vi "数据编码.vi"(0 "table输入":string(combo), 5 "错误常量 2":errorcluster caption="错误输入", 9 "QN":string, 13 "MN":string, 14 "PW":string) -> (4 "错误常量":errorcluster caption="错误输出", 8 "数据区":string, 15 "通讯包字符串":string)   [LabVIEW 2016]
uses:
  <vilib>/ptbypt/NI_PtbyPt.lvlib
panel:
  in  "时间戳 2":string
  in  "时间戳":string
  out "总包数":i32
  out "包数":i32=1024
  out "核查数据发送次数":i32
  out "当前包数":i32
  out "总包数":string
  out "小时数据发送次数":i32
  out "长度":i32
  in  "数据块":T1
  out "通讯包":T2={"包头（2）"="##", "数据段长度（4）"="", "数据段"="", "CRC校验"="", "包尾"=""}
  # "范例代码：\n\n##0101QN=20160801085857223;ST=32;CN=1062;PW=100000;MN=010000A8900016F000169DC0;Flag=5\n;CP=&&RtdInterval=30&&1C80\\r\\n"
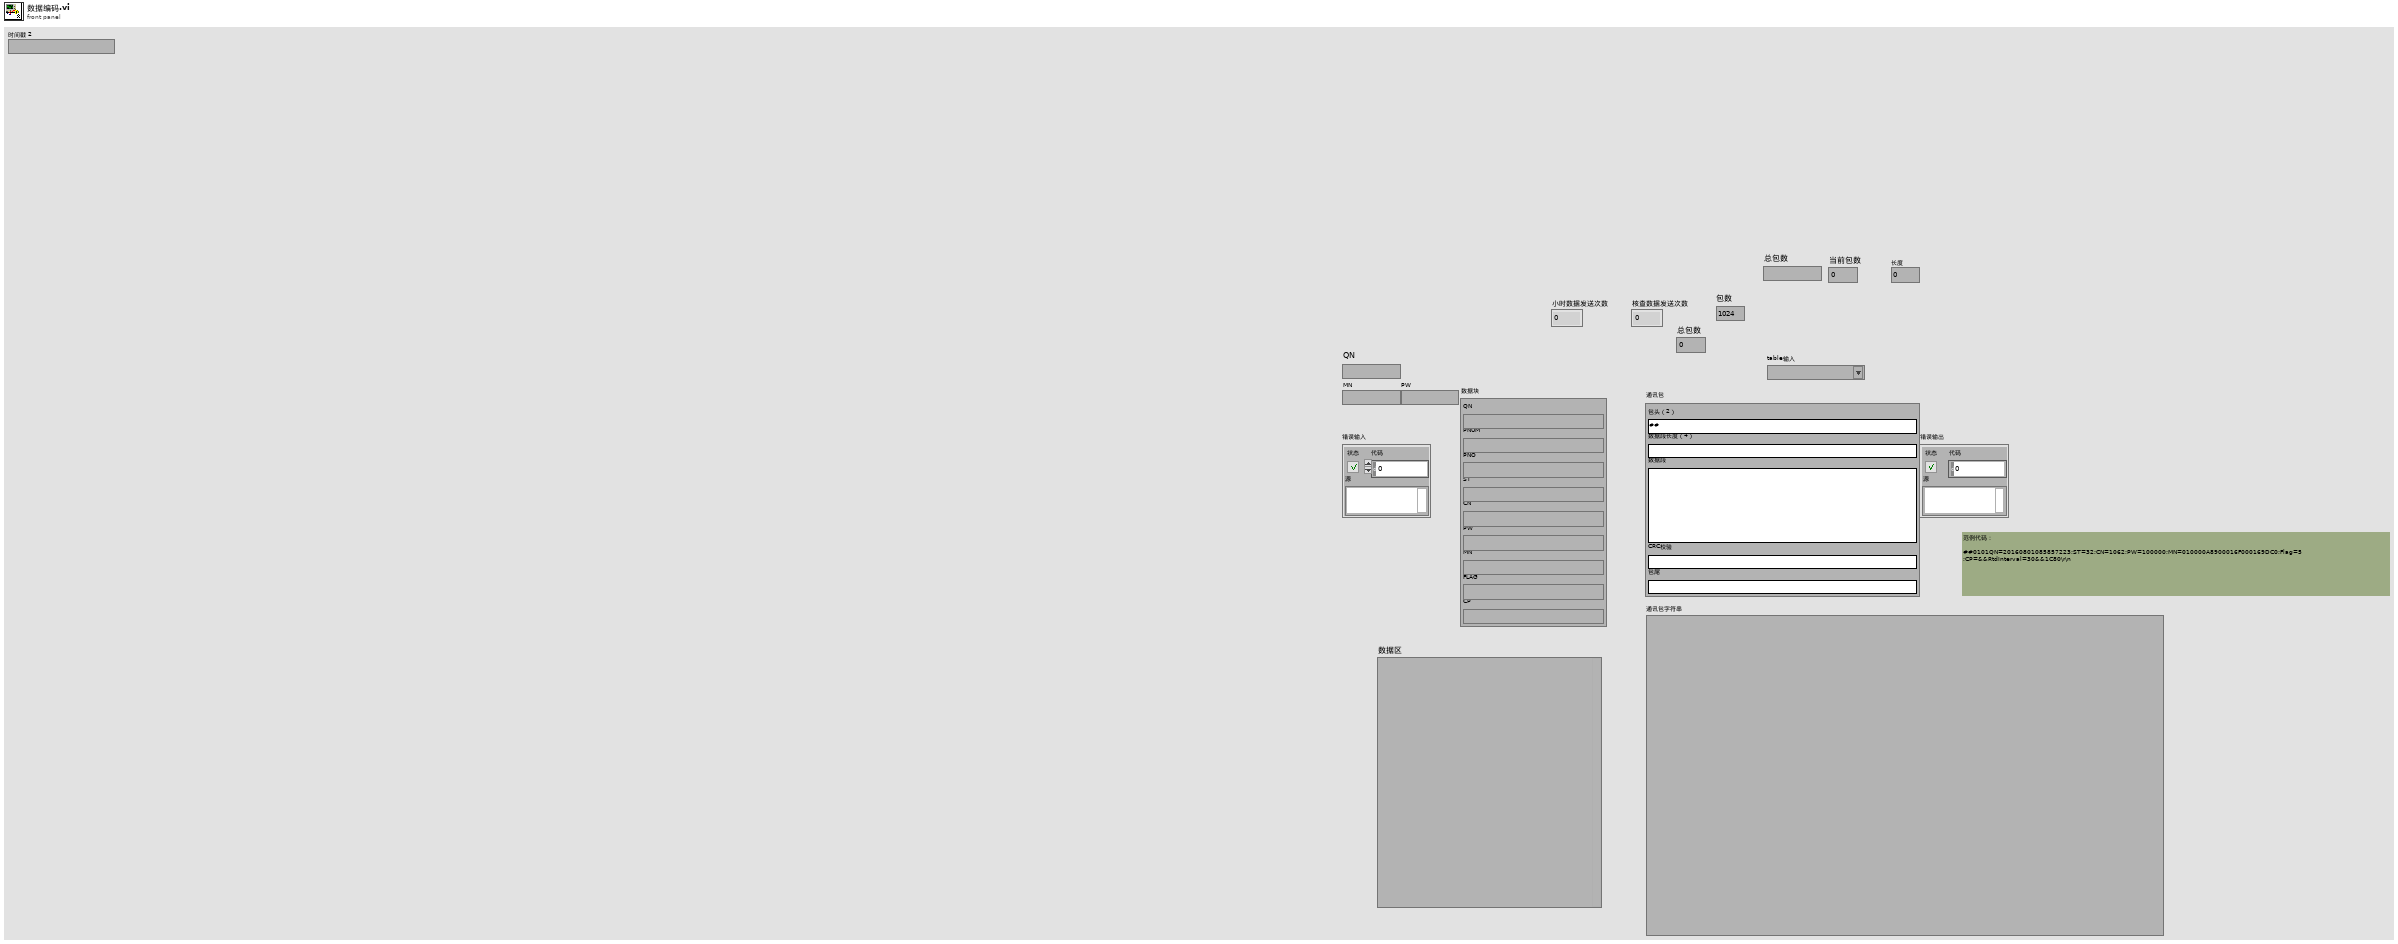
[diagram p1: front panel]
types:
  T1 = cluster{"QN":string, "ST":string, "CN":string, "PW":string, "MN":string, "FLAG":string, "PNUM":string, "PNO":string, "CP":string}
  T2 = cluster{"包头（2）":string, "数据段长度（4）":string, "数据段":string, "CRC校验":string, "包尾":string}
  T3 = cluster{"PH":string[][], "CODCr":string[][], "氨氮":string[][], "CODMn":string[][], "总氮":string[][], "总磷":string[][], "电导率":string[][], "水温":string[][], "DO":string[][], "浊度":string[][], "叶绿素":string[][], "藻密度":string[][]}
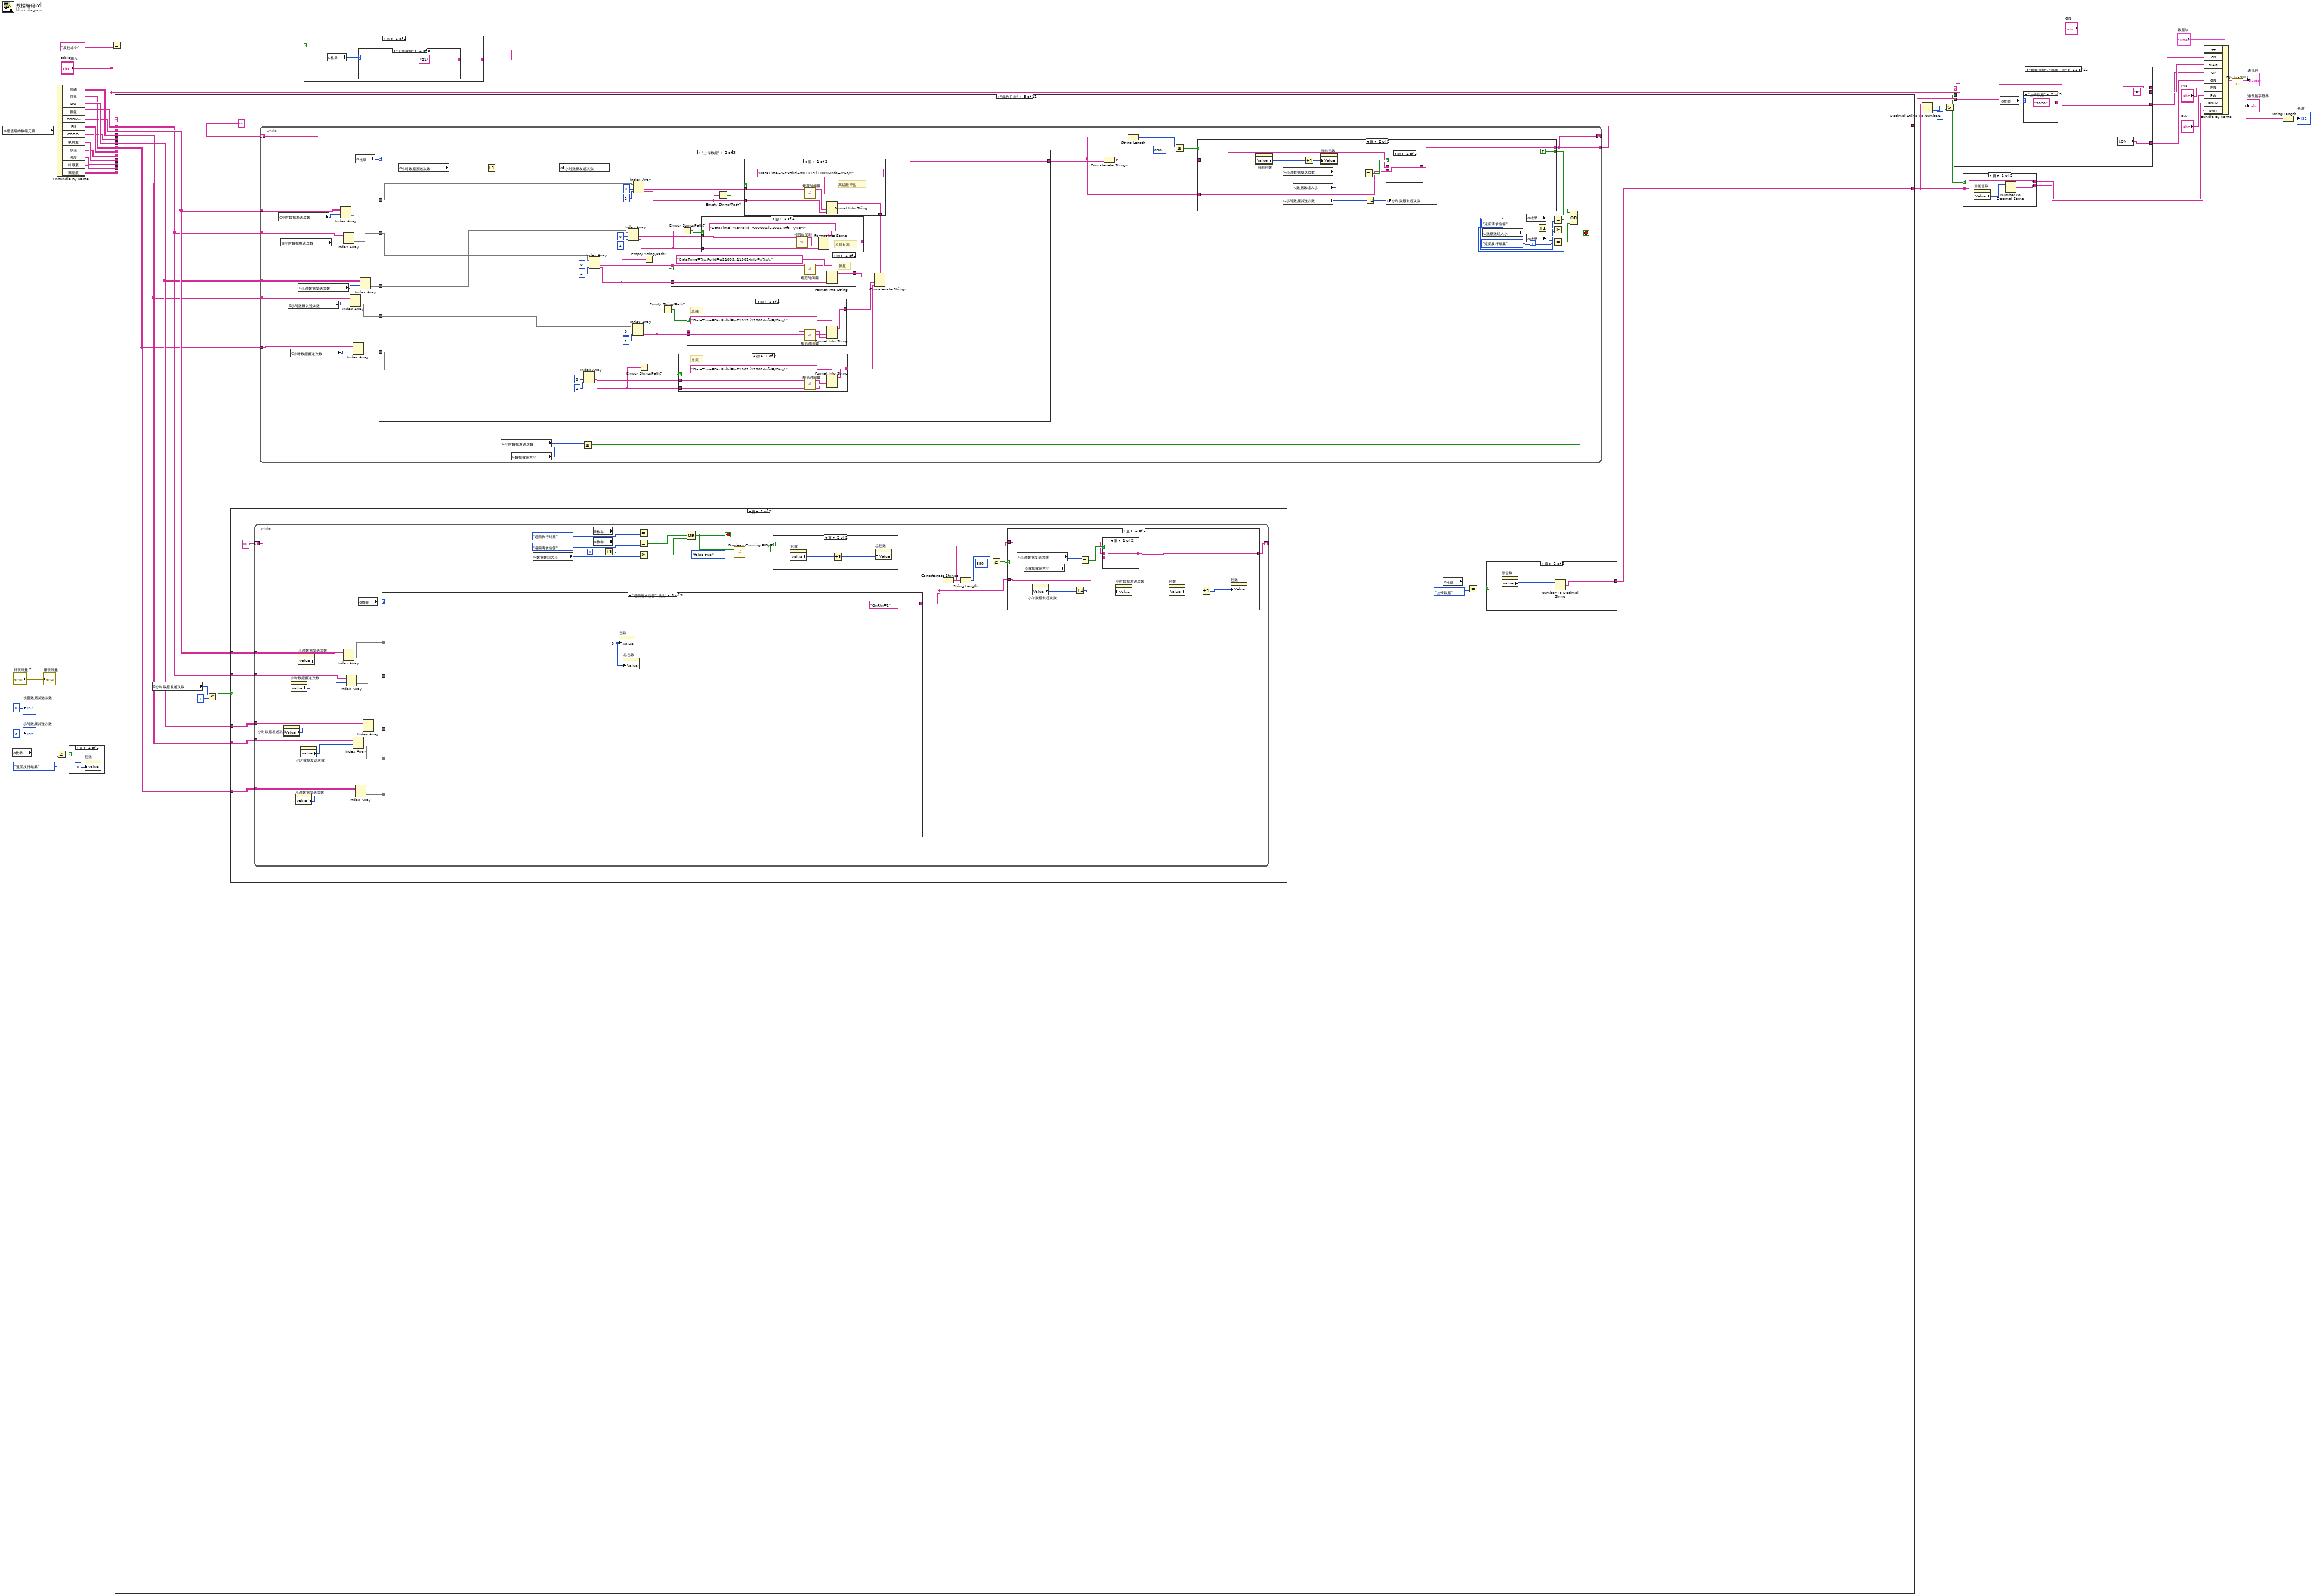
[diagram p0: block diagram]
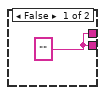
[diagram p3: hidden frame]
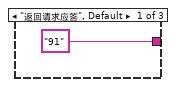
[diagram p4: hidden frame]
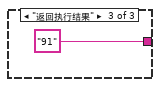
[diagram p5: hidden frame]
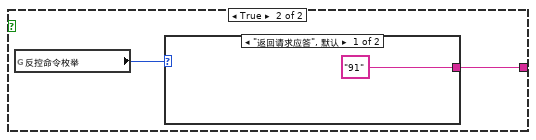
[diagram p6: hidden frame]
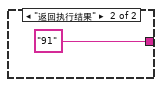
[diagram p7: hidden frame]
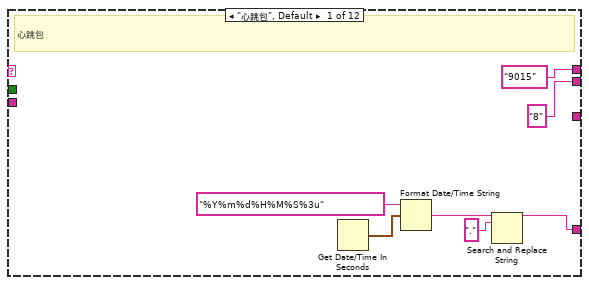
[diagram p8: hidden frame]
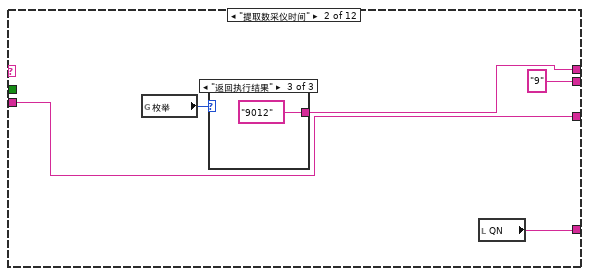
[diagram p9: hidden frame]
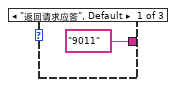
[diagram p10: hidden frame]
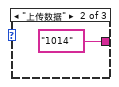
[diagram p11: hidden frame]
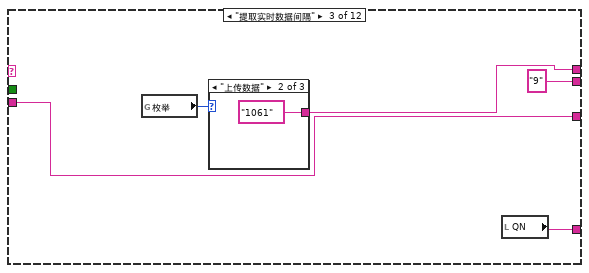
[diagram p12: hidden frame]
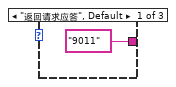
[diagram p13: hidden frame]
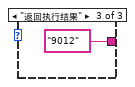
[diagram p14: hidden frame]
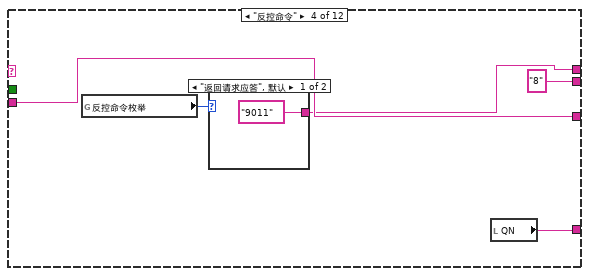
[diagram p15: hidden frame]
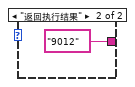
[diagram p16: hidden frame]
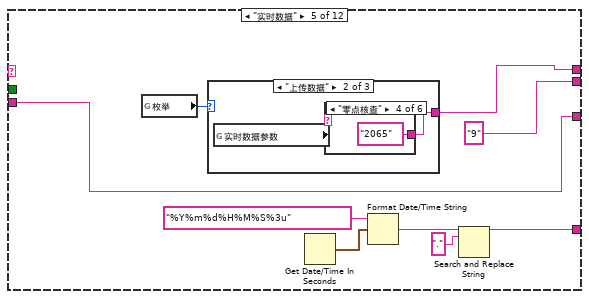
[diagram p17: hidden frame]
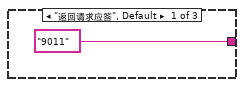
[diagram p18: hidden frame]
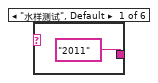
[diagram p19: hidden frame]
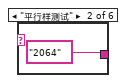
[diagram p20: hidden frame]
diagram:
  n1 = global read "插值后的新数组.vi" "插值后的数组元素"() -> (w9:T3)
  n2 = global read "全局1.vi" "枚举"() -> (w17:enum16{"返回请求应答", "上传数据", "返回执行结果"})
  n3 = Not Equal?(x=w17, y=enum16{"返回请求应答", "上传数据", "返回执行结果"}."返回执行结果") -> (x != y?=w15:bool)
  n4 = Unbundle By Name(w9) -> ("总磷"=w25:string[][], "总氮"=w24:string[][], "DO"=w26:string[][], "氨氮"=w27:string[][], "CODMn"=w8:string[][], "PH"=w12:string[][], "CODCr"=w11:string[][], "电导率"=w7:string[][], "水温"=w6:string[][], "浊度"=w5:string[][], "叶绿素"=w4:string[][], "藻密度"=w3:string[][])
  n5 = case shown="真" w15 {
    frame False {
    }
    frame True {
      n6 = property on="包数" class="DigNum (严格)"("Value"=0 ("总包数")) -> ()  [unwired: 2 in, 2 out]
    }
  }
  n7 = Equal?(x="table输入", y="反控命令") -> (x = y?=w29:bool)
  n8 = case shown="\"操作日志\"" "table输入" {
    tunnel: [w44 _ w48 w58 w67 w591 w985 w1448 w1880 w2166 w2437] -> w10
    tunnel: w8 -> [_ _ _ _ _ w589 w983 w1457 w1879 w2165 _]
    tunnel: w27 -> [_ _ _ _ _ w588 w982 w1456 w1878 w2164 _]
    tunnel: w26 -> [_ _ _ _ _ w587 w981 w1455 w1877 w2163 _]
    tunnel: w25 -> [_ _ _ _ _ w586 w980 w1454 w1876 w2162 _]
    tunnel: w24 -> [_ _ _ _ _ w585 w979 w1453 w1875 w2161 _]
    tunnel: [_ _ "" "" _ w558 w952 w1447 w1871 w2156 _] -> w14
    tunnel: w12 -> [_ _ _ _ _ w579 w973 w1445 _ _ _]
    tunnel: w11 -> [_ _ _ _ _ w578 w972 w1444 _ _ _]
    tunnel: w7 -> [_ _ _ _ _ w577 w971 _ _ _ _]
    tunnel: w6 -> [_ _ _ _ _ w576 w970 _ _ _ _]
    tunnel: w5 -> [_ _ _ _ _ w575 w969 _ _ _ _]
    tunnel: w4 -> [_ _ _ _ _ w574 w968 _ _ _ _]
    tunnel: w3 -> [_ _ _ _ _ w573 w967 _ _ _ _]
    frame "反控命令" {
      n9 = global read "全局 反控命令枚举.vi" "反控命令枚举"() -> (w43:enum16{"返回请求应答", "返回执行结果"})
      n10 = case shown="\"返回执行结果\"" w43 {
        tunnel: ["QnRtn=1" "ExeRtn=1"] -> w44
        frame "返回请求应答", Default {
        }
        frame "返回执行结果" {
        }
      }
    }
    frame "心跳包", Default {
    }
    frame "提取数采仪时间" {
      n11 = global read "全局1.vi" "枚举"() -> (w49:enum16{"返回请求应答", "上传数据", "返回执行结果"})
      n12 = case shown="\"上传数据\"" w49 {
        tunnel: ["QnRtn=1" w51 "ExeRtn=1"] -> w48
        frame "返回请求应答", Default {
        }
        frame "上传数据" {
          n13 = Get Date/Time In Seconds() -> (seconds since 1Jan1904=w55:timestamp)
          n14 = Format Date/Time String(time format string (%c)="%Y%m%d%H%M%S" ("时间格式字符串(%c)"), seconds (now)=w55) -> (date/time string=w52:string)  [unwired: 1 in]
          n15 = Concatenate Strings("SystemTime=", w52) -> (w51:string)
        }
        frame "返回执行结果" {
        }
      }
    }
    frame "提取实时数据间隔" {
      n16 = global read "全局1.vi" "枚举"() -> (w59:enum16{"返回请求应答", "上传数据", "返回执行结果"})
      n17 = case shown="\"上传数据\"" w59 {
        tunnel: ["QnRtn=1" w63 "ExeRtn=1"] -> w58
        frame "返回请求应答", Default {
        }
        frame "上传数据" {
          n18 = global read "实时数据发送间隔全局.vi" "实时数据发送间隔"() -> (w62:u32)
          n19 = Number To Decimal String(number=w62) -> (decimal integer string=w61:string)  [unwired: 1 in]
          n20 = Concatenate Strings("RtdInterval=", w61) -> (w63:string)
        }
        frame "返回执行结果" {
        }
      }
    }
    frame "实时数据" {
      n21 = global read "全局 实时数据参数.vi" "实时数据参数"() -> (w66:string)
      n22 = case shown="\"水样测试\", 默认" w66 {
        tunnel: [w68 w194 w321 w447] -> w67
        frame "水样测试", Default {
          n23 = global read "全局1.vi" "枚举"() -> (w69:enum16{"返回请求应答", "上传数据", "返回执行结果"})
          n24 = case shown="\"上传数据\"" w69 {
            tunnel: ["QnRtn=1" w75 "ExeRtn=1"] -> w68
            frame "返回请求应答", Default {
            }
            frame "上传数据" {
              n25 = control-ref of="时间戳"() -> (w73:refnum<vi>)
              n26 = Empty String/Path?(string/path="时间戳") -> (empty?=w72:bool)
              n27 = call "实时数据时间戳 (子VI).vi"("String输入"=w73) -> ()  [unwired: 11 in]
              n28 = Not(x=w72) -> (.not. x?=w71:bool)
              n29 = case shown="真" w71 {
                tunnel: ["" w190] -> w75
                tunnel: "时间戳" -> [_ w189]
                frame False {
                }
                frame True {
                  # "CODCr"
                  # "总氮"
                  # "总磷"
                  # "叶绿素"
                  # "叶绿素"
                  # "浊度"
                  # "电导率"
                  # "DO"
                  # "PH"
                  # "水温"
                  # "NH3"
                  # "CODMn"
                  n30 = global read "全局 所有参数.vi" "CODMn"() -> (w173:string[][])
                  n31 = global read "全局 所有参数.vi" "氨氮"() -> (w178:string[][])
                  n32 = global read "全局 所有参数.vi" "水温"() -> (w166:string[][])
                  n33 = global read "全局 所有参数.vi" "电导率"() -> (w138:string[][])
                  n34 = global read "全局 所有参数.vi" "DO"() -> (w148:string[][])
                  n35 = global read "全局 所有参数.vi" "PH"() -> (w156:string[][])
                  n36 = global read "全局 所有参数.vi" "藻密度"() -> (w111:string[][])
                  n37 = global read "全局 所有参数.vi" "浊度"() -> (w130:string[][])
                  n38 = global read "全局 所有参数.vi" "叶绿素"() -> (w121:string[][])
                  n39 = global read "全局 所有参数.vi" "CODCr"() -> (w83:string[][])
                  n40 = global read "全局 所有参数.vi" "总磷"() -> (w103:string[][])
                  n41 = global read "全局 所有参数.vi" "总氮"() -> (w91:string[][])
                  n42 = Index Array(array=w178, index (row)=0 ("索引 (行)")) -> (element=w176:string[])  [unwired: 1 in]
                  n43 = call "规范小时时间戳.vi"("字符串"=w189) -> ("result string"=w192:string)  [unwired: 10 in]
                  n44 = Index Array(array=w166, index (row)=0 ("索引 (行)")) -> (element=w168:string[])  [unwired: 1 in]
                  n45 = Index Array(array=w148, index (row)=0 ("索引 (行)")) -> (element=w150:string[])  [unwired: 1 in]
                  n46 = Index Array(array=w156, index (row)=0 ("索引 (行)")) -> (element=w154:string[])  [unwired: 1 in]
                  n47 = Index Array(array=w138, index (row)=0 ("索引 (行)")) -> (element=w136:string[])  [unwired: 1 in]
                  n48 = Index Array(array=w173, index (row)=0 ("索引 (行)")) -> (element=w171:string[])  [unwired: 1 in]
                  n49 = Index Array(array=w130, index (row)=0 ("索引 (行)")) -> (element=w132:string[])  [unwired: 1 in]
                  n50 = Index Array(array=w111, index (row)=0 ("索引 (行)")) -> (element=w109:string[])  [unwired: 1 in]
                  n51 = Index Array(array=w121, index (row)=0 ("索引 (行)")) -> (element=w123:string[])  [unwired: 1 in]
                  n52 = Index Array(array=w103, index (row)=0 ("索引 (行)")) -> (element=w105:string[])  [unwired: 1 in]
                  n53 = Index Array(array=w176, index=3 ("索引")) -> (element=w175:string)
                  n54 = Index Array(array=w91, index (row)=0 ("索引 (行)")) -> (element=w89:string[])  [unwired: 1 in]
                  n55 = Index Array(array=w83, index (row)=0 ("索引 (行)")) -> (element=w85:string[])  [unwired: 1 in]
                  n56 = Index Array(array=w168, index=3 ("索引")) -> (element=w169:string)
                  n57 = Index Array(array=w150, index=3 ("索引")) -> (element=w151:string)
                  n58 = Index Array(array=w154, index=3 ("索引")) -> (element=w153:string)
                  n59 = Index Array(array=w136, index=3 ("索引")) -> (element=w135:string)
                  n60 = Index Array(array=w132, index=3 ("索引")) -> (element=w133:string)
                  n61 = Index Array(array=w171, index=3 ("索引")) -> (element=w170:string)
                  n62 = Index Array(array=w109, index=3 ("索引")) -> (element=w108:string)
                  n63 = Index Array(array=w123, index=3 ("索引")) -> (element=w124:string)
                  n64 = Index Array(array=w105, index=3 ("索引")) -> (element=w106:string)
                  n65 = Index Array(array=w89, index=3 ("索引")) -> (element=w88:string)
                  n66 = Index Array(array=w85, index=3 ("索引")) -> (element=w86:string)
                  n67 = call "数据编码整合输出.vi"("数据标识"="N" ("字符串"), "数据类型"="-Rtd=", "污染物编码"="w21003", "数据精度"=3 ("精度"), "数据值"=w175) -> ("编码输出"=w180:string)  [unwired: 6 in]
                  n68 = call "数据编码整合输出.vi"("数据标识"="N" ("字符串"), "数据类型"="-Rtd=", "污染物编码"="w01010", "数据值"=w169) -> ("编码输出"=w161:string)  [unwired: 7 in]
                  n69 = call "数据编码整合输出.vi"("数据标识"="N" ("字符串"), "数据类型"="-Rtd=", "污染物编码"="w01009", "数据值"=w151) -> ("编码输出"=w143:string)  [unwired: 7 in]
                  n70 = call "数据编码整合输出.vi"("数据标识"="N" ("字符串"), "数据类型"="-Rtd=", "污染物编码"="w01001", "数据值"=w153) -> ("编码输出"=w152:string)  [unwired: 7 in]
                  n71 = call "数据编码整合输出.vi"("数据标识"="N" ("字符串"), "数据类型"="-Rtd=", "污染物编码"="w01014", "数据值"=w135) -> ("编码输出"=w134:string)  [unwired: 7 in]
                  n72 = call "数据编码整合输出.vi"("数据标识"="N" ("字符串"), "数据类型"="-Rtd=", "污染物编码"="w01014", "数据值"=w133) -> ("编码输出"=w125:string)  [unwired: 7 in]
                  n73 = call "数据编码整合输出.vi"("数据标识"="N" ("字符串"), "数据类型"="-Rtd=", "污染物编码"="w01019", "数据值"=w170) -> ("编码输出"=w185:string)  [unwired: 7 in]
                  n74 = call "数据编码整合输出.vi"("数据标识"="N" ("字符串"), "数据类型"="-Rtd=", "污染物编码"="w19011", "数据值"=w108) -> ("编码输出"=w107:string)  [unwired: 7 in]
                  n75 = call "数据编码整合输出.vi"("数据标识"="N" ("字符串"), "数据类型"="-Rtd=", "污染物编码"="w01016", "数据值"=w124) -> ("编码输出"=w116:string)  [unwired: 7 in]
                  n76 = call "数据编码整合输出.vi"("数据标识"="N" ("字符串"), "数据类型"="-Rtd=", "污染物编码"="w21011", "数据精度"=3 ("精度"), "数据值"=w106) -> ("编码输出"=w97:string)  [unwired: 6 in]
                  n77 = call "数据编码整合输出.vi"("数据标识"="N" ("字符串"), "数据类型"="-Rtd=", "污染物编码"="w21001", "数据精度"=3 ("精度"), "数据值"=w88) -> ("编码输出"=w87:string)  [unwired: 6 in]
                  n78 = call "数据编码整合输出.vi"("数据标识"="N" ("字符串"), "数据类型"="-Rtd=", "污染物编码"="w01018", "数据精度"=3 ("精度"), "数据值"=w86) -> ("编码输出"=w77:string)  [unwired: 6 in]
                  n79 = Format Into String(format string="DataTime=%s;%s%s%s%s%s%s%s%s%s%s%s%s" ("格式字符串"), w192, w185, w180, w161, w152, w143, w134, w125, w116, w107, w97, w87, w77) -> (resulting string=w190:string)  [unwired: 2 in, 1 out]
                }
              }
            }
            frame "返回执行结果" {
            }
          }
        }
        frame "平行样测试" {
          n80 = global read "全局1.vi" "枚举"() -> (w195:enum16{"返回请求应答", "上传数据", "返回执行结果"})
          n81 = case shown="\"上传数据\"" w195 {
            tunnel: ["QnRtn=1" w200 "ExeRtn=1"] -> w194
            frame "返回请求应答", Default {
            }
            frame "上传数据" {
              n82 = control-ref of="时间戳"() -> (w198:refnum<vi>)
              n83 = local read "时间戳"() -> (w199:string)
              n84 = call "实时数据时间戳 (子VI).vi"("String输入"=w198) -> ()  [unwired: 11 in]
              n85 = Empty String/Path?(string/path=w199) -> (empty?=w201:bool)
              n86 = Not(x=w201) -> (.not. x?=w197:bool)
              n87 = case shown="假" w197 {
                tunnel: ["" w316] -> w200
                tunnel: w199 -> [_ w203]
                frame False {
                }
                frame True {
                  # "CODCr"
                  # "总氮"
                  # "总磷"
                  # "叶绿素"
                  # "叶绿素"
                  # "浊度"
                  # "电导率"
                  # "DO"
                  # "PH"
                  # "水温"
                  # "NH3"
                  # "CODMn"
                  n88 = global read "全局 所有参数.vi" "CODMn"() -> (w300:string[][])
                  n89 = global read "全局 所有参数.vi" "氨氮"() -> (w305:string[][])
                  n90 = global read "全局 所有参数.vi" "水温"() -> (w293:string[][])
                  n91 = global read "全局 所有参数.vi" "电导率"() -> (w265:string[][])
                  n92 = global read "全局 所有参数.vi" "DO"() -> (w275:string[][])
                  n93 = global read "全局 所有参数.vi" "PH"() -> (w283:string[][])
                  n94 = global read "全局 所有参数.vi" "藻密度"() -> (w238:string[][])
                  n95 = global read "全局 所有参数.vi" "浊度"() -> (w257:string[][])
                  n96 = global read "全局 所有参数.vi" "叶绿素"() -> (w248:string[][])
                  n97 = global read "全局 所有参数.vi" "CODCr"() -> (w210:string[][])
                  n98 = global read "全局 所有参数.vi" "总磷"() -> (w230:string[][])
                  n99 = global read "全局 所有参数.vi" "总氮"() -> (w218:string[][])
                  n100 = Index Array(array=w305, index (row)=0 ("索引 (行)")) -> (element=w303:string[])  [unwired: 1 in]
                  n101 = Index Array(array=w293, index (row)=0 ("索引 (行)")) -> (element=w295:string[])  [unwired: 1 in]
                  n102 = Index Array(array=w275, index (row)=0 ("索引 (行)")) -> (element=w277:string[])  [unwired: 1 in]
                  n103 = Index Array(array=w283, index (row)=0 ("索引 (行)")) -> (element=w281:string[])  [unwired: 1 in]
                  n104 = Index Array(array=w265, index (row)=0 ("索引 (行)")) -> (element=w263:string[])  [unwired: 1 in]
                  n105 = Index Array(array=w300, index (row)=0 ("索引 (行)")) -> (element=w298:string[])  [unwired: 1 in]
                  n106 = call "规范小时时间戳.vi"("字符串"=w203) -> ("result string"=w318:string)  [unwired: 10 in]
                  n107 = Index Array(array=w257, index (row)=0 ("索引 (行)")) -> (element=w259:string[])  [unwired: 1 in]
                  n108 = Index Array(array=w238, index (row)=0 ("索引 (行)")) -> (element=w236:string[])  [unwired: 1 in]
                  n109 = Index Array(array=w248, index (row)=0 ("索引 (行)")) -> (element=w250:string[])  [unwired: 1 in]
                  n110 = Index Array(array=w230, index (row)=0 ("索引 (行)")) -> (element=w232:string[])  [unwired: 1 in]
                  n111 = Index Array(array=w303, index=3 ("索引")) -> (element=w302:string)
                  n112 = Index Array(array=w218, index (row)=0 ("索引 (行)")) -> (element=w216:string[])  [unwired: 1 in]
                  n113 = Index Array(array=w210, index (row)=0 ("索引 (行)")) -> (element=w212:string[])  [unwired: 1 in]
                  n114 = Index Array(array=w295, index=3 ("索引")) -> (element=w296:string)
                  n115 = Index Array(array=w277, index=3 ("索引")) -> (element=w278:string)
                  n116 = Index Array(array=w281, index=3 ("索引")) -> (element=w280:string)
                  n117 = Index Array(array=w263, index=3 ("索引")) -> (element=w262:string)
                  n118 = Index Array(array=w259, index=3 ("索引")) -> (element=w260:string)
                  n119 = Index Array(array=w298, index=3 ("索引")) -> (element=w297:string)
                  n120 = Index Array(array=w236, index=3 ("索引")) -> (element=w235:string)
                  n121 = Index Array(array=w250, index=3 ("索引")) -> (element=w251:string)
                  n122 = Index Array(array=w232, index=3 ("索引")) -> (element=w233:string)
                  n123 = Index Array(array=w216, index=3 ("索引")) -> (element=w215:string)
                  n124 = Index Array(array=w212, index=3 ("索引")) -> (element=w213:string)
                  n125 = call "数据编码整合输出.vi"("数据标识"="N" ("字符串"), "数据类型"="-Rtd=", "污染物编码"="w21003", "数据精度"=3 ("精度"), "数据值"=w302) -> ("编码输出"=w307:string)  [unwired: 6 in]
                  n126 = call "数据编码整合输出.vi"("数据标识"="N" ("字符串"), "数据类型"="-Rtd=", "污染物编码"="w01010", "数据值"=w296) -> ("编码输出"=w288:string)  [unwired: 7 in]
                  n127 = call "数据编码整合输出.vi"("数据标识"="N" ("字符串"), "数据类型"="-Rtd=", "污染物编码"="w01009", "数据值"=w278) -> ("编码输出"=w270:string)  [unwired: 7 in]
                  n128 = call "数据编码整合输出.vi"("数据标识"="N" ("字符串"), "数据类型"="-Rtd=", "污染物编码"="w01001", "数据值"=w280) -> ("编码输出"=w279:string)  [unwired: 7 in]
                  n129 = call "数据编码整合输出.vi"("数据标识"="N" ("字符串"), "数据类型"="-Rtd=", "污染物编码"="w01014", "数据值"=w262) -> ("编码输出"=w261:string)  [unwired: 7 in]
                  n130 = call "数据编码整合输出.vi"("数据标识"="N" ("字符串"), "数据类型"="-Rtd=", "污染物编码"="w01014", "数据值"=w260) -> ("编码输出"=w252:string)  [unwired: 7 in]
                  n131 = call "数据编码整合输出.vi"("数据标识"="N" ("字符串"), "数据类型"="-Rtd=", "污染物编码"="w01019", "数据值"=w297) -> ("编码输出"=w312:string)  [unwired: 7 in]
                  n132 = call "数据编码整合输出.vi"("数据标识"="N" ("字符串"), "数据类型"="-Rtd=", "污染物编码"="w19011", "数据值"=w235) -> ("编码输出"=w234:string)  [unwired: 7 in]
                  n133 = call "数据编码整合输出.vi"("数据标识"="N" ("字符串"), "数据类型"="-Rtd=", "污染物编码"="w01016", "数据值"=w251) -> ("编码输出"=w243:string)  [unwired: 7 in]
                  n134 = call "数据编码整合输出.vi"("数据标识"="N" ("字符串"), "数据类型"="-Rtd=", "污染物编码"="w21011", "数据精度"=3 ("精度"), "数据值"=w233) -> ("编码输出"=w224:string)  [unwired: 6 in]
                  n135 = call "数据编码整合输出.vi"("数据标识"="N" ("字符串"), "数据类型"="-Rtd=", "污染物编码"="w21001", "数据精度"=3 ("精度"), "数据值"=w215) -> ("编码输出"=w214:string)  [unwired: 6 in]
                  n136 = call "数据编码整合输出.vi"("数据标识"="N" ("字符串"), "数据类型"="-Rtd=", "污染物编码"="w01018", "数据精度"=3 ("精度"), "数据值"=w213) -> ("编码输出"=w204:string)  [unwired: 6 in]
                  n137 = Format Into String(format string="DataTime=%s;%s%s%s%s%s%s%s%s%s%s%s%s" ("格式字符串"), w318, w312, w307, w288, w279, w270, w261, w252, w243, w234, w224, w214, w204) -> (resulting string=w316:string)  [unwired: 2 in, 1 out]
                }
              }
            }
            frame "返回执行结果" {
            }
          }
        }
        frame "加标回收测试" {
          n138 = global read "全局1.vi" "枚举"() -> (w320:enum16{"返回请求应答", "上传数据", "返回执行结果"})
          n139 = case shown="\"上传数据\"" w320 {
            tunnel: ["QnRtn=1" w326 "ExeRtn=1"] -> w321
            frame "返回请求应答", Default {
            }
            frame "上传数据" {
              n140 = control-ref of="时间戳"() -> (w325:refnum<vi>)
              n141 = local read "时间戳"() -> (w324:string)
              n142 = Empty String/Path?(string/path=w324) -> (empty?=w327:bool)
              n143 = call "实时数据时间戳 (子VI).vi"("String输入"=w325) -> ()  [unwired: 11 in]
              n144 = Not(x=w327) -> (.not. x?=w323:bool)
              n145 = case shown="真" w323 {
                tunnel: ["" w442] -> w326
                tunnel: w324 -> [_ w329]
                frame False {
                }
                frame True {
                  # "CODCr"
                  # "总氮"
                  # "总磷"
                  # "叶绿素"
                  # "叶绿素"
                  # "浊度"
                  # "电导率"
                  # "DO"
                  # "PH"
                  # "水温"
                  # "NH3"
                  # "CODMn"
                  n146 = global read "全局 所有参数.vi" "CODMn"() -> (w426:string[][])
                  n147 = global read "全局 所有参数.vi" "氨氮"() -> (w431:string[][])
                  n148 = global read "全局 所有参数.vi" "水温"() -> (w419:string[][])
                  n149 = global read "全局 所有参数.vi" "电导率"() -> (w391:string[][])
                  n150 = global read "全局 所有参数.vi" "DO"() -> (w401:string[][])
                  n151 = global read "全局 所有参数.vi" "PH"() -> (w409:string[][])
                  n152 = global read "全局 所有参数.vi" "藻密度"() -> (w364:string[][])
                  n153 = global read "全局 所有参数.vi" "浊度"() -> (w383:string[][])
                  n154 = global read "全局 所有参数.vi" "叶绿素"() -> (w374:string[][])
                  n155 = global read "全局 所有参数.vi" "CODCr"() -> (w336:string[][])
                  n156 = global read "全局 所有参数.vi" "总磷"() -> (w356:string[][])
                  n157 = global read "全局 所有参数.vi" "总氮"() -> (w344:string[][])
                  n158 = Index Array(array=w431, index (row)=0 ("索引 (行)")) -> (element=w429:string[])  [unwired: 1 in]
                  n159 = Index Array(array=w419, index (row)=0 ("索引 (行)")) -> (element=w421:string[])  [unwired: 1 in]
                  n160 = Index Array(array=w401, index (row)=0 ("索引 (行)")) -> (element=w403:string[])  [unwired: 1 in]
                  n161 = Index Array(array=w409, index (row)=0 ("索引 (行)")) -> (element=w407:string[])  [unwired: 1 in]
                  n162 = Index Array(array=w391, index (row)=0 ("索引 (行)")) -> (element=w389:string[])  [unwired: 1 in]
                  n163 = Index Array(array=w426, index (row)=0 ("索引 (行)")) -> (element=w424:string[])  [unwired: 1 in]
                  n164 = Index Array(array=w383, index (row)=0 ("索引 (行)")) -> (element=w385:string[])  [unwired: 1 in]
                  n165 = Index Array(array=w364, index (row)=0 ("索引 (行)")) -> (element=w362:string[])  [unwired: 1 in]
                  n166 = Index Array(array=w374, index (row)=0 ("索引 (行)")) -> (element=w376:string[])  [unwired: 1 in]
                  n167 = Index Array(array=w356, index (row)=0 ("索引 (行)")) -> (element=w358:string[])  [unwired: 1 in]
                  n168 = Index Array(array=w429, index=3 ("索引")) -> (element=w428:string)
                  n169 = call "规范小时时间戳.vi"("字符串"=w329) -> ("result string"=w444:string)  [unwired: 10 in]
                  n170 = Index Array(array=w344, index (row)=0 ("索引 (行)")) -> (element=w342:string[])  [unwired: 1 in]
                  n171 = Index Array(array=w336, index (row)=0 ("索引 (行)")) -> (element=w338:string[])  [unwired: 1 in]
                  n172 = Index Array(array=w421, index=3 ("索引")) -> (element=w422:string)
                  n173 = Index Array(array=w403, index=3 ("索引")) -> (element=w404:string)
                  n174 = Index Array(array=w407, index=3 ("索引")) -> (element=w406:string)
                  n175 = Index Array(array=w389, index=3 ("索引")) -> (element=w388:string)
                  n176 = Index Array(array=w385, index=3 ("索引")) -> (element=w386:string)
                  n177 = Index Array(array=w424, index=3 ("索引")) -> (element=w423:string)
                  n178 = Index Array(array=w362, index=3 ("索引")) -> (element=w361:string)
                  n179 = Index Array(array=w376, index=3 ("索引")) -> (element=w377:string)
                  n180 = Index Array(array=w358, index=3 ("索引")) -> (element=w359:string)
                  n181 = Index Array(array=w342, index=3 ("索引")) -> (element=w341:string)
                  n182 = Index Array(array=w338, index=3 ("索引")) -> (element=w339:string)
                  n183 = call "数据编码整合输出.vi"("数据标识"="N" ("字符串"), "数据类型"="-Rtd=", "污染物编码"="w21003", "数据精度"=3 ("精度"), "数据值"=w428) -> ("编码输出"=w433:string)  [unwired: 6 in]
                  n184 = call "数据编码整合输出.vi"("数据标识"="N" ("字符串"), "数据类型"="-Rtd=", "污染物编码"="w01010", "数据值"=w422) -> ("编码输出"=w414:string)  [unwired: 7 in]
                  n185 = call "数据编码整合输出.vi"("数据标识"="N" ("字符串"), "数据类型"="-Rtd=", "污染物编码"="w01009", "数据值"=w404) -> ("编码输出"=w396:string)  [unwired: 7 in]
                  n186 = call "数据编码整合输出.vi"("数据标识"="N" ("字符串"), "数据类型"="-Rtd=", "污染物编码"="w01001", "数据值"=w406) -> ("编码输出"=w405:string)  [unwired: 7 in]
                  n187 = call "数据编码整合输出.vi"("数据标识"="N" ("字符串"), "数据类型"="-Rtd=", "污染物编码"="w01014", "数据值"=w388) -> ("编码输出"=w387:string)  [unwired: 7 in]
                  n188 = call "数据编码整合输出.vi"("数据标识"="N" ("字符串"), "数据类型"="-Rtd=", "污染物编码"="w01014", "数据值"=w386) -> ("编码输出"=w378:string)  [unwired: 7 in]
                  n189 = call "数据编码整合输出.vi"("数据标识"="N" ("字符串"), "数据类型"="-Rtd=", "污染物编码"="w01019", "数据值"=w423) -> ("编码输出"=w438:string)  [unwired: 7 in]
                  n190 = call "数据编码整合输出.vi"("数据标识"="N" ("字符串"), "数据类型"="-Rtd=", "污染物编码"="w19011", "数据值"=w361) -> ("编码输出"=w360:string)  [unwired: 7 in]
                  n191 = call "数据编码整合输出.vi"("数据标识"="N" ("字符串"), "数据类型"="-Rtd=", "污染物编码"="w01016", "数据值"=w377) -> ("编码输出"=w369:string)  [unwired: 7 in]
                  n192 = call "数据编码整合输出.vi"("数据标识"="N" ("字符串"), "数据类型"="-Rtd=", "污染物编码"="w21011", "数据精度"=3 ("精度"), "数据值"=w359) -> ("编码输出"=w350:string)  [unwired: 6 in]
                  n193 = call "数据编码整合输出.vi"("数据标识"="N" ("字符串"), "数据类型"="-Rtd=", "污染物编码"="w21001", "数据精度"=3 ("精度"), "数据值"=w341) -> ("编码输出"=w340:string)  [unwired: 6 in]
                  n194 = call "数据编码整合输出.vi"("数据标识"="N" ("字符串"), "数据类型"="-Rtd=", "污染物编码"="w01018", "数据精度"=3 ("精度"), "数据值"=w339) -> ("编码输出"=w330:string)  [unwired: 6 in]
                  n195 = Format Into String(format string="DataTime=%s;%s%s%s%s%s%s%s%s%s%s%s%s" ("格式字符串"), w444, w438, w433, w414, w405, w396, w387, w378, w369, w360, w350, w340, w330) -> (resulting string=w442:string)  [unwired: 2 in, 1 out]
                }
              }
            }
            frame "返回执行结果" {
            }
          }
        }
        frame "跨度核查", "零点核查" {
          n196 = global read "全局1.vi" "枚举"() -> (w446:enum16{"返回请求应答", "上传数据", "返回执行结果"})
          n197 = case shown="\"上传数据\"" w446 {
            tunnel: ["QnRtn=1" w452 "ExeRtn=1"] -> w447
            frame "返回请求应答", Default {
            }
            frame "上传数据" {
              n198 = control-ref of="时间戳"() -> (w450:refnum<vi>)
              n199 = local read "时间戳"() -> (w451:string)
              n200 = call "实时数据时间戳 (子VI).vi"("String输入"=w450) -> ()  [unwired: 11 in]
              n201 = Empty String/Path?(string/path=w451) -> (empty?=w453:bool)
              n202 = Not(x=w453) -> (.not. x?=w449:bool)
              n203 = case shown="假" w449 {
                tunnel: ["" w554] -> w452
                tunnel: w451 -> [_ w533]
                frame False {
                }
                frame True {
                  # "CODCr"
                  # "总氮"
                  # "总磷"
                  # "NH3"
                  # "CODMn"
                  n204 = global read "全局 所有参数.vi" "CODMn"() -> (w548:string[][])
                  n205 = global read "全局 所有参数.vi" "氨氮"() -> (w552:string[][])
                  n206 = global read "全局 所有参数.vi" "总磷"() -> (w543:string[][])
                  n207 = global read "全局 所有参数.vi" "总氮"() -> (w540:string[][])
                  n208 = global read "全局 所有参数.vi" "CODCr"() -> (w535:string[][])
                  n209 = Index Array(array=w552, index (row)=0 ("索引 (行)")) -> (element=w550:string[])  [unwired: 1 in]
                  n210 = Index Array(array=w548, index (row)=0 ("索引 (行)")) -> (element=w546:string[])  [unwired: 1 in]
                  n211 = Index Array(array=w543, index (row)=0 ("索引 (行)")) -> (element=w545:string[])  [unwired: 1 in]
                  n212 = Index Array(array=w540, index (row)=0 ("索引 (行)")) -> (element=w538:string[])  [unwired: 1 in]
                  n213 = Index Array(array=w535, index (row)=0 ("索引 (行)")) -> (element=w537:string[])  [unwired: 1 in]
                  n214 = Index Array(array=w550, index #1=3 ("索引"), index #2=7 ("索引")) -> (element #1=w508:string, element #2=w506:string)
                  n215 = call "规范小时时间戳.vi"("字符串"=w533) -> ("result string"=w556:string)  [unwired: 10 in]
                  n216 = Index Array(array=w546, index #1=3 ("索引"), index #2=7 ("索引")) -> (element #1=w530:string, element #2=w520:string)
                  n217 = Index Array(array=w545, index #1=3 ("索引"), index #2=7 ("索引")) -> (element #1=w490:string, element #2=w488:string)
                  n218 = Index Array(array=w538, index #1=3 ("索引"), index #2=7 ("索引")) -> (element #1=w475:string, element #2=w473:string)
                  n219 = Index Array(array=w537, index #1=3 ("索引"), index #2=7 ("索引")) -> (element #1=w460:string, element #2=w458:string)
                  n220 = call "核查数据编码整合输出.vi"("字段结束"=FALSE, "数据标识"="N" ("字符串"), "数据类型"="-Check=", "污染物编码"="w01019", "数据值"=w530) -> ("编码输出"=w526:string)  [unwired: 6 in]
                  n221 = call "核查数据编码整合输出.vi"("字段结束"=FALSE, "数据标识"="N" ("字符串"), "数据类型"="-Check=", "污染物编码"="w21003", "数据精度"=3 ("精度"), "数据值"=w508) -> ("编码输出"=w504:string)  [unwired: 5 in]
                  n222 = call "核查数据编码整合输出.vi"("字段结束"=TRUE, "数据标识"="N" ("字符串"), "数据类型"="-StandardValue=", "污染物编码"="w01019", "数据值"=w520) -> ("编码输出"=w519:string)  [unwired: 6 in]
                  n223 = call "核查数据编码整合输出.vi"("字段结束"=TRUE, "数据标识"="N" ("字符串"), "数据类型"="-StandardValue=", "污染物编码"="w21001", "数据精度"=3 ("精度"), "数据值"=w473) -> ("编码输出"=w477:string)  [unwired: 5 in]
                  n224 = call "核查数据编码整合输出.vi"("字段结束"=TRUE, "数据标识"="N" ("字符串"), "数据类型"="-StandardValue=", "污染物编码"="w21011", "数据精度"=3 ("精度"), "数据值"=w488) -> ("编码输出"=w501:string)  [unwired: 5 in]
                  n225 = call "核查数据编码整合输出.vi"("字段结束"=TRUE, "数据标识"="N" ("字符串"), "数据类型"="-StandardValue=", "污染物编码"="w21003", "数据精度"=3 ("精度"), "数据值"=w506) -> ("编码输出"=w505:string)  [unwired: 5 in]
                  n226 = call "核查数据编码整合输出.vi"("字段结束"=FALSE, "数据标识"="N" ("字符串"), "数据类型"="-Check=", "污染物编码"="w21001", "数据精度"=3 ("精度"), "数据值"=w475) -> ("编码输出"=w476:string)  [unwired: 5 in]
                  n227 = call "核查数据编码整合输出.vi"("字段结束"=FALSE, "数据标识"="N" ("字符串"), "数据类型"="-Check=", "污染物编码"="w21011", "数据精度"=3 ("精度"), "数据值"=w490) -> ("编码输出"=w502:string)  [unwired: 5 in]
                  n228 = call "核查数据编码整合输出.vi"("字段结束"=TRUE, "数据标识"="N" ("字符串"), "数据类型"="-StandardValue=", "污染物编码"="w01018", "数据精度"=3 ("精度"), "数据值"=w458) -> ("编码输出"=w471:string)  [unwired: 5 in]
                  n229 = call "核查数据编码整合输出.vi"("字段结束"=FALSE, "数据标识"="N" ("字符串"), "数据类型"="-Check=", "污染物编码"="w01018", "数据精度"=3 ("精度"), "数据值"=w460) -> ("编码输出"=w472:string)  [unwired: 5 in]
                  n230 = Concatenate Strings(w504, w505) -> (w503:string)
                  n231 = Concatenate Strings(w526, w519) -> (w525:string)
                  n232 = Concatenate Strings(w476, w477) -> (w456:string)
                  n233 = Concatenate Strings(w502, w501) -> (w457:string)
                  n234 = Concatenate Strings(w472, w471) -> (w455:string)
                  n235 = Format Into String(format string="DataTime=%s;%s%s%s%s%s" ("格式字符串"), w556, w525, w503, w457, w456, w455) -> (resulting string=w554:string)  [unwired: 2 in, 1 out]
                }
              }
            }
            frame "返回执行结果" {
            }
          }
        }
      }
    }
    frame "小时数据" {
      # "发送小时数据"
      n236 = global read "插值后的新数组.vi" "插值后的数组元素"() -> (w572:T3)
      n237 = while {
        tunnel: w589 -> [w818]
        tunnel: w588 -> [w814]
        tunnel: w587 -> [w812]
        tunnel: w586 -> [w809]
        tunnel: w585 -> [w806]
        tunnel: [w791] -> w591
        shift-right: [w791] -> _
        shift-left: "" -> [w792]
        tunnel: w579 -> [w787]
        tunnel: w578 -> [w783]
        tunnel: w577 -> [w781]
        tunnel: w576 -> [w778]
        tunnel: w575 -> [w774]
        tunnel: w574 -> [w771]
        tunnel: w573 -> [w770]
        i -> [w821]
        stop <- w799 stop-if-true
        # "藻密度"
        # "叶绿素"
        # "浊度"
        # "水温"
        n238 = global read "全局 小时数据发送次数.vi" "小时数据发送次数"() -> (w782:i32)
        n239 = global read "全局 小时数据发送次数.vi" "小时数据发送次数"() -> (w784:i32)
        n240 = global read "全局 小时数据发送次数.vi" "小时数据发送次数"() -> (w788:i32)
        n241 = global read "全局 小时数据发送次数.vi" "小时数据发送次数"() -> (w813:i32)
        n242 = global read "全局 小时数据发送次数.vi" "小时数据发送次数"() -> (w776:i32)
        n243 = global read "全局 小时数据发送次数.vi" "小时数据发送次数"() -> (w810:i32)
        n244 = global read "全局 小时数据发送次数.vi" "小时数据发送次数"() -> (w819:i32)
        n245 = global read "全局 小时数据发送次数.vi" "小时数据发送次数"() -> (w772:i32)
        n246 = global read "全局 小时数据发送次数.vi" "小时数据发送次数"() -> (w816:i32)
        n247 = global read "全局 小时数据发送次数.vi" "小时数据发送次数"() -> (w779:i32)
        n248 = global read "全局 小时数据发送次数.vi" "小时数据发送次数"() -> (w807:i32)
        n249 = global read "全局 小时数据发送次数.vi" "小时数据发送次数"() -> (w773:i32)
        n250 = Index Array(array=w783, index (row)=w784) -> (element=w785:string[])  [unwired: 1 in]
        n251 = Index Array(array=w787, index (row)=w788) -> (element=w786:string[])  [unwired: 1 in]
        n252 = Index Array(array=w814, index (row)=w816) -> (element=w815:string[])  [unwired: 1 in]
        n253 = Index Array(array=w812, index (row)=w813) -> (element=w811:string[])  [unwired: 1 in]
        n254 = Index Array(array=w809, index (row)=w810) -> (element=w808:string[])  [unwired: 1 in]
        n255 = Index Array(array=w818, index (row)=w819) -> (element=w817:string[])  [unwired: 1 in]
        n256 = Index Array(array=w781, index (row)=w782) -> (element=w780:string[])  [unwired: 1 in]
        n257 = Index Array(array=w774, index (row)=w776) -> (element=w775:string[])  [unwired: 1 in]
        n258 = Index Array(array=w778, index (row)=w779) -> (element=w777:string[])  [unwired: 1 in]
        n259 = Index Array(array=w806, index (row)=w807) -> (element=w805:string[])  [unwired: 1 in]
        n260 = Index Array(array=w770, index (row)=w772) -> (element=w768:string[])  [unwired: 1 in]
        n261 = Index Array(array=w771, index (row)=w773) -> (element=w769:string[])  [unwired: 1 in]
        n262 = global read "全局1.vi" "枚举"() -> (w822:enum16{"返回请求应答", "上传数据", "返回执行结果"})
        n263 = case shown="\"返回执行结果\"" w822 {
          tunnel: ["QnRtn=1" w853 "ExeRtn=1"] -> w798
          tunnel: w817 -> [_ w925 _]
          tunnel: w811 -> [_ w942 _]
          tunnel: w808 -> [_ w941 _]
          tunnel: w805 -> [_ w940 _]
          tunnel: w815 -> [_ w938 _]
          tunnel: w786 -> [_ w924 _]
          tunnel: w785 -> [_ w930 _]
          tunnel: w780 -> [_ w927 _]
          tunnel: w777 -> [_ w926 _]
          tunnel: w775 -> [_ w923 _]
          tunnel: w769 -> [_ w922 _]
          tunnel: w768 -> [_ w921 _]
          frame "返回请求应答", Default {
            w844 = 0 ("当前包数")
            n264 = property on="当前包数" class="DigNum (严格)"("Value"=w844) -> ()  [unwired: 2 in, 2 out]
            n265 = property on="总包数" class="DigNum (严格)"("Value"=w844) -> ()  [unwired: 2 in, 2 out]
            n266 = global read "全局 数据数组大小.vi" "数据数组大小"() -> (w845:i32)
            n267 = global write "全局1.vi" "枚举"(enum16{"返回请求应答", "上传数据", "返回执行结果"}."上传数据" ("枚举")) -> ()
            n268 = Equal To 0?(x=w845) -> (x = 0?=w846:bool)
            n269 = case shown="真" w846 {
              frame False {
              }
              frame True {
                n270 = global read "全局 小时数据发送次数.vi" "小时数据发送次数"() -> (w850:i32)
                n271 = Increment(x=w850) -> (x+1=w849:i32)
                n272 = global write "全局 小时数据发送次数.vi" "小时数据发送次数"(w849) -> ()
              }
            }
          }
          frame "上传数据" {
            # "PH"
            # "总氮"
            # "总磷"
            # "藻密度"
            # "叶绿素"
            # "浊度"
            # "电导率"
            # "DO"
            # "CODCr"
            # "水温"
            # "NH3"
            # "CODMn"
            n273 = Index Array(array=w922) -> (element #2=w879:string)  [unwired: 2 in, 1 out]
            n274 = Index Array(array=w927) -> (element #2=w888:string)  [unwired: 2 in, 1 out]
            n275 = Index Array(array=w923) -> (element #2=w884:string)  [unwired: 2 in, 1 out]
            n276 = Index Array(array=w921) -> (element #2=w874:string)  [unwired: 2 in, 1 out]
            n277 = Index Array(array=w926) -> (element #2=w906:string)  [unwired: 2 in, 1 out]
            n278 = Index Array(array=w942, index #1=0 ("索引")) -> (element #2=w895:string)  [unwired: 1 in, 1 out]
            n279 = Index Array(array=w925, index #1=0 ("索引"), index #2=1 ("索引")) -> (element #1=w893:string, element #2=w920:string)
            n280 = Index Array(array=w924) -> (element #2=w856:string)  [unwired: 2 in, 1 out]
            n281 = Index Array(array=w938, index #1=0 ("索引"), index #2=1 ("索引")) -> (element #2=w912:string)  [unwired: 1 out]
            n282 = Index Array(array=w930, index #1=0 ("索引"), index #2=1 ("索引")) -> (element #2=w900:string)  [unwired: 1 out]
            n283 = Index Array(array=w941, index #1=0 ("索引"), index #2=1 ("索引")) -> (element #2=w869:string)  [unwired: 1 out]
            n284 = Index Array(array=w940, index #1=0 ("索引"), index #2=1 ("索引")) -> (element #2=w864:string)  [unwired: 1 out]
            n285 = global read "全局 小时数据发送次数.vi" "小时数据发送次数"() -> (w937:i32)
            n286 = call "规范小时时间戳.vi"("字符串"=w893) -> ("result string"=w852:string)  [unwired: 10 in]
            n287 = Increment(x=w937) -> (x+1=w936:i32)
            n288 = global write "全局 小时数据发送次数.vi" "小时数据发送次数"(w936) -> ()
            n289 = call "数据编码整合输出.vi"("数据标识"="N" ("字符串"), "数据类型"="-Avg=", "污染物编码"="w01019", "数据值"=w920) -> ("编码输出"=w919:string)  [unwired: 7 in]
            n290 = call "数据编码整合输出.vi"("数据标识"="N" ("字符串"), "数据类型"="-Avg=", "污染物编码"="w01010", "数据值"=w906) -> ("编码输出"=w905:string)  [unwired: 7 in]
            n291 = call "数据编码整合输出.vi"("数据标识"="N" ("字符串"), "数据类型"="-Avg=", "污染物编码"="w01018", "数据精度"=3, "数据值"=w900) -> ("编码输出"=w899:string)  [unwired: 6 in]
            n292 = call "数据编码整合输出.vi"("数据标识"="N" ("字符串"), "数据类型"="-Avg=", "污染物编码"="w21003", "数据精度"=3, "数据值"=w912) -> ("编码输出"=w911:string)  [unwired: 6 in]
            n293 = call "数据编码整合输出.vi"("数据标识"="N" ("字符串"), "数据类型"="-Avg=", "污染物编码"="w21001", "数据精度"=3, "数据值"=w864) -> ("编码输出"=w863:string)  [unwired: 6 in]
            n294 = call "数据编码整合输出.vi"("数据标识"="N" ("字符串"), "数据类型"="-Avg=", "污染物编码"="w01001", "数据精度"=2, "数据值"=w856) -> ("编码输出"=w855:string)  [unwired: 6 in]
            n295 = call "数据编码整合输出.vi"("数据标识"="N" ("字符串"), "数据类型"="-Avg=", "污染物编码"="w01014", "数据值"=w888) -> ("编码输出"=w889:string)  [unwired: 7 in]
            n296 = call "数据编码整合输出.vi"("数据标识"="N" ("字符串"), "数据类型"="-Avg=", "污染物编码"="w01009", "数据值"=w895) -> ("编码输出"=w894:string)  [unwired: 7 in]
            n297 = call "数据编码整合输出.vi"("数据标识"="N" ("字符串"), "数据类型"="-Avg=", "污染物编码"="w19011", "数据值"=w874) -> ("编码输出"=w873:string)  [unwired: 7 in]
            n298 = call "数据编码整合输出.vi"("数据标识"="N" ("字符串"), "数据类型"="-Avg=", "污染物编码"="w01003", "数据值"=w884) -> ("编码输出"=w883:string)  [unwired: 7 in]
            n299 = call "数据编码整合输出.vi"("数据标识"="N" ("字符串"), "数据类型"="-Avg=", "污染物编码"="w01016", "数据值"=w879) -> ("编码输出"=w878:string)  [unwired: 7 in]
            n300 = call "数据编码整合输出.vi"("数据标识"="N" ("字符串"), "数据类型"="-Avg=", "污染物编码"="w21011", "数据精度"=3, "数据值"=w869) -> ("编码输出"=w868:string)  [unwired: 6 in]
            n301 = Format Into String(format string="DataTime=%s;%s%s%s%s%s%s%s%s%s%s%s%s" ("格式字符串"), w852, w919, w911, w905, w899, w894, w889, w883, w878, w873, w868, w863, w855) -> (resulting string=w854:string)  [unwired: 2 in, 1 out]
            n302 = Empty String/Path?(string/path=w852) -> (empty?=w851:bool)
            n303 = case shown="真" w851 {
              tunnel: w854 -> [w947 _]
              tunnel: [w947 ""] -> w853
              frame False {
              }
              frame True {
              }
            }
          }
          frame "返回执行结果" {
            w949 = 0 ("当前包数")
            n304 = property on="当前包数" class="DigNum (严格)"("Value"=w949) -> ()  [unwired: 2 in, 2 out]
            n305 = property on="总包数" class="DigNum (严格)"("Value"=w949) -> ()  [unwired: 2 in, 2 out]
            n306 = global write "全局1.vi" "枚举"(enum16{"返回请求应答", "上传数据", "返回执行结果"}."返回请求应答" ("枚举")) -> ()
          }
        }
        n307 = Concatenate Strings(w792, w798) -> (w790:string)
        n308 = String Length(string=w790) -> (length=w795:i32)
        n309 = Greater Or Equal?(x=w795, y=1024) -> (x >= y?=w789:bool)
        n310 = case shown="假" w789 {
          tunnel: [w823 TRUE ("值")] -> w793
          tunnel: [w824 w834] -> w791
          tunnel: w792 -> [_ w835]
          tunnel: w790 -> [w824 w833]
          frame False {
            n311 = global read "全局 小时数据发送次数.vi" "小时数据发送次数"() -> (w825:i32)
            n312 = global read "全局 数据数组大小.vi" "数据数组大小"() -> (w826:i32)
            n313 = Equal?(x=w825, y=w826) -> (x = y?=w827:bool)
            n314 = case shown="真" w827 {
              tunnel: [_ TRUE ("值")] -> w823
              frame False {
              }
              frame True {
                n315 = property on="当前包数" class="DigNum (严格)"() -> ("Value"=w830:i32)  [unwired: 2 in, 2 out]
                n316 = Increment(x=w830) -> (x+1=w829:i32)
                n317 = property on="当前包数" class="DigNum (严格)"("Value"=w829) -> ()  [unwired: 2 in, 2 out]
              }
            }
          }
          frame True {
            n318 = property on="当前包数" class="DigNum (严格)"() -> ("Value"=w841:i32)  [unwired: 2 in, 2 out]
            n319 = global read "全局 小时数据发送次数.vi" "小时数据发送次数"() -> (w837:i32)
            n320 = global read "全局 小时数据发送次数.vi" "小时数据发送次数"() -> (w832:i32)
            n321 = Increment(x=w841) -> (x+1=→"当前包数":i32)
            n322 = global read "全局 数据数组大小.vi" "数据数组大小"() -> (w838:i32)
            n323 = Equal?(x=w837, y=w838) -> (x = y?=w836:bool)
            n324 = Decrement(x=w832) -> (x-1=w831:i32)
            n325 = case shown="假" w836 {
              tunnel: w835 -> [w842 _]
              tunnel: [w842 w843] -> w834
              tunnel: w833 -> [_ w843]
              frame False {
              }
              frame True {
              }
            }
            n326 = global write "全局 小时数据发送次数.vi" "小时数据发送次数"(w831) -> ()
          }
        }
        n327 = global read "全局 小时数据发送次数.vi" "小时数据发送次数"() -> (w797:i32)
        n328 = global read "全局 数据数组大小.vi" "数据数组大小"() -> (w820:i32)
        n329 = global read "全局 数据数组大小.vi" "数据数组大小"() -> (w796:i32)
        n330 = Greater Or Equal?(x=w797, y=w796) -> (x >= y?=w767:bool)
        n331 = global read "全局1.vi" "枚举"() -> (w803:enum16{"返回请求应答", "上传数据", "返回执行结果"})
        n332 = Increment(x=w821) -> (x+1=w804:i32)
        n333 = Not Equal?(x=w803, y=enum16{"返回请求应答", "上传数据", "返回执行结果"}."上传数据") -> (x != y?=w801:bool)
        n334 = Greater Or Equal?(x=w804, y=w820) -> (x >= y?=w800:bool)
        n335 = Compound Arithmetic op=OR ("复合运算")(w767, w793, w801, w800) -> (w799:bool)
      }
      n336 = Unbundle By Name(w572) -> ("总磷"=w571:string[][], "总氮"=w570:string[][], "DO"=w569:string[][], "氨氮"=w568:string[][], "CODMn"=w567:string[][], "PH"=w565:string[][], "CODCr"=w566:string[][], "电导率"=w564:string[][], "水温"=w563:string[][], "浊度"=w562:string[][], "叶绿素"=w561:string[][], "藻密度"=w560:string[][])
      n337 = while {
        tunnel: w567 -> [w660]
        tunnel: w568 -> [w659]
        tunnel: w569 -> [w658]
        tunnel: w571 -> [w657]
        tunnel: w570 -> [w656]
        tunnel: [w633] -> w584 mode=indexing
        shift-right: [w639] -> _
        shift-left: "" -> [w638]
        tunnel: w566 -> [w616]
        tunnel: w565 -> [w618]
        tunnel: w564 -> [w624]
        tunnel: w563 -> [w621]
        tunnel: w562 -> [w611]
        tunnel: w561 -> [w609]
        tunnel: w560 -> [w608]
        i -> [w662]
        stop <- w634 stop-if-true
        n338 = property on="小时数据发送次数" class="DigNum (严格)"() -> ("Value"=w647:i32)  [unwired: 2 in, 2 out]
        n339 = property on="小时数据发送次数" class="DigNum (严格)"() -> ("Value"=w646:i32)  [unwired: 2 in, 2 out]
        n340 = property on="小时数据发送次数" class="DigNum (严格)"() -> ("Value"=w623:i32)  [unwired: 2 in, 2 out]
        n341 = property on="小时数据发送次数" class="DigNum (严格)"() -> ("Value"=w617:i32)  [unwired: 2 in, 2 out]
        n342 = property on="小时数据发送次数" class="DigNum (严格)"() -> ("Value"=w645:i32)  [unwired: 2 in, 2 out]
        n343 = property on="小时数据发送次数" class="DigNum (严格)"() -> ("Value"=w626:i32)  [unwired: 2 in, 2 out]
        n344 = property on="小时数据发送次数" class="DigNum (严格)"() -> ("Value"=w644:i32)  [unwired: 2 in, 2 out]
        n345 = property on="小时数据发送次数" class="DigNum (严格)"() -> ("Value"=w614:i32)  [unwired: 2 in, 2 out]
        n346 = property on="小时数据发送次数" class="DigNum (严格)"() -> ("Value"=w613:i32)  [unwired: 2 in, 2 out]
        n347 = property on="小时数据发送次数" class="DigNum (严格)"() -> ("Value"=w612:i32)  [unwired: 2 in, 2 out]
        n348 = property on="小时数据发送次数" class="DigNum (严格)"() -> ("Value"=w648:i32)  [unwired: 2 in, 2 out]
        n349 = property on="小时数据发送次数" class="DigNum (严格)"() -> ("Value"=w620:i32)  [unwired: 2 in, 2 out]
        n350 = global read "全局 数据数组大小.vi" "数据数组大小"() -> (w661:i32)
        n351 = global read "全局1.vi" "枚举"() -> (w650:enum16{"返回请求应答", "上传数据", "返回执行结果"})
        n352 = global read "全局1.vi" "枚举"() -> (w654:enum16{"返回请求应答", "上传数据", "返回执行结果"})
        n353 = Index Array(array=w660, index (row)=w647) -> (element=w627:string[])  [unwired: 1 in]
        n354 = Index Array(array=w659, index (row)=w646) -> (element=w628:string[])  [unwired: 1 in]
        n355 = Index Array(array=w621, index (row)=w623) -> (element=w622:string[])  [unwired: 1 in]
        n356 = Index Array(array=w616, index (row)=w617) -> (element=w615:string[])  [unwired: 1 in]
        n357 = Index Array(array=w658, index (row)=w645) -> (element=w629:string[])  [unwired: 1 in]
        n358 = Index Array(array=w624, index (row)=w626) -> (element=w625:string[])  [unwired: 1 in]
        n359 = Index Array(array=w657, index (row)=w644) -> (element=w631:string[])  [unwired: 1 in]
        n360 = Index Array(array=w611, index (row)=w614) -> (element=w610:string[])  [unwired: 1 in]
        n361 = Index Array(array=w609, index (row)=w613) -> (element=w606:string[])  [unwired: 1 in]
        n362 = Index Array(array=w608, index (row)=w612) -> (element=w607:string[])  [unwired: 1 in]
        n363 = Index Array(array=w656, index (row)=w648) -> (element=w630:string[])  [unwired: 1 in]
        n364 = Increment(x=w662) -> (x+1=w655:i32)
        n365 = Index Array(array=w618, index (row)=w620) -> (element=w619:string[])  [unwired: 1 in]
        n366 = global read "全局1.vi" "枚举"() -> (w632:enum16{"返回请求应答", "上传数据", "返回执行结果"})
        n367 = Equal?(x=w650, y=enum16{"返回请求应答", "上传数据", "返回执行结果"}."返回执行结果") -> (x = y?=w649:bool)
        n368 = Equal?(x=w654, y=enum16{"返回请求应答", "上传数据", "返回执行结果"}."返回请求应答") -> (x = y?=w652:bool)
        n369 = Greater Or Equal?(x=w655, y=w661) -> (x >= y?=w637:bool)
        n370 = Compound Arithmetic op=OR ("复合运算")(w649, w652, w637) -> (w634:bool)
        n371 = case shown="\"上传数据\"" w632 {
          tunnel: ["QnRtn=1" w746 "ExeRtn=1"] -> w633
          tunnel: w629 -> [_ w752 _]
          tunnel: w631 -> [_ w751 _]
          tunnel: w630 -> [_ w750 _]
          tunnel: w628 -> [_ w748 _]
          tunnel: w619 -> [_ w737 _]
          tunnel: w625 -> [_ w739 _]
          tunnel: w622 -> [_ w738 _]
          tunnel: w610 -> [_ w736 _]
          tunnel: w606 -> [_ w735 _]
          tunnel: w607 -> [_ w734 _]
          tunnel: w627 -> [_ w731 _]
          tunnel: w615 -> [_ w730 _]
          frame "返回请求应答", Default {
          }
          frame "上传数据" {
            # "PH"
            # "总氮"
            # "总磷"
            # "藻密度"
            # "叶绿素"
            # "浊度"
            # "电导率"
            # "DO"
            # "CODCr"
            # "水温"
            # "NH3"
            # "CODMn"
            n372 = Index Array(array=w737) -> (element #2=w664:string)  [unwired: 2 in, 1 out]
            n373 = Index Array(array=w750, index #1=0 ("索引"), index #2=1 ("索引")) -> (element #2=w667:string)  [unwired: 1 out]
            n374 = Index Array(array=w738) -> (element #2=w714:string)  [unwired: 2 in, 1 out]
            n375 = Index Array(array=w739) -> (element #2=w695:string)  [unwired: 2 in, 1 out]
            n376 = Index Array(array=w736) -> (element #2=w693:string)  [unwired: 2 in, 1 out]
            n377 = Index Array(array=w731, index #1=0 ("索引"), index #2=1 ("索引")) -> (element #1=w729:string, element #2=w725:string)
            n378 = Index Array(array=w748, index #1=0 ("索引"), index #2=1 ("索引")) -> (element #2=w719:string)  [unwired: 1 out]
            n379 = Index Array(array=w730, index #1=0 ("索引"), index #2=1 ("索引")) -> (element #2=w708:string)  [unwired: 1 out]
            n380 = Index Array(array=w752, index #1=0 ("索引")) -> (element #2=w697:string)  [unwired: 1 in, 1 out]
            n381 = Index Array(array=w751, index #1=0 ("索引"), index #2=1 ("索引")) -> (element #2=w669:string)  [unwired: 1 out]
            n382 = Index Array(array=w735) -> (element #2=w673:string)  [unwired: 2 in, 1 out]
            n383 = Index Array(array=w734) -> (element #2=w671:string)  [unwired: 2 in, 1 out]
            n384 = property on="小时数据发送次数" class="DigNum (严格)"() -> ("Value"=w733:i32)  [unwired: 2 in, 2 out]
            n385 = Increment(x=w733) -> (x+1=w732:i32)
            n386 = call "规范小时时间戳.vi"("字符串"=w729) -> ("result string"=w757:string)  [unwired: 10 in]
            n387 = property on="小时数据发送次数" class="DigNum (严格)"("Value"=w732) -> ()  [unwired: 2 in, 2 out]
            n388 = call "数据编码整合输出.vi"("数据标识"="N" ("字符串"), "数据类型"="-Avg=", "污染物编码"="w21001", "数据精度"=3, "数据值"=w667) -> ("编码输出"=w666:string)  [unwired: 6 in]
            n389 = call "数据编码整合输出.vi"("数据标识"="N" ("字符串"), "数据类型"="-Avg=", "污染物编码"="w01001", "数据精度"=2, "数据值"=w664) -> ("编码输出"=w665:string)  [unwired: 6 in]
            n390 = call "数据编码整合输出.vi"("数据标识"="N" ("字符串"), "数据类型"="-Avg=", "污染物编码"="w21011", "数据精度"=3, "数据值"=w669) -> ("编码输出"=w668:string)  [unwired: 6 in]
            n391 = call "数据编码整合输出.vi"("数据标识"="N" ("字符串"), "数据类型"="-Avg=", "污染物编码"="w19011", "数据值"=w671) -> ("编码输出"=w670:string)  [unwired: 7 in]
            n392 = call "数据编码整合输出.vi"("数据标识"="N" ("字符串"), "数据类型"="-Avg=", "污染物编码"="w01016", "数据值"=w673) -> ("编码输出"=w672:string)  [unwired: 7 in]
            n393 = call "数据编码整合输出.vi"("数据标识"="N" ("字符串"), "数据类型"="-Avg=", "污染物编码"="w01003", "数据值"=w693) -> ("编码输出"=w692:string)  [unwired: 7 in]
            n394 = call "数据编码整合输出.vi"("数据标识"="N" ("字符串"), "数据类型"="-Avg=", "污染物编码"="w01014", "数据值"=w695) -> ("编码输出"=w694:string)  [unwired: 7 in]
            n395 = call "数据编码整合输出.vi"("数据标识"="N" ("字符串"), "数据类型"="-Avg=", "污染物编码"="w01009", "数据值"=w697) -> ("编码输出"=w696:string)  [unwired: 7 in]
            n396 = call "数据编码整合输出.vi"("数据标识"="N" ("字符串"), "数据类型"="-Avg=", "污染物编码"="w01018", "数据精度"=3, "数据值"=w708) -> ("编码输出"=w707:string)  [unwired: 6 in]
            n397 = call "数据编码整合输出.vi"("数据标识"="N" ("字符串"), "数据类型"="-Avg=", "污染物编码"="w01010", "数据值"=w714) -> ("编码输出"=w713:string)  [unwired: 7 in]
            n398 = call "数据编码整合输出.vi"("数据标识"="N" ("字符串"), "数据类型"="-Avg=", "污染物编码"="w21003", "数据精度"=3, "数据值"=w719) -> ("编码输出"=w718:string)  [unwired: 6 in]
            n399 = call "数据编码整合输出.vi"("数据标识"="N" ("字符串"), "数据类型"="-Avg=", "污染物编码"="w01019", "数据值"=w725) -> ("编码输出"=w724:string)  [unwired: 7 in]
            n400 = Format Into String(format string="DataTime=%s;%s%s%s%s%s%s%s%s%s%s%s%s" ("格式字符串"), w757, w724, w718, w713, w707, w696, w694, w692, w672, w670, w668, w666, w665) -> (resulting string=w746:string)  [unwired: 2 in, 1 out]
          }
          frame "返回执行结果" {
          }
        }
        n401 = call <vilib>:"Boolean Crossing PtByPt.vi"("direction"=enum16{"either", "false-true", "true-false"}."false-true", "input"=w634) -> ("crossing"=w636:bool)  [unwired: 1 in]
        n402 = case shown="真" w636 {
          frame False {
          }
          frame True {
            n403 = property on="包数" class="DigNum (严格)"() -> ("Value"=w760:i32)  [unwired: 2 in, 2 out]
            n404 = Increment(x=w760) -> (x+1=→"总包数":i32)
          }
        }
        n405 = Concatenate Strings(w638, w633) -> (w640:string)
        n406 = String Length(string=w640) -> (length=w643:i32)
        n407 = Greater Or Equal?(x=w643, y=1024) -> (x >= y?=w641:bool)
        n408 = case shown="真" w641 {
          tunnel: w640 -> [w761 _]
          tunnel: [w761 w762] -> w639
          tunnel: w633 -> [_ w762]
          frame False {
          }
          frame True {
            n409 = property on="包数" class="DigNum (严格)"() -> ("Value"=w766:i32)  [unwired: 2 in, 2 out]
            n410 = property on="小时数据发送次数" class="DigNum (严格)"() -> ("Value"=w764:i32)  [unwired: 2 in, 2 out]
            n411 = Increment(x=w766) -> (x+1=→"包数":i32)
            n412 = Decrement(x=w764) -> (x-1=w763:i32)
            n413 = property on="小时数据发送次数" class="DigNum (严格)"("Value"=w763) -> ()  [unwired: 2 in, 2 out]
          }
        }
      }
      n414 = global read "全局1.vi" "枚举"() -> (w583:enum16{"返回请求应答", "上传数据", "返回执行结果"})
      n415 = Equal?(x=w583, y=enum16{"返回请求应答", "上传数据", "返回执行结果"}."上传数据") -> (x = y?=w581:bool)
      n416 = case shown="真" w581 {
        tunnel: w584 -> [_ w601]
        tunnel: [w592 w597] -> w559
        tunnel: [w592 w593] -> w558
        frame False {
          w592 = ""
        }
        frame True {
          n417 = for {
            tunnel: w601 -> [w605] mode=indexing
            shift-right: [w603] -> w602
            shift-left: "" -> [w604]
            n418 = Concatenate Strings(w604, w605) -> (w603:string)
          }
          "数据区" <- w602
          n419 = String Length(string=w602) -> (length=w598:i32)
          n420 = property on="总包数" class="DigNum (严格)"() -> ("Value"=w594:i32)  [unwired: 2 in, 2 out]
          n421 = Quotient & Remainder(x=w598, y=834) -> (floor(x/y)=w596:i32)  [unwired: 1 out]
          n422 = Increment(x=w596) -> (x+1=w595:i32)
          n423 = Number To Decimal String(number=w595) -> (decimal integer string=w597:string)  [unwired: 1 in]
          n424 = Number To Decimal String(number=w594) -> (decimal integer string=w593:string)  [unwired: 1 in]
        }
      }
      "总包数" <- w559
    }
    frame "提取实时数据" {
      # "提取实时数据"
      n425 = global read "插值后的新数组.vi" "插值后的数组元素"() -> (w966:T3)
      n426 = Unbundle By Name(w966) -> ("总磷"=w965:string[][], "总氮"=w964:string[][], "DO"=w963:string[][], "氨氮"=w962:string[][], "CODMn"=w961:string[][], "PH"=w959:string[][], "CODCr"=w960:string[][], "电导率"=w958:string[][], "水温"=w957:string[][], "浊度"=w956:string[][], "叶绿素"=w955:string[][], "藻密度"=w954:string[][])
      n427 = while {
        tunnel: w983 -> [w1292]
        tunnel: w982 -> [w1288]
        tunnel: w981 -> [w1286]
        tunnel: w980 -> [w1283]
        tunnel: w979 -> [w1280]
        tunnel: [w1239] -> w985
        shift-right: [w1239] -> _
        shift-left: "" -> [w1242]
        tunnel: w973 -> [w1275]
        tunnel: w972 -> [w1271]
        tunnel: w971 -> [w1269]
        tunnel: w970 -> [w1266]
        tunnel: w969 -> [w1262]
        tunnel: w968 -> [w1259]
        tunnel: w967 -> [w1258]
        i -> [w1244]
        stop <- w1240 stop-if-true
        # "叶绿素"
        # "浊度"
        # "电导率"
        n428 = global read "全局 小时数据发送次数.vi" "小时数据发送次数"() -> (w1276:i32)
        n429 = global read "全局 小时数据发送次数.vi" "小时数据发送次数"() -> (w1270:i32)
        n430 = global read "全局 小时数据发送次数.vi" "小时数据发送次数"() -> (w1261:i32)
        n431 = global read "全局 小时数据发送次数.vi" "小时数据发送次数"() -> (w1290:i32)
        n432 = global read "全局 小时数据发送次数.vi" "小时数据发送次数"() -> (w1293:i32)
        n433 = global read "全局 小时数据发送次数.vi" "小时数据发送次数"() -> (w1284:i32)
        n434 = global read "全局 小时数据发送次数.vi" "小时数据发送次数"() -> (w1264:i32)
        n435 = global read "全局 小时数据发送次数.vi" "小时数据发送次数"() -> (w1287:i32)
        n436 = global read "全局 小时数据发送次数.vi" "小时数据发送次数"() -> (w1260:i32)
        n437 = global read "全局 小时数据发送次数.vi" "小时数据发送次数"() -> (w1267:i32)
        n438 = global read "全局 小时数据发送次数.vi" "小时数据发送次数"() -> (w1281:i32)
        n439 = global read "全局 小时数据发送次数.vi" "小时数据发送次数"() -> (w1272:i32)
        n440 = global read "全局 小时数据发送次数.vi" "小时数据发送次数"() -> (w1278:i32)
        n441 = global read "全局 数据数组大小.vi" "数据数组大小"() -> (w1277:i32)
        n442 = Index Array(array=w1275, index (row)=w1276) -> (element=w1274:string[])  [unwired: 1 in]
        n443 = Greater Or Equal?(x=w1278, y=w1277) -> (x >= y?=w1241:bool)
        n444 = Index Array(array=w1292, index (row)=w1293) -> (element=w1291:string[])  [unwired: 1 in]
        n445 = Index Array(array=w1288, index (row)=w1290) -> (element=w1289:string[])  [unwired: 1 in]
        n446 = Index Array(array=w1266, index (row)=w1267) -> (element=w1265:string[])  [unwired: 1 in]
        n447 = Index Array(array=w1271, index (row)=w1272) -> (element=w1273:string[])  [unwired: 1 in]
        n448 = Index Array(array=w1286, index (row)=w1287) -> (element=w1285:string[])  [unwired: 1 in]
        n449 = Index Array(array=w1269, index (row)=w1270) -> (element=w1268:string[])  [unwired: 1 in]
        n450 = Index Array(array=w1283, index (row)=w1284) -> (element=w1282:string[])  [unwired: 1 in]
        n451 = Index Array(array=w1262, index (row)=w1264) -> (element=w1263:string[])  [unwired: 1 in]
        n452 = Index Array(array=w1259, index (row)=w1261) -> (element=w1257:string[])  [unwired: 1 in]
        n453 = Index Array(array=w1280, index (row)=w1281) -> (element=w1279:string[])  [unwired: 1 in]
        n454 = Index Array(array=w1258, index (row)=w1260) -> (element=w1256:string[])  [unwired: 1 in]
        n455 = global read "全局1.vi" "枚举"() -> (w1294:enum16{"返回请求应答", "上传数据", "返回执行结果"})
        n456 = case shown="\"上传数据\"" w1294 {
          tunnel: ["QnRtn=1" w1327 "ExeRtn=1"] -> w1243
          tunnel: w1291 -> [_ w1416 _]
          tunnel: w1285 -> [_ w1433 _]
          tunnel: w1282 -> [_ w1432 _]
          tunnel: w1279 -> [_ w1431 _]
          tunnel: w1289 -> [_ w1429 _]
          tunnel: w1274 -> [_ w1415 _]
          tunnel: w1273 -> [_ w1421 _]
          tunnel: w1268 -> [_ w1418 _]
          tunnel: w1265 -> [_ w1417 _]
          tunnel: w1263 -> [_ w1414 _]
          tunnel: w1257 -> [_ w1413 _]
          tunnel: w1256 -> [_ w1412 _]
          frame "返回请求应答", Default {
            n457 = local write "总包数"("" ("总包数")) -> ()
            n458 = property on="当前包数" class="DigNum (严格)"("Value"=0 ("当前包数")) -> ()  [unwired: 2 in, 2 out]
            n459 = global read "全局 数据数组大小.vi" "数据数组大小"() -> (w1316:i32)
            n460 = global write "全局1.vi" "枚举"(enum16{"返回请求应答", "上传数据", "返回执行结果"}."上传数据" ("枚举")) -> ()
            n461 = Equal To 0?(x=w1316) -> (x = 0?=w1317:bool)
            n462 = case shown="真" w1317 {
              frame False {
              }
              frame True {
                n463 = global read "全局 小时数据发送次数.vi" "小时数据发送次数"() -> (w1323:i32)
                n464 = Increment(x=w1323) -> (x+1=w1322:i32)
                n465 = global write "全局 小时数据发送次数.vi" "小时数据发送次数"(w1322) -> ()
              }
            }
          }
          frame "上传数据" {
            (unwired) "-Rtd=" ("数据类型")
            # "PH"
            # "总氮"
            # "总磷"
            # "藻密度"
            # "叶绿素"
            # "浊度"
            # "电导率"
            # "DO"
            # "CODCr"
            # "水温"
            # "NH3"
            # "CODMn"
            n466 = Index Array(array=w1415, index #2=3 ("索引"), index #3=5 ("索引")) -> (element #2=w1328:string, element #3=w1329:string)  [unwired: 1 in, 1 out]
            n467 = Index Array(array=w1431, index #1=0 ("索引"), index #2=3 ("索引"), index #3=5 ("索引")) -> (element #2=w1331:string, element #3=w1332:string)  [unwired: 1 out]
            n468 = Index Array(array=w1413, index #2=3 ("索引"), index #3=5 ("索引")) -> (element #2=w1340:string, element #3=w1341:string)  [unwired: 1 in, 1 out]
            n469 = Index Array(array=w1412, index #2=3 ("索引"), index #3=5 ("索引")) -> (element #2=w1337:string, element #3=w1338:string)  [unwired: 1 in, 1 out]
            n470 = Index Array(array=w1417, index #2=3 ("索引"), index #3=5 ("索引")) -> (element #2=w1377:string, element #3=w1378:string)  [unwired: 1 in, 1 out]
            n471 = Index Array(array=w1418, index #2=3 ("索引"), index #3=5 ("索引")) -> (element #2=w1361:string, element #3=w1362:string)  [unwired: 1 in, 1 out]
            n472 = Index Array(array=w1414, index #2=3 ("索引"), index #3=5 ("索引")) -> (element #2=w1344:string, element #3=w1345:string)  [unwired: 1 in, 1 out]
            n473 = Index Array(array=w1432, index #1=0 ("索引"), index #2=3 ("索引"), index #3=5 ("索引")) -> (element #2=w1334:string, element #3=w1335:string)  [unwired: 1 out]
            n474 = Index Array(array=w1416, index #1=0 ("索引"), index #2=3 ("索引"), index #3=5 ("索引")) -> (element #1=w1392:string, element #2=w1389:string, element #3=w1388:string)
            n475 = Index Array(array=w1429, index #1=0 ("索引"), index #2=3 ("索引"), index #3=5 ("索引")) -> (element #2=w1380:string, element #3=w1381:string)  [unwired: 1 out]
            n476 = Index Array(array=w1421, index #1=0 ("索引"), index #2=3 ("索引"), index #3=5 ("索引")) -> (element #2=w1367:string, element #3=w1368:string)  [unwired: 1 out]
            n477 = Index Array(array=w1433, index #1=0 ("索引"), index #2=3 ("索引"), index #3=5 ("索引")) -> (element #2=w1364:string, element #3=w1365:string)  [unwired: 1 out]
            n478 = global read "全局 小时数据发送次数.vi" "小时数据发送次数"() -> (w1428:i32)
            n479 = call "规范小时时间戳.vi"("字符串"=w1392) -> ("result string"=w1325:string)  [unwired: 10 in]
            n480 = Increment(x=w1428) -> (x+1=w1427:i32)
            n481 = global write "全局 小时数据发送次数.vi" "小时数据发送次数"(w1427) -> ()
            n482 = call "数据编码整合输出.vi"("数据标识"=w1329, "数据类型"="-Rtd=", "污染物编码"="w01001", "数据精度"=2, "数据值"=w1328) -> ("编码输出"=w1330:string)  [unwired: 6 in]
            n483 = call "数据编码整合输出.vi"("数据标识"=w1388, "数据类型"="-Rtd=", "污染物编码"="w01019", "数据值"=w1389) -> ("编码输出"=w1387:string)  [unwired: 7 in]
            n484 = call "数据编码整合输出.vi"("数据标识"=w1381, "数据类型"="-Rtd=", "污染物编码"="w21003", "数据精度"=3 ("精度"), "数据值"=w1380) -> ("编码输出"=w1379:string)  [unwired: 6 in]
            n485 = call "数据编码整合输出.vi"("数据标识"=w1332, "数据类型"="-Rtd=", "污染物编码"="w21001", "数据精度"=3, "数据值"=w1331) -> ("编码输出"=w1333:string)  [unwired: 6 in]
            n486 = call "数据编码整合输出.vi"("数据标识"=w1341, "数据类型"="-Rtd=", "污染物编码"="w01016", "数据值"=w1340) -> ("编码输出"=w1342:string)  [unwired: 7 in]
            n487 = call "数据编码整合输出.vi"("数据标识"=w1338, "数据类型"="-Rtd=", "污染物编码"="w19011", "数据值"=w1337) -> ("编码输出"=w1339:string)  [unwired: 7 in]
            n488 = call "数据编码整合输出.vi"("数据标识"=w1335, "污染物编码"="w21011", "数据精度"=3, "数据值"=w1334) -> ("编码输出"=w1336:string)  [unwired: 7 in]
            n489 = call "数据编码整合输出.vi"("数据标识"=w1368, "数据类型"="-Rtd=", "污染物编码"="w01018", "数据精度"=3, "数据值"=w1367) -> ("编码输出"=w1366:string)  [unwired: 6 in]
            n490 = call "数据编码整合输出.vi"("数据标识"=w1378, "数据类型"="-Rtd=", "污染物编码"="w01010", "数据值"=w1377) -> ("编码输出"=w1376:string)  [unwired: 7 in]
            n491 = call "数据编码整合输出.vi"("数据标识"=w1345, "数据类型"="-Rtd=", "污染物编码"="w01003", "数据值"=w1344) -> ("编码输出"=w1343:string)  [unwired: 7 in]
            n492 = call "数据编码整合输出.vi"("数据标识"=w1362, "数据类型"="-Rtd=", "污染物编码"="w01014", "数据值"=w1361) -> ("编码输出"=w1360:string)  [unwired: 7 in]
            n493 = call "数据编码整合输出.vi"("数据标识"=w1365, "数据类型"="-Rtd=", "污染物编码"="w01009", "数据值"=w1364) -> ("编码输出"=w1363:string)  [unwired: 7 in]
            n494 = Format Into String(format string="DataTime=%s;%s%s%s%s%s%s%s%s%s%s%s%s" ("格式字符串"), w1325, w1387, w1379, w1376, w1366, w1363, w1360, w1343, w1342, w1339, w1336, w1333, w1330) -> (resulting string=w1326:string)  [unwired: 2 in, 1 out]
            n495 = Empty String/Path?(string/path=w1325) -> (empty?=w1324:bool)
            n496 = case shown="真" w1324 {
              tunnel: [w1438 ""] -> w1327
              tunnel: w1326 -> [w1438 _]
              frame False {
              }
              frame True {
              }
            }
          }
          frame "返回执行结果" {
            n497 = local write "总包数"("" ("总包数")) -> ()
            n498 = property on="当前包数" class="DigNum (严格)"("Value"=0 ("当前包数")) -> ()  [unwired: 2 in, 2 out]
            n499 = global write "全局1.vi" "枚举"(enum16{"返回请求应答", "上传数据", "返回执行结果"}."返回请求应答" ("枚举")) -> ()
          }
        }
        n500 = Concatenate Strings(w1242, w1243) -> (w1246:string)
        n501 = String Length(string=w1246) -> (length=w1249:i32)
        n502 = Greater Or Equal?(x=w1249, y=1024) -> (x >= y?=w1245:bool)
        n503 = case shown="真" w1245 {
          tunnel: [w1295 TRUE ("值")] -> w1247
          tunnel: [w1296 w1308] -> w1239
          tunnel: w1242 -> [_ w1309]
          tunnel: w1246 -> [w1296 w1307]
          frame False {
            n504 = global read "全局 小时数据发送次数.vi" "小时数据发送次数"() -> (w1297:i32)
            n505 = global read "全局 数据数组大小.vi" "数据数组大小"() -> (w1298:i32)
            n506 = Equal?(x=w1297, y=w1298) -> (x = y?=w1299:bool)
            n507 = case shown="真" w1299 {
              tunnel: [_ TRUE ("值")] -> w1295
              frame False {
              }
              frame True {
                n508 = property on="当前包数" class="DigNum (严格)"() -> ("Value"=w1301:i32)  [unwired: 2 in, 2 out]
                n509 = Increment(x=w1301) -> (x+1=w1300:i32)
                n510 = property on="当前包数" class="DigNum (严格)"("Value"=w1300) -> ()  [unwired: 2 in, 2 out]
              }
            }
          }
          frame True {
            n511 = property on="当前包数" class="DigNum (严格)"() -> ("Value"=w1304:i32)  [unwired: 2 in, 2 out]
            n512 = global read "全局 小时数据发送次数.vi" "小时数据发送次数"() -> (w1311:i32)
            n513 = global read "全局 小时数据发送次数.vi" "小时数据发送次数"() -> (w1306:i32)
            n514 = global read "全局 数据数组大小.vi" "数据数组大小"() -> (w1312:i32)
            n515 = Increment(x=w1304) -> (x+1=w1303:i32)
            n516 = property on="当前包数" class="DigNum (严格)"("Value"=w1303) -> ()  [unwired: 2 in, 2 out]
            n517 = Equal?(x=w1311, y=w1312) -> (x = y?=w1310:bool)
            n518 = Decrement(x=w1306) -> (x-1=w1305:i32)
            n519 = case shown="假" w1310 {
              tunnel: w1309 -> [w1314 _]
              tunnel: [w1314 w1315] -> w1308
              tunnel: w1307 -> [_ w1315]
              frame False {
              }
              frame True {
              }
            }
            n520 = global write "全局 小时数据发送次数.vi" "小时数据发送次数"(w1305) -> ()
          }
        }
        n521 = global read "全局 数据数组大小.vi" "数据数组大小"() -> (w1255:i32)
        n522 = global read "全局1.vi" "枚举"() -> (w1253:enum16{"返回请求应答", "上传数据", "返回执行结果"})
        n523 = Increment(x=w1244) -> (x+1=w1254:i32)
        n524 = Not Equal?(x=w1253, y=enum16{"返回请求应答", "上传数据", "返回执行结果"}."上传数据") -> (x != y?=w1251:bool)
        n525 = Greater Or Equal?(x=w1254, y=w1255) -> (x >= y?=w1250:bool)
        n526 = Compound Arithmetic op=OR ("复合运算")(w1241, w1247, w1251, w1250) -> (w1240:bool)
      }
      n527 = while {
        tunnel: w961 -> [w1054]
        tunnel: w962 -> [w1053]
        tunnel: w963 -> [w1052]
        tunnel: w965 -> [w1051]
        tunnel: w964 -> [w1050]
        tunnel: [w1027] -> w978 mode=indexing
        shift-right: [w1033] -> _
        shift-left: "" -> [w1032]
        tunnel: w960 -> [w1010]
        tunnel: w959 -> [w1012]
        tunnel: w958 -> [w1018]
        tunnel: w957 -> [w1015]
        tunnel: w956 -> [w1005]
        tunnel: w955 -> [w1003]
        tunnel: w954 -> [w1002]
        i -> [w1056]
        stop <- w1028 stop-if-true
        n528 = property on="小时数据发送次数" class="DigNum (严格)"() -> ("Value"=w1041:i32)  [unwired: 2 in, 2 out]
        n529 = property on="小时数据发送次数" class="DigNum (严格)"() -> ("Value"=w1040:i32)  [unwired: 2 in, 2 out]
        n530 = property on="小时数据发送次数" class="DigNum (严格)"() -> ("Value"=w1017:i32)  [unwired: 2 in, 2 out]
        n531 = property on="小时数据发送次数" class="DigNum (严格)"() -> ("Value"=w1011:i32)  [unwired: 2 in, 2 out]
        n532 = property on="小时数据发送次数" class="DigNum (严格)"() -> ("Value"=w1039:i32)  [unwired: 2 in, 2 out]
        n533 = property on="小时数据发送次数" class="DigNum (严格)"() -> ("Value"=w1020:i32)  [unwired: 2 in, 2 out]
        n534 = property on="小时数据发送次数" class="DigNum (严格)"() -> ("Value"=w1038:i32)  [unwired: 2 in, 2 out]
        n535 = property on="小时数据发送次数" class="DigNum (严格)"() -> ("Value"=w1008:i32)  [unwired: 2 in, 2 out]
        n536 = property on="小时数据发送次数" class="DigNum (严格)"() -> ("Value"=w1007:i32)  [unwired: 2 in, 2 out]
        n537 = property on="小时数据发送次数" class="DigNum (严格)"() -> ("Value"=w1006:i32)  [unwired: 2 in, 2 out]
        n538 = property on="小时数据发送次数" class="DigNum (严格)"() -> ("Value"=w1042:i32)  [unwired: 2 in, 2 out]
        n539 = property on="小时数据发送次数" class="DigNum (严格)"() -> ("Value"=w1014:i32)  [unwired: 2 in, 2 out]
        n540 = global read "全局 数据数组大小.vi" "数据数组大小"() -> (w1055:i32)
        n541 = global read "全局1.vi" "枚举"() -> (w1044:enum16{"返回请求应答", "上传数据", "返回执行结果"})
        n542 = global read "全局1.vi" "枚举"() -> (w1048:enum16{"返回请求应答", "上传数据", "返回执行结果"})
        n543 = Index Array(array=w1054, index (row)=w1041) -> (element=w1021:string[])  [unwired: 1 in]
        n544 = Index Array(array=w1053, index (row)=w1040) -> (element=w1022:string[])  [unwired: 1 in]
        n545 = Index Array(array=w1015, index (row)=w1017) -> (element=w1016:string[])  [unwired: 1 in]
        n546 = Index Array(array=w1010, index (row)=w1011) -> (element=w1009:string[])  [unwired: 1 in]
        n547 = Index Array(array=w1052, index (row)=w1039) -> (element=w1023:string[])  [unwired: 1 in]
        n548 = Index Array(array=w1018, index (row)=w1020) -> (element=w1019:string[])  [unwired: 1 in]
        n549 = Index Array(array=w1051, index (row)=w1038) -> (element=w1025:string[])  [unwired: 1 in]
        n550 = Index Array(array=w1005, index (row)=w1008) -> (element=w1004:string[])  [unwired: 1 in]
        n551 = Index Array(array=w1003, index (row)=w1007) -> (element=w1000:string[])  [unwired: 1 in]
        n552 = Index Array(array=w1002, index (row)=w1006) -> (element=w1001:string[])  [unwired: 1 in]
        n553 = Index Array(array=w1050, index (row)=w1042) -> (element=w1024:string[])  [unwired: 1 in]
        n554 = Index Array(array=w1012, index (row)=w1014) -> (element=w1013:string[])  [unwired: 1 in]
        n555 = Increment(x=w1056) -> (x+1=w1049:i32)
        n556 = global read "全局1.vi" "枚举"() -> (w1026:enum16{"返回请求应答", "上传数据", "返回执行结果"})
        n557 = Equal?(x=w1044, y=enum16{"返回请求应答", "上传数据", "返回执行结果"}."返回执行结果") -> (x = y?=w1043:bool)
        n558 = Equal?(x=w1048, y=enum16{"返回请求应答", "上传数据", "返回执行结果"}."返回请求应答") -> (x = y?=w1046:bool)
        n559 = Greater Or Equal?(x=w1049, y=w1055) -> (x >= y?=w1031:bool)
        n560 = case shown="\"上传数据\"" w1026 {
          tunnel: ["QnRtn=1" w1113 "ExeRtn=1"] -> w1027
          tunnel: w1023 -> [_ w1132 _]
          tunnel: w1025 -> [_ w1131 _]
          tunnel: w1024 -> [_ w1130 _]
          tunnel: w1022 -> [_ w1128 _]
          tunnel: w1013 -> [_ w1089 _]
          tunnel: w1019 -> [_ w1098 _]
          tunnel: w1016 -> [_ w1096 _]
          tunnel: w1004 -> [_ w1084 _]
          tunnel: w1000 -> [_ w1077 _]
          tunnel: w1001 -> [_ w1076 _]
          tunnel: w1021 -> [_ w1069 _]
          tunnel: w1009 -> [_ w1066 _]
          frame "返回请求应答", Default {
          }
          frame "上传数据" {
            # "将非空数组的时间戳写入"
            n561 = Index Array(array=w1096, index #2=3 ("索引")) -> (element #2=w1091:string)  [unwired: 1 in, 1 out]
            n562 = Index Array(array=w1098, index #2=3 ("索引")) -> (element #2=w1068:string)  [unwired: 1 in, 1 out]
            n563 = Index Array(array=w1084, index #2=3 ("索引")) -> (element #2=w1073:string)  [unwired: 1 in, 1 out]
            n564 = Index Array(array=w1077, index #2=3 ("索引")) -> (element #2=w1075:string)  [unwired: 1 in, 1 out]
            n565 = Index Array(array=w1076, index #2=3 ("索引")) -> (element #2=w1074:string)  [unwired: 1 in, 1 out]
            n566 = Index Array(array=w1089, index #2=3 ("索引")) -> (element #2=w1067:string)  [unwired: 1 in, 1 out]
            n567 = Index Array(array=w1069, index #1=0 ("索引"), index #2=3 ("索引")) -> (element #2=w1126:string)  [unwired: 1 out]
            n568 = Index Array(array=w1128, index #1=0 ("索引"), index #2=3 ("索引")) -> (element #2=w1123:string)  [unwired: 1 out]
            n569 = Index Array(array=w1066, index #1=0 ("索引"), index #2=3 ("索引")) -> (element #2=w1104:string)  [unwired: 1 out]
            n570 = Index Array(array=w1132, index #1=0 ("索引"), index #2=3 ("索引")) -> (element #2=w1102:string)  [unwired: 1 out]
            n571 = Index Array(array=w1131, index #1=0 ("索引"), index #2=3 ("索引")) -> (element #1=w1058:string, element #2=w1103:string)
            n572 = Index Array(array=w1130, index #1=0 ("索引"), index #2=3 ("索引")) -> (element #2=w1116:string)  [unwired: 1 out]
            n573 = Empty String/Path?(string/path=w1091) -> (empty?=w1094:bool)
            n574 = Empty String/Path?(string/path=w1068) -> (empty?=w1120:bool)
            n575 = Empty String/Path?(string/path=w1073) -> (empty?=w1086:bool)
            n576 = Empty String/Path?(string/path=w1075) -> (empty?=w1081:bool)
            n577 = Empty String/Path?(string/path=w1074) -> (empty?=w1080:bool)
            n578 = Empty String/Path?(string/path=w1067) -> (empty?=w1093:bool)
            n579 = property on="小时数据发送次数" class="DigNum (严格)"() -> ("Value"=w1071:i32)  [unwired: 2 in, 2 out]
            n580 = Empty String/Path?(string/path=w1116) -> (empty?=w1117:bool)
            n581 = Empty String/Path?(string/path=w1126) -> (empty?=w1127:bool)
            n582 = Empty String/Path?(string/path=w1123) -> (empty?=w1124:bool)
            n583 = Empty String/Path?(string/path=w1102) -> (empty?=w1121:bool)
            n584 = Empty String/Path?(string/path=w1103) -> (empty?=w1119:bool)
            n585 = Not(x=w1094) -> (.not. x?=w1092:bool)
            n586 = Not(x=w1120) -> (.not. x?=w1097:bool)
            n587 = Not(x=w1086) -> (.not. x?=w1085:bool)
            n588 = Not(x=w1081) -> (.not. x?=w1078:bool)
            n589 = Not(x=w1080) -> (.not. x?=w1079:bool)
            n590 = Not(x=w1093) -> (.not. x?=w1090:bool)
            n591 = case shown="真" w1092 {
              tunnel: ["" ("编码输出") w1173] -> w1095
              tunnel: w1091 -> [_ w1174]
              frame False {
              }
              frame True {
                n592 = call "字符串精度转换.vi"("输入字符串"=w1174) -> ("输出字符串"=w1172:string)  [unwired: 10 in]
                n593 = call "污染物CP编码.vi"("字符串"="N", "数据类型"="-Rtd=", "污染物浓度"=w1172, "污染物编码"="w01010") -> ("编码输出"=w1173:string)  [unwired: 6 in]
              }
            }
            n594 = case shown="真" w1085 {
              tunnel: ["" ("编码输出") w1160] -> w1087
              tunnel: w1073 -> [_ w1159]
              frame False {
              }
              frame True {
                n595 = call "字符串精度转换.vi"("输入字符串"=w1159) -> ("输出字符串"=w1158:string)  [unwired: 10 in]
                n596 = call "污染物CP编码.vi"("字符串"="N", "数据类型"="-Rtd=", "污染物浓度"=w1158, "污染物编码"="w01003") -> ("编码输出"=w1160:string)  [unwired: 6 in]
              }
            }
            n597 = case shown="真" w1078 {
              tunnel: ["" ("编码输出") w1153] -> w1083
              tunnel: w1075 -> [_ w1152]
              frame False {
              }
              frame True {
                n598 = call "字符串精度转换.vi"("输入字符串"=w1152) -> ("输出字符串"=w1151:string)  [unwired: 10 in]
                n599 = call "污染物CP编码.vi"("字符串"="N", "数据类型"="-Rtd=", "污染物浓度"=w1151, "污染物编码"="w01016") -> ("编码输出"=w1153:string)  [unwired: 6 in]
              }
            }
            n600 = case shown="真" w1079 {
              tunnel: ["" ("编码输出") w1146] -> w1082
              tunnel: w1074 -> [_ w1145]
              frame False {
              }
              frame True {
                n601 = call "字符串精度转换.vi"("输入字符串"=w1145) -> ("输出字符串"=w1144:string)  [unwired: 10 in]
                n602 = call "污染物CP编码.vi"("字符串"="N", "数据类型"="-Rtd=", "污染物浓度"=w1144, "污染物编码"="w19011") -> ("编码输出"=w1146:string)  [unwired: 6 in]
              }
            }
            n603 = case shown="真" w1090 {
              tunnel: ["" ("编码输出") w1167] -> w1088
              tunnel: w1067 -> [_ w1166]
              frame False {
              }
              frame True {
                n604 = call "字符串精度转换.vi"("输入字符串"=w1166) -> ("输出字符串"=w1165:string)  [unwired: 10 in]
                n605 = call "污染物CP编码.vi"("字符串"="N", "数据类型"="-Rtd=", "污染物浓度"=w1165, "污染物编码"="w01001") -> ("编码输出"=w1167:string)  [unwired: 6 in]
              }
            }
            n606 = Increment(x=w1071) -> (x+1=w1070:i32)
            n607 = Not(x=w1127) -> (.not. x?=w1125:bool)
            n608 = Not(x=w1124) -> (.not. x?=w1122:bool)
            n609 = Not(x=w1121) -> (.not. x?=w1099:bool)
            n610 = Not(x=w1119) -> (.not. x?=w1118:bool)
            n611 = case shown="真" w1097 {
              tunnel: ["" ("编码输出") w1180] -> w1100
              tunnel: w1068 -> [_ w1181]
              frame False {
              }
              frame True {
                n612 = call "字符串精度转换.vi"("输入字符串"=w1181) -> ("输出字符串"=w1179:string)  [unwired: 10 in]
                n613 = call "污染物CP编码.vi"("字符串"="N", "数据类型"="-Rtd=", "污染物浓度"=w1179, "污染物编码"="w01014") -> ("编码输出"=w1180:string)  [unwired: 6 in]
              }
            }
            n614 = property on="小时数据发送次数" class="DigNum (严格)"("Value"=w1070) -> ()  [unwired: 2 in, 2 out]
            n615 = call "规范小时时间戳.vi"("字符串"=w1058) -> ("result string"=w1140:string)  [unwired: 10 in]
            n616 = case shown="真" w1125 {
              tunnel: ["" ("编码输出") w1228] -> w1141
              tunnel: w1126 -> [_ w1226]
              frame False {
              }
              frame True {
                n617 = call "字符串精度转换.vi"("输入字符串"=w1226) -> ("输出字符串"=w1225:string)  [unwired: 10 in]
                n618 = call "污染物CP编码.vi"("字符串"="N", "数据类型"="-Rtd=", "污染物浓度"=w1225, "污染物编码"="w01019") -> ("编码输出"=w1228:string)  [unwired: 6 in]
              }
            }
            n619 = case shown="真" w1122 {
              tunnel: ["" ("编码输出") w1220] -> w1138
              tunnel: w1123 -> [_ w1219]
              frame False {
              }
              frame True {
                n620 = call "字符串精度转换.vi"("精度"=3, "输入字符串"=w1219) -> ("输出字符串"=w1217:string)  [unwired: 9 in]
                n621 = call "污染物CP编码.vi"("字符串"="N", "数据类型"="-Rtd=", "污染物浓度"=w1217, "污染物编码"="w21003") -> ("编码输出"=w1220:string)  [unwired: 6 in]
              }
            }
            n622 = case shown="真" w1099 {
              tunnel: ["" ("编码输出") w1187] -> w1101
              tunnel: w1102 -> [_ w1188]
              frame False {
              }
              frame True {
                n623 = call "字符串精度转换.vi"("输入字符串"=w1188) -> ("输出字符串"=w1186:string)  [unwired: 10 in]
                n624 = call "污染物CP编码.vi"("字符串"="N", "数据类型"="-Rtd=", "污染物浓度"=w1186, "污染物编码"="w01009") -> ("编码输出"=w1187:string)  [unwired: 6 in]
              }
            }
            n625 = case shown="真" w1118 {
              tunnel: ["" ("编码输出") w1211] -> w1135
              tunnel: w1103 -> [_ w1210]
              frame False {
              }
              frame True {
                n626 = call "字符串精度转换.vi"("精度"=3, "输入字符串"=w1210) -> ("输出字符串"=w1209:string)  [unwired: 9 in]
                n627 = call "污染物CP编码.vi"("字符串"="N", "数据类型"="-Rtd=", "污染物浓度"=w1209, "污染物编码"="w21011") -> ("编码输出"=w1211:string)  [unwired: 6 in]
              }
            }
            n628 = Empty String/Path?(string/path=w1104) -> (empty?=w1112:bool)
            n629 = Not(x=w1112) -> (.not. x?=w1111:bool)
            n630 = case shown="真" w1111 {
              tunnel: w1104 -> [_ w1197]
              tunnel: ["" ("编码输出") w1194] -> w1072
              frame False {
              }
              frame True {
                n631 = call "字符串精度转换.vi"("精度"=3, "输入字符串"=w1197) -> ("输出字符串"=w1193:string)  [unwired: 9 in]
                n632 = call "污染物CP编码.vi"("字符串"="N", "数据类型"="-Rtd=", "污染物浓度"=w1193, "污染物编码"="w01018") -> ("编码输出"=w1194:string)  [unwired: 6 in]
              }
            }
            n633 = Not(x=w1117) -> (.not. x?=w1115:bool)
            n634 = case shown="真" w1115 {
              tunnel: ["" ("编码输出") w1203] -> w1133
              tunnel: w1116 -> [_ w1202]
              frame False {
              }
              frame True {
                n635 = call "字符串精度转换.vi"("精度"=3, "输入字符串"=w1202) -> ("输出字符串"=w1201:string)  [unwired: 9 in]
                n636 = call "污染物CP编码.vi"("字符串"="N", "数据类型"="-Rtd=", "污染物浓度"=w1201, "污染物编码"="w21001") -> ("编码输出"=w1203:string)  [unwired: 6 in]
              }
            }
            n637 = Format Into String(format string="DataTime=%s;%s%s%s%s%s%s%s%s%s%s%s%s" ("格式字符串"), w1140, w1141, w1138, w1095, w1072, w1101, w1100, w1087, w1083, w1082, w1135, w1133, w1088) -> (resulting string=w1113:string)  [unwired: 2 in, 1 out]
          }
          frame "返回执行结果" {
          }
        }
        n638 = Compound Arithmetic op=OR ("复合运算")(w1043, w1046, w1031) -> (w1028:bool)
        n639 = call <vilib>:"Boolean Crossing PtByPt.vi"("direction"=enum16{"either", "false-true", "true-false"}."false-true", "input"=w1028) -> ("crossing"=w1030:bool)  [unwired: 1 in]
        n640 = case shown="真" w1030 {
          frame False {
          }
          frame True {
            n641 = property on="包数" class="DigNum (严格)"() -> ("Value"=w1232:i32)  [unwired: 2 in, 2 out]
            n642 = Increment(x=w1232) -> (x+1=w1231:i32)
            n643 = property on="总包数" class="DigNum (严格)"("Value"=w1231) -> ()  [unwired: 2 in, 2 out]
          }
        }
        n644 = Concatenate Strings(w1032, w1027) -> (w1034:string)
        n645 = String Length(string=w1034) -> (length=w1037:i32)
        n646 = Greater Or Equal?(x=w1037, y=1024) -> (x >= y?=w1035:bool)
        n647 = case shown="真" w1035 {
          tunnel: w1034 -> [w1233 _]
          tunnel: [w1233 w1236] -> w1033
          tunnel: w1027 -> [_ w1236]
          frame False {
          }
          frame True {
            n648 = property on="包数" class="DigNum (严格)"() -> ("Value"=w1235:i32)  [unwired: 2 in, 2 out]
            n649 = property on="小时数据发送次数" class="DigNum (严格)"() -> ("Value"=w1238:i32)  [unwired: 2 in, 2 out]
            n650 = Increment(x=w1235) -> (x+1=w1234:i32)
            n651 = Decrement(x=w1238) -> (x-1=w1237:i32)
            n652 = property on="小时数据发送次数" class="DigNum (严格)"("Value"=w1237) -> ()  [unwired: 2 in, 2 out]
            n653 = property on="包数" class="DigNum (严格)"("Value"=w1234) -> ()  [unwired: 2 in, 2 out]
          }
        }
      }
      n654 = global read "全局1.vi" "枚举"() -> (w977:enum16{"返回请求应答", "上传数据", "返回执行结果"})
      n655 = Equal?(x=w977, y=enum16{"返回请求应答", "上传数据", "返回执行结果"}."上传数据") -> (x = y?=w975:bool)
      n656 = case shown="真" w975 {
        tunnel: w978 -> [_ w996]
        tunnel: [w986 w992] -> w953
        tunnel: [w986 w988] -> w952
        frame False {
          w986 = ""
        }
        frame True {
          n657 = for {
            tunnel: w996 -> [w999] mode=indexing
            shift-right: [w997] -> w989
            shift-left: "" -> [w998]
            n658 = Concatenate Strings(w998, w999) -> (w997:string)
          }
          n659 = local write "数据区"(w989) -> ()
          n660 = String Length(string=w989) -> (length=w993:i32)
          n661 = property on="总包数" class="DigNum (严格)"() -> ("Value"=w987:i32)  [unwired: 2 in, 2 out]
          n662 = Quotient & Remainder(x=w993, y=834) -> (floor(x/y)=w991:i32)  [unwired: 1 out]
          n663 = Increment(x=w991) -> (x+1=w990:i32)
          n664 = Number To Decimal String(number=w990) -> (decimal integer string=w992:string)  [unwired: 1 in]
          n665 = Number To Decimal String(number=w987) -> (decimal integer string=w988:string)  [unwired: 1 in]
        }
      }
      n666 = local write "总包数"(w953) -> ()
    }
    frame "核查数据", "跨度核查", "零点核查" {
      # "发送零点核查数据/跨度核查数据/核查数据"
      n667 = while {
        tunnel: w1457 -> [w1493]
        tunnel: w1456 -> [w1492]
        tunnel: w1455 -> [w1491]
        tunnel: w1454 -> [w1490]
        tunnel: w1453 -> [w1489]
        tunnel: [w1473] -> w1449 mode=indexing
        tunnel: w1444 -> [w1472]
        i -> [w1495]
        stop <- w1486 stop-if-true
        n668 = property on="核查数据发送次数" class="DigNum (严格)"() -> ("Value"=w1471:i32)  [unwired: 2 in, 2 out]
        n669 = global read "全局 数据数组大小.vi" "数据数组大小"() -> (w1494:i32)
        n670 = Index Array(array=w1493, index (row)=w1471) -> (element=w1479:string[])  [unwired: 1 in]
        n671 = Index Array(array=w1492, index (row)=w1471) -> (element=w1478:string[])  [unwired: 1 in]
        n672 = Index Array(array=w1490, index (row)=w1471) -> (element=w1475:string[])  [unwired: 1 in]
        n673 = Index Array(array=w1472, index (row)=w1471) -> (element=w1470:string[])  [unwired: 1 in]
        n674 = Index Array(array=w1491, index (row)=w1471) -> (element=w1476:string[])  [unwired: 1 in]
        n675 = global read "全局1.vi" "枚举"() -> (w1481:enum16{"返回请求应答", "上传数据", "返回执行结果"})
        n676 = global read "全局1.vi" "枚举"() -> (w1485:enum16{"返回请求应答", "上传数据", "返回执行结果"})
        n677 = Index Array(array=w1489, index (row)=w1471) -> (element=w1474:string[])  [unwired: 1 in]
        n678 = Increment(x=w1495) -> (x+1=w1488:i32)
        n679 = global read "全局1.vi" "枚举"() -> (w1477:enum16{"返回请求应答", "上传数据", "返回执行结果"})
        n680 = Equal?(x=w1481, y=enum16{"返回请求应答", "上传数据", "返回执行结果"}."返回执行结果") -> (x = y?=w1480:bool)
        n681 = Equal?(x=w1485, y=enum16{"返回请求应答", "上传数据", "返回执行结果"}."返回请求应答") -> (x = y?=w1483:bool)
        n682 = Greater Or Equal?(x=w1488, y=w1494) -> (x >= y?=w1487:bool)
        n683 = case shown="\"上传数据\"" w1477 {
          tunnel: ["QnRtn=1" w1545 "ExeRtn=1"] -> w1473
          tunnel: w1479 -> [_ w1559 _]
          tunnel: w1476 -> [_ _ _]
          tunnel: w1475 -> [_ w1558 _]
          tunnel: w1474 -> [_ w1557 _]
          tunnel: w1478 -> [_ w1555 _]
          tunnel: w1470 -> [_ w1502 _]
          frame "返回请求应答", Default {
          }
          frame "上传数据" {
            n684 = Index Array(array=w1557, index #1=0 ("索引"), index #2=3 ("索引"), index #3=7 ("索引")) -> (element #2=w1548:string, element #3=w1523:string)  [unwired: 1 out]
            n685 = Index Array(array=w1559, index #1=0 ("索引"), index #2=3 ("索引"), index #3=7 ("索引")) -> (element #1=w1501:string, element #2=w1543:string, element #3=w1539:string)
            n686 = Index Array(array=w1555, index #1=0 ("索引"), index #2=3 ("索引"), index #3=7 ("索引")) -> (element #2=w1535:string, element #3=w1533:string)  [unwired: 1 out]
            n687 = Index Array(array=w1558, index #1=0 ("索引"), index #2=3 ("索引"), index #3=7 ("索引")) -> (element #2=w1551:string, element #3=w1525:string)  [unwired: 1 out]
            n688 = Index Array(array=w1502, index #1=0 ("索引"), index #2=3 ("索引"), index #3=7 ("索引")) -> (element #2=w1505:string, element #3=w1503:string)  [unwired: 1 out]
            n689 = property on="核查数据发送次数" class="DigNum (严格)"() -> ("Value"=w1519:i32)  [unwired: 2 in, 2 out]
            n690 = Empty String/Path?(string/path=w1523) -> (empty?=w1524:bool)
            n691 = Empty String/Path?(string/path=w1551) -> (empty?=w1552:bool)
            n692 = Empty String/Path?(string/path=w1525) -> (empty?=w1527:bool)
            n693 = Empty String/Path?(string/path=w1505) -> (empty?=w1509:bool)
            n694 = Not(x=w1524) -> (.not. x?=w1522:bool)
            n695 = Not(x=w1552) -> (.not. x?=w1550:bool)
            n696 = Not(x=w1527) -> (.not. x?=w1526:bool)
            n697 = Empty String/Path?(string/path=w1533) -> (empty?=w1497:bool)
            n698 = Increment(x=w1519) -> (x+1=w1518:i32)
            n699 = Empty String/Path?(string/path=w1539) -> (empty?=w1541:bool)
            n700 = Empty String/Path?(string/path=w1535) -> (empty?=w1553:bool)
            n701 = Not(x=w1497) -> (.not. x?=w1534:bool)
            n702 = Empty String/Path?(string/path=w1543) -> (empty?=w1554:bool)
            n703 = Not(x=w1509) -> (.not. x?=w1508:bool)
            n704 = Not(x=w1554) -> (.not. x?=w1544:bool)
            n705 = Not(x=w1541) -> (.not. x?=w1540:bool)
            n706 = Not(x=w1553) -> (.not. x?=w1536:bool)
            n707 = Empty String/Path?(string/path=w1548) -> (empty?=w1549:bool)
            n708 = call "规范小时时间戳.vi"("字符串"=w1501) -> ("result string"=w1563:string)  [unwired: 10 in]
            n709 = case shown="真" w1522 {
              tunnel: ["" ("编码输出") w1585] -> w1520
              tunnel: w1523 -> [_ w1584]
              frame False {
              }
              frame True {
                n710 = call "字符串精度转换.vi"("精度"=3, "输入字符串"=w1584) -> ("输出字符串"=w1582:string)  [unwired: 9 in]
                n711 = call "污染物CP编码.vi"("字段结束"=TRUE, "数据类型"="-StandardValue=", "污染物浓度"=w1582, "污染物编码"="w21001") -> ("编码输出"=w1585:string)  [unwired: 6 in]
              }
            }
            n712 = case shown="真" w1508 {
              tunnel: w1505 -> [_ w1578]
              tunnel: ["" ("编码输出") w1574] -> w1498
              tunnel: w1503 -> [_ w1570]
              frame False {
              }
              frame True {
                n713 = call "字符串精度转换.vi"("精度"=3, "输入字符串"=w1570) -> ("输出字符串"=w1566:string)  [unwired: 9 in]
                n714 = call "污染物CP编码.vi"("字段结束"=TRUE, "数据类型"="-StandardValue=", "污染物浓度"=w1566, "污染物编码"="w01018") -> ("编码输出"=w1569:string)  [unwired: 6 in]
                n715 = call "字符串精度转换.vi"("精度"=3, "输入字符串"=w1578) -> ("输出字符串"=w1567:string)  [unwired: 9 in]
                n716 = call "污染物CP编码.vi"("字段结束"=FALSE, "数据类型"="-Check=", "污染物浓度"=w1567, "污染物编码"="w01018") -> ("编码输出"=w1575:string)  [unwired: 6 in]
                n717 = Concatenate Strings(w1575, w1569) -> (w1574:string)
              }
            }
            n718 = case shown="真" w1550 {
              tunnel: ["" ("编码输出") w1639] -> w1529
              tunnel: w1551 -> [_ w1638]
              frame False {
              }
              frame True {
                n719 = call "字符串精度转换.vi"("精度"=3, "输入字符串"=w1638) -> ("输出字符串"=w1635:string)  [unwired: 9 in]
                n720 = call "污染物CP编码.vi"("字段结束"=FALSE, "数据类型"="-Check=", "污染物浓度"=w1635, "污染物编码"="w21011") -> ("编码输出"=w1639:string)  [unwired: 6 in]
              }
            }
            n721 = case shown="真" w1526 {
              tunnel: ["" ("编码输出") w1593] -> w1528
              tunnel: w1525 -> [_ w1592]
              frame False {
              }
              frame True {
                n722 = call "字符串精度转换.vi"("精度"=3, "输入字符串"=w1592) -> ("输出字符串"=w1589:string)  [unwired: 9 in]
                n723 = call "污染物CP编码.vi"("字段结束"=TRUE, "数据类型"="-StandardValue=", "污染物浓度"=w1589, "污染物编码"="w21011") -> ("编码输出"=w1593:string)  [unwired: 6 in]
              }
            }
            n724 = property on="核查数据发送次数" class="DigNum (严格)"("Value"=w1518) -> ()  [unwired: 2 in, 2 out]
            n725 = case shown="真" w1544 {
              tunnel: w1543 -> [_ w1624]
              tunnel: ["" ("编码输出") w1622] -> w1542
              frame False {
              }
              frame True {
                # "污染物CP编码"
                n726 = call "字符串精度转换.vi"("输入字符串"=w1624) -> ("输出字符串"=w1620:string)  [unwired: 10 in]
                n727 = call "污染物CP编码.vi"("字段结束"=FALSE, "数据类型"="-Check=", "污染物浓度"=w1620, "污染物编码"="w01019") -> ("编码输出"=w1622:string)  [unwired: 6 in]
              }
            }
            n728 = case shown="真" w1540 {
              tunnel: w1539 -> [_ w1617]
              tunnel: ["" ("编码输出") w1615] -> w1538
              frame False {
              }
              frame True {
                # "污染物CP编码"
                n729 = call "字符串精度转换.vi"("输入字符串"=w1617) -> ("输出字符串"=w1613:string)  [unwired: 10 in]
                n730 = call "污染物CP编码.vi"("字段结束"=TRUE, "数据类型"="-StandardValue=", "污染物浓度"=w1613, "污染物编码"="w01019") -> ("编码输出"=w1615:string)  [unwired: 6 in]
              }
            }
            n731 = case shown="真" w1534 {
              tunnel: w1533 -> [_ w1600]
              tunnel: ["" ("编码输出") w1598] -> w1531
              frame False {
              }
              frame True {
                # "污染物CP编码"
                n732 = call "字符串精度转换.vi"("精度"=3, "输入字符串"=w1600) -> ("输出字符串"=w1597:string)  [unwired: 9 in]
                n733 = call "污染物CP编码.vi"("字段结束"=TRUE, "数据类型"="-StandardValue=", "污染物浓度"=w1597, "污染物编码"="w21003") -> ("编码输出"=w1598:string)  [unwired: 6 in]
              }
            }
            n734 = case shown="真" w1536 {
              tunnel: w1535 -> [_ w1608]
              tunnel: ["" ("编码输出") w1607] -> w1532
              frame False {
              }
              frame True {
                # "污染物CP编码"
                n735 = call "字符串精度转换.vi"("精度"=3, "输入字符串"=w1608) -> ("输出字符串"=w1605:string)  [unwired: 9 in]
                n736 = call "污染物CP编码.vi"("字段结束"=FALSE, "数据类型"="-Check=", "污染物浓度"=w1605, "污染物编码"="w21003") -> ("编码输出"=w1607:string)  [unwired: 6 in]
              }
            }
            n737 = Not(x=w1549) -> (.not. x?=w1547:bool)
            n738 = case shown="真" w1547 {
              tunnel: ["" ("编码输出") w1631] -> w1521
              tunnel: w1548 -> [_ w1630]
              frame False {
              }
              frame True {
                n739 = call "字符串精度转换.vi"("精度"=3, "输入字符串"=w1630) -> ("输出字符串"=w1627:string)  [unwired: 9 in]
                n740 = call "污染物CP编码.vi"("字段结束"=FALSE, "数据类型"="-Check=", "污染物浓度"=w1627, "污染物编码"="w21001") -> ("编码输出"=w1631:string)  [unwired: 6 in]
              }
            }
            n741 = Concatenate Strings(w1529, w1528) -> (w1500:string)
            n742 = Concatenate Strings(w1521, w1520) -> (w1499:string)
            n743 = Concatenate Strings(w1542, w1538) -> (w1537:string)
            n744 = Concatenate Strings(w1532, w1531) -> (w1530:string)
            n745 = Format Into String(format string="DataTime=%s;%s%s%s%s%s" ("格式字符串"), w1563, w1537, w1530, w1500, w1499, w1498) -> (resulting string=w1545:string)  [unwired: 2 in, 1 out]
          }
          frame "返回执行结果" {
          }
        }
        n746 = Compound Arithmetic op=OR ("复合运算")(w1480, w1483, w1487) -> (w1486:bool)
      }
      n747 = while {
        tunnel: w1457 -> [w1673]
        tunnel: w1456 -> [w1669]
        tunnel: w1455 -> [_]
        tunnel: w1454 -> [w1667]
        tunnel: w1453 -> [w1664]
        tunnel: [w1652] -> w1448
        shift-right: [w1652] -> _
        shift-left: "" -> [w1651]
        tunnel: w1444 -> [w1644]
        tunnel: w1445 -> [_]
        i -> [w1676]
        stop <- w1657 stop-if-true
        n748 = global read "全局 小时数据发送次数.vi" "小时数据发送次数"() -> (w1654:i32)
        n749 = global read "全局 小时数据发送次数.vi" "小时数据发送次数"() -> (w1671:i32)
        n750 = global read "全局 小时数据发送次数.vi" "小时数据发送次数"() -> (w1674:i32)
        n751 = global read "全局 小时数据发送次数.vi" "小时数据发送次数"() -> (w1668:i32)
        n752 = global read "全局 小时数据发送次数.vi" "小时数据发送次数"() -> (w1645:i32)
        n753 = global read "全局 数据数组大小.vi" "数据数组大小"() -> (w1653:i32)
        n754 = global read "全局 小时数据发送次数.vi" "小时数据发送次数"() -> (w1665:i32)
        n755 = Greater Or Equal?(x=w1654, y=w1653) -> (x >= y?=w1656:bool)
        n756 = Index Array(array=w1669, index (row)=w1671) -> (element=w1670:string[])  [unwired: 1 in]
        n757 = Index Array(array=w1673, index (row)=w1674) -> (element=w1672:string[])  [unwired: 1 in]
        n758 = Index Array(array=w1667, index (row)=w1668) -> (element=w1666:string[])  [unwired: 1 in]
        n759 = Index Array(array=w1644, index (row)=w1645) -> (element=w1643:string[])  [unwired: 1 in]
        n760 = Index Array(array=w1664, index (row)=w1665) -> (element=w1663:string[])  [unwired: 1 in]
        n761 = global read "全局1.vi" "枚举"() -> (w1677:enum16{"返回请求应答", "上传数据", "返回执行结果"})
        n762 = case shown="\"返回执行结果\"" w1677 {
          tunnel: ["QnRtn=1" w1708 "ExeRtn=1"] -> w1655
          tunnel: w1672 -> [_ w1771 _]
          tunnel: w1666 -> [_ w1770 _]
          tunnel: w1663 -> [_ w1769 _]
          tunnel: w1670 -> [_ w1767 _]
          tunnel: w1643 -> [_ w1716 _]
          frame "返回请求应答", Default {
            n763 = property on="当前包数" class="DigNum (严格)"("Value"=0 ("当前包数")) -> ()  [unwired: 2 in, 2 out]
            n764 = global read "全局 数据数组大小.vi" "数据数组大小"() -> (w1701:i32)
            n765 = global write "全局1.vi" "枚举"(enum16{"返回请求应答", "上传数据", "返回执行结果"}."上传数据" ("枚举")) -> ()
            n766 = Equal To 0?(x=w1701) -> (x = 0?=w1700:bool)
            n767 = case shown="真" w1700 {
              frame False {
              }
              frame True {
                n768 = global read "全局 小时数据发送次数.vi" "小时数据发送次数"() -> (w1705:i32)
                n769 = Increment(x=w1705) -> (x+1=w1704:i32)
                n770 = global write "全局 小时数据发送次数.vi" "小时数据发送次数"(w1704) -> ()
              }
            }
          }
          frame "上传数据" {
            # "五参数没有核查数据"
            # "将非空数组的时间戳写入"
            n771 = Index Array(array=w1769, index #1=0 ("索引"), index #2=3 ("索引"), index #3=7 ("索引")) -> (element #2=w1760:string, element #3=w1735:string)  [unwired: 1 out]
            n772 = Index Array(array=w1767, index #1=0 ("索引"), index #2=3 ("索引"), index #3=7 ("索引")) -> (element #1=w1713:string, element #2=w1748:string, element #3=w1745:string)
            n773 = Index Array(array=w1771, index #1=0 ("索引"), index #2=3 ("索引"), index #3=7 ("索引")) -> (element #2=w1756:string, element #3=w1752:string)  [unwired: 1 out]
            n774 = Index Array(array=w1770, index #1=0 ("索引"), index #2=3 ("索引"), index #3=7 ("索引")) -> (element #2=w1763:string, element #3=w1737:string)  [unwired: 1 out]
            n775 = Index Array(array=w1716, index #1=0 ("索引"), index #2=3 ("索引"), index #3=7 ("索引")) -> (element #2=w1717:string, element #3=w1714:string)  [unwired: 1 out]
            n776 = global read "全局 小时数据发送次数.vi" "小时数据发送次数"() -> (w1731:i32)
            n777 = Empty String/Path?(string/path=w1763) -> (empty?=w1764:bool)
            n778 = Empty String/Path?(string/path=w1737) -> (empty?=w1739:bool)
            n779 = Empty String/Path?(string/path=w1760) -> (empty?=w1761:bool)
            n780 = Empty String/Path?(string/path=w1735) -> (empty?=w1736:bool)
            n781 = Empty String/Path?(string/path=w1756) -> (empty?=w1766:bool)
            n782 = Empty String/Path?(string/path=w1752) -> (empty?=w1754:bool)
            n783 = Empty String/Path?(string/path=w1745) -> (empty?=w1747:bool)
            n784 = Empty String/Path?(string/path=w1717) -> (empty?=w1721:bool)
            n785 = Empty String/Path?(string/path=w1748) -> (empty?=w1765:bool)
            n786 = Not(x=w1764) -> (.not. x?=w1762:bool)
            n787 = Not(x=w1739) -> (.not. x?=w1738:bool)
            n788 = Not(x=w1761) -> (.not. x?=w1759:bool)
            n789 = Not(x=w1736) -> (.not. x?=w1734:bool)
            n790 = Not(x=w1766) -> (.not. x?=w1757:bool)
            n791 = Not(x=w1754) -> (.not. x?=w1753:bool)
            n792 = Not(x=w1721) -> (.not. x?=w1720:bool)
            n793 = Not(x=w1747) -> (.not. x?=w1746:bool)
            n794 = case shown="真" w1762 {
              tunnel: ["" ("编码输出") w1862] -> w1741
              tunnel: w1763 -> [_ w1861]
              frame False {
              }
              frame True {
                n795 = call "字符串精度转换.vi"("精度"=3, "输入字符串"=w1861) -> ("输出字符串"=w1858:string)  [unwired: 9 in]
                n796 = call "污染物CP编码.vi"("字符串"="N", "字段结束"=FALSE, "数据类型"="-Check=", "污染物浓度"=w1858, "污染物编码"="w21011") -> ("编码输出"=w1862:string)  [unwired: 5 in]
              }
            }
            n797 = case shown="真" w1738 {
              tunnel: ["" ("编码输出") w1810] -> w1740
              tunnel: w1737 -> [_ w1809]
              frame False {
              }
              frame True {
                n798 = call "字符串精度转换.vi"("精度"=3, "输入字符串"=w1809) -> ("输出字符串"=w1806:string)  [unwired: 9 in]
                n799 = call "污染物CP编码.vi"("字符串"="N", "字段结束"=TRUE, "数据类型"="-StandardValue=", "污染物浓度"=w1806, "污染物编码"="w21011") -> ("编码输出"=w1810:string)  [unwired: 5 in]
              }
            }
            n800 = case shown="真" w1759 {
              tunnel: ["" ("编码输出") w1853] -> w1733
              tunnel: w1760 -> [_ w1852]
              frame False {
              }
              frame True {
                n801 = call "字符串精度转换.vi"("精度"=3, "输入字符串"=w1852) -> ("输出字符串"=w1849:string)  [unwired: 9 in]
                n802 = call "污染物CP编码.vi"("字符串"="N", "字段结束"=FALSE, "数据类型"="-Check=", "污染物浓度"=w1849, "污染物编码"="w21001") -> ("编码输出"=w1853:string)  [unwired: 5 in]
              }
            }
            n803 = case shown="真" w1734 {
              tunnel: ["" ("编码输出") w1801] -> w1732
              tunnel: w1735 -> [_ w1800]
              frame False {
              }
              frame True {
                n804 = call "字符串精度转换.vi"("精度"=3, "输入字符串"=w1800) -> ("输出字符串"=w1798:string)  [unwired: 9 in]
                n805 = call "污染物CP编码.vi"("字符串"="N", "字段结束"=TRUE, "数据类型"="-StandardValue=", "污染物浓度"=w1798, "污染物编码"="w21001") -> ("编码输出"=w1801:string)  [unwired: 5 in]
              }
            }
            n806 = case shown="真" w1720 {
              tunnel: w1717 -> [_ w1793]
              tunnel: ["" ("编码输出") w1789] -> w1710
              tunnel: w1714 -> [_ w1785]
              frame False {
              }
              frame True {
                n807 = call "字符串精度转换.vi"("精度"=3, "输入字符串"=w1785) -> ("输出字符串"=w1781:string)  [unwired: 9 in]
                n808 = call "污染物CP编码.vi"("字符串"="N", "字段结束"=TRUE, "数据类型"="-StandardValue=", "污染物浓度"=w1781, "污染物编码"="w01018") -> ("编码输出"=w1784:string)  [unwired: 5 in]
                n809 = call "字符串精度转换.vi"("精度"=3, "输入字符串"=w1793) -> ("输出字符串"=w1782:string)  [unwired: 9 in]
                n810 = call "污染物CP编码.vi"("字符串"="N", "字段结束"=FALSE, "数据类型"="-Check=", "污染物浓度"=w1782, "污染物编码"="w01018") -> ("编码输出"=w1790:string)  [unwired: 5 in]
                n811 = Concatenate Strings(w1790, w1784) -> (w1789:string)
              }
            }
            n812 = case shown="真" w1757 {
              tunnel: w1756 -> [_ w1845]
              tunnel: ["" ("编码输出") w1843] -> w1755
              frame False {
              }
              frame True {
                # "污染物CP编码"
                n813 = call "字符串精度转换.vi"("输入字符串"=w1845) -> ("输出字符串"=w1841:string)  [unwired: 10 in]
                n814 = call "污染物CP编码.vi"("字符串"="N", "字段结束"=FALSE, "数据类型"="-Check=", "污染物浓度"=w1841, "污染物编码"="w01019") -> ("编码输出"=w1843:string)  [unwired: 5 in]
              }
            }
            n815 = case shown="真" w1753 {
              tunnel: w1752 -> [_ w1837]
              tunnel: ["" ("编码输出") w1835] -> w1751
              frame False {
              }
              frame True {
                # "污染物CP编码"
                n816 = call "字符串精度转换.vi"("输入字符串"=w1837) -> ("输出字符串"=w1833:string)  [unwired: 10 in]
                n817 = call "污染物CP编码.vi"("字符串"="N", "字段结束"=TRUE, "数据类型"="-StandardValue=", "污染物浓度"=w1833, "污染物编码"="w01019") -> ("编码输出"=w1835:string)  [unwired: 5 in]
              }
            }
            n818 = Increment(x=w1731) -> (x+1=w1730:i32)
            n819 = Not(x=w1765) -> (.not. x?=w1749:bool)
            n820 = global write "全局 小时数据发送次数.vi" "小时数据发送次数"(w1730) -> ()
            n821 = case shown="真" w1749 {
              tunnel: w1748 -> [_ w1827]
              tunnel: ["" ("编码输出") w1826] -> w1744
              frame False {
              }
              frame True {
                # "污染物CP编码"
                n822 = call "字符串精度转换.vi"("精度"=3, "输入字符串"=w1827) -> ("输出字符串"=w1824:string)  [unwired: 9 in]
                n823 = call "污染物CP编码.vi"("字符串"="N", "字段结束"=FALSE, "数据类型"="-Check=", "污染物浓度"=w1824, "污染物编码"="w21003") -> ("编码输出"=w1826:string)  [unwired: 5 in]
              }
            }
            n824 = case shown="真" w1746 {
              tunnel: w1745 -> [_ w1818]
              tunnel: ["" ("编码输出") w1816] -> w1743
              frame False {
              }
              frame True {
                # "污染物CP编码"
                n825 = call "字符串精度转换.vi"("精度"=3, "输入字符串"=w1818) -> ("输出字符串"=w1815:string)  [unwired: 9 in]
                n826 = call "污染物CP编码.vi"("字符串"="N", "字段结束"=TRUE, "数据类型"="-StandardValue=", "污染物浓度"=w1815, "污染物编码"="w21003") -> ("编码输出"=w1816:string)  [unwired: 5 in]
              }
            }
            n827 = call "规范小时时间戳.vi"("字符串"=w1713) -> ("result string"=w1706:string)  [unwired: 10 in]
            n828 = Concatenate Strings(w1741, w1740) -> (w1712:string)
            n829 = Concatenate Strings(w1733, w1732) -> (w1711:string)
            n830 = Concatenate Strings(w1755, w1751) -> (w1750:string)
            n831 = Concatenate Strings(w1744, w1743) -> (w1742:string)
            n832 = Format Into String(format string="DataTime=%s;%s%s%s%s%s" ("格式字符串"), w1706, w1750, w1742, w1712, w1711, w1710) -> (resulting string=w1709:string)  [unwired: 2 in, 1 out]
            n833 = Empty String/Path?(string/path=w1706) -> (empty?=w1707:bool)
            n834 = case shown="真" w1707 {
              tunnel: [w1775 ""] -> w1708
              tunnel: w1709 -> [w1775 _]
              frame False {
              }
              frame True {
              }
            }
          }
          frame "返回执行结果" {
            n835 = property on="当前包数" class="DigNum (严格)"("Value"=0 ("当前包数")) -> ()  [unwired: 2 in, 2 out]
            n836 = global write "全局1.vi" "枚举"(enum16{"返回请求应答", "上传数据", "返回执行结果"}."返回请求应答" ("枚举")) -> ()
          }
        }
        n837 = Concatenate Strings(w1651, w1655) -> (w1650:string)
        n838 = String Length(string=w1650) -> (length=w1648:i32)
        n839 = Greater Or Equal?(x=w1648, y=1024) -> (x >= y?=w1646:bool)
        n840 = case shown="真" w1646 {
          tunnel: [w1678 TRUE ("值")] -> w1649
          tunnel: [w1679 w1691] -> w1652
          tunnel: w1651 -> [_ w1692]
          tunnel: w1650 -> [w1679 w1690]
          frame False {
            n841 = global read "全局 小时数据发送次数.vi" "小时数据发送次数"() -> (w1680:i32)
            n842 = global read "全局 数据数组大小.vi" "数据数组大小"() -> (w1681:i32)
            n843 = Equal?(x=w1680, y=w1681) -> (x = y?=w1682:bool)
            n844 = case shown="真" w1682 {
              tunnel: [_ TRUE ("值")] -> w1678
              frame False {
              }
              frame True {
                n845 = property on="当前包数" class="DigNum (严格)"() -> ("Value"=w1684:i32)  [unwired: 2 in, 2 out]
                n846 = Increment(x=w1684) -> (x+1=w1683:i32)
                n847 = property on="当前包数" class="DigNum (严格)"("Value"=w1683) -> ()  [unwired: 2 in, 2 out]
              }
            }
          }
          frame True {
            n848 = property on="当前包数" class="DigNum (严格)"() -> ("Value"=w1687:i32)  [unwired: 2 in, 2 out]
            n849 = global read "全局 小时数据发送次数.vi" "小时数据发送次数"() -> (w1694:i32)
            n850 = global read "全局 小时数据发送次数.vi" "小时数据发送次数"() -> (w1689:i32)
            n851 = global read "全局 数据数组大小.vi" "数据数组大小"() -> (w1695:i32)
            n852 = Increment(x=w1687) -> (x+1=w1686:i32)
            n853 = property on="当前包数" class="DigNum (严格)"("Value"=w1686) -> ()  [unwired: 2 in, 2 out]
            n854 = Equal?(x=w1694, y=w1695) -> (x = y?=w1693:bool)
            n855 = Decrement(x=w1689) -> (x-1=w1688:i32)
            n856 = case shown="假" w1693 {
              tunnel: w1692 -> [w1697 _]
              tunnel: [w1697 w1698] -> w1691
              tunnel: w1690 -> [_ w1698]
              frame False {
              }
              frame True {
              }
            }
            n857 = global write "全局 小时数据发送次数.vi" "小时数据发送次数"(w1688) -> ()
          }
        }
        n858 = global read "全局 数据数组大小.vi" "数据数组大小"() -> (w1675:i32)
        n859 = global read "全局1.vi" "枚举"() -> (w1661:enum16{"返回请求应答", "上传数据", "返回执行结果"})
        n860 = Increment(x=w1676) -> (x+1=w1662:i32)
        n861 = Not Equal?(x=w1661, y=enum16{"返回请求应答", "上传数据", "返回执行结果"}."上传数据") -> (x != y?=w1659:bool)
        n862 = Greater Or Equal?(x=w1662, y=w1675) -> (x >= y?=w1658:bool)
        n863 = Compound Arithmetic op=OR ("复合运算")(w1656, w1649, w1659, w1658) -> (w1657:bool)
      }
      n864 = global read "全局1.vi" "枚举"() -> (w1452:enum16{"返回请求应答", "上传数据", "返回执行结果"})
      n865 = Equal?(x=w1452, y=enum16{"返回请求应答", "上传数据", "返回执行结果"}."上传数据") -> (x = y?=w1450:bool)
      n866 = case shown="真" w1450 {
        tunnel: w1449 -> [_ w1465]
        tunnel: ["" w1459] -> w1447
        frame False {
        }
        frame True {
          n867 = for {
            tunnel: w1465 -> [w1469] mode=indexing
            shift-right: [w1467] -> w1466
            shift-left: "" -> [w1468]
            n868 = Concatenate Strings(w1468, w1469) -> (w1467:string)
          }
          n869 = String Length(string=w1466) -> (length=w1460:i32)
          n870 = Quotient & Remainder(x=w1460, y=834) -> (floor(x/y)=w1462:i32)  [unwired: 1 out]
          n871 = Increment(x=w1462) -> (x+1=w1463:i32)
          n872 = Number To Decimal String(number=w1463) -> (decimal integer string=w1459:string)  [unwired: 1 in]
        }
      }
    }
    frame "操作日志" {
      n873 = global read "全局 小时数据发送次数.vi" "小时数据发送次数"() -> (w1870:i32)
      n874 = Less Or Equal?(x=w1870, y=1) -> (x <= y?=w1868:bool)
      n875 = case shown="真" w1868 {
        tunnel: w1879 -> [_ w1887]
        tunnel: w1878 -> [_ w1886]
        tunnel: w1877 -> [_ w1885]
        tunnel: w1876 -> [_ w1884]
        tunnel: w1875 -> [_ w1883]
        frame False {
        }
        frame True {
          n876 = while {
            tunnel: w1887 -> [w1907]
            tunnel: w1886 -> [w1906]
            tunnel: w1885 -> [w1905]
            tunnel: w1884 -> [w1904]
            tunnel: w1883 -> [w1903]
            shift-right: [w1889] -> _
            shift-left: "" -> [w1890]
            i -> [w1914]
            stop <- w1893 stop-if-true
            n877 = property on="小时数据发送次数" class="DigNum (严格)"() -> ("Value"=w1900:i32)  [unwired: 2 in, 2 out]
            n878 = property on="小时数据发送次数" class="DigNum (严格)"() -> ("Value"=w1899:i32)  [unwired: 2 in, 2 out]
            n879 = property on="小时数据发送次数" class="DigNum (严格)"() -> ("Value"=w1902:i32)  [unwired: 2 in, 2 out]
            n880 = property on="小时数据发送次数" class="DigNum (严格)"() -> ("Value"=w1898:i32)  [unwired: 2 in, 2 out]
            n881 = property on="小时数据发送次数" class="DigNum (严格)"() -> ("Value"=w1901:i32)  [unwired: 2 in, 2 out]
            n882 = Index Array(array=w1907, index (row)=w1898) -> (element=w1910:string[])  [unwired: 1 in]
            n883 = Index Array(array=w1906, index (row)=w1899) -> (element=w1909:string[])  [unwired: 1 in]
            n884 = Index Array(array=w1904, index (row)=w1901) -> (element=w1911:string[])  [unwired: 1 in]
            n885 = Index Array(array=w1903, index (row)=w1902) -> (element=w1912:string[])  [unwired: 1 in]
            n886 = global read "全局1.vi" "枚举"() -> (w1908:enum16{"返回请求应答", "上传数据", "返回执行结果"})
            n887 = Index Array(array=w1905, index (row)=w1900) -> (element=w1913:string[])  [unwired: 1 in]
            n888 = case shown="\"返回请求应答\", 默认" w1908 {
              tunnel: ["QnRtn=1" w1973 "ExeRtn=1"] -> w1888
              tunnel: w1909 -> [_ w1966 _]
              tunnel: w1910 -> [_ w1964 _]
              tunnel: w1911 -> [_ w1962 _]
              tunnel: w1912 -> [_ w1961 _]
              tunnel: w1913 -> [_ w1959 _]
              frame "返回请求应答", Default {
                w1944 = 0 ("包数")
                n889 = property on="包数" class="DigNum (严格)"("Value"=w1944) -> ()  [unwired: 2 in, 2 out]
                n890 = property on="总包数" class="DigNum (严格)"("Value"=w1944) -> ()  [unwired: 2 in, 2 out]
              }
              frame "上传数据" {
                n891 = property on="小时数据发送次数" class="DigNum (严格)"() -> ("Value"=w1947:i32)  [unwired: 2 in, 2 out]
                n892 = Increment(x=w1947) -> (x+1=w1946:i32)
                n893 = property on="小时数据发送次数" class="DigNum (严格)"("Value"=w1946) -> ()  [unwired: 2 in, 2 out]
                n894 = Index Array(array=w1961, index #1=0 ("索引"), index #2=2 ("索引")) -> (element #1=w1960:string, element #2=w1950:string)
                n895 = Index Array(array=w1966, index #1=0 ("索引"), index #2=2 ("索引")) -> (element #1=w1965:string, element #2=w1952:string)
                n896 = Index Array(array=w1959, index #1=0 ("索引"), index #2=2 ("索引")) -> (element #1=w1958:string, element #2=w1954:string)
                n897 = Index Array(array=w1962, index #1=0 ("索引"), index #2=2 ("索引")) -> (element #1=w1967:string, element #2=w1948:string)
                n898 = Index Array(array=w1964, index #1=0 ("索引"), index #2=2 ("索引")) -> (element #1=w1963:string, element #2=w1957:string)
                n899 = Empty String/Path?(string/path=w1950) -> (empty?=w1951:bool)
                n900 = Empty String/Path?(string/path=w1952) -> (empty?=w1953:bool)
                n901 = Empty String/Path?(string/path=w1948) -> (empty?=w1949:bool)
                n902 = case shown="假" w1953 {
                  tunnel: [w1998 ""] -> w1980
                  tunnel: w1952 -> [w1997 _]
                  tunnel: w1965 -> [w1996 _]
                  frame False {
                    # "氨氮"
                    n903 = call "规范时间戳.vi"("字符串"=w1996) -> ("result string"=w1999:string)  [unwired: 10 in]
                    n904 = Format Into String(format string="DataTime=%s;PolId=w21003,i11001-Info=//%s//;" ("格式字符串"), w1999, w1997) -> (resulting string=w1998:string)  [unwired: 2 in, 1 out]
                  }
                  frame True {
                  }
                }
                n905 = case shown="假" w1951 {
                  tunnel: [w1990 ""] -> w1975
                  tunnel: w1960 -> [w1992 _]
                  tunnel: w1950 -> [w1991 _]
                  frame False {
                    # "总氮"
                    n906 = call "规范时间戳.vi"("字符串"=w1992) -> ("result string"=w1994:string)  [unwired: 10 in]
                    n907 = Format Into String(format string="DataTime=%s;PolId=w21001,i11001-Info=//%s//;" ("格式字符串"), w1994, w1991) -> (resulting string=w1990:string)  [unwired: 2 in, 1 out]
                  }
                  frame True {
                  }
                }
                n908 = Empty String/Path?(string/path=w1954) -> (empty?=w1955:bool)
                n909 = case shown="假" w1949 {
                  tunnel: [w1987 ""] -> w1976
                  tunnel: w1967 -> [w1985 _]
                  tunnel: w1948 -> [w1984 _]
                  frame False {
                    # "总磷"
                    n910 = call "规范时间戳.vi"("字符串"=w1985) -> ("result string"=w1988:string)  [unwired: 10 in]
                    n911 = Format Into String(format string="DataTime=%s;PolId=w21011,i11001-Info=//%s//;" ("格式字符串"), w1988, w1984) -> (resulting string=w1987:string)  [unwired: 2 in, 1 out]
                  }
                  frame True {
                  }
                }
                n912 = case shown="假" w1955 {
                  tunnel: [w2006 ""] -> w1979
                  tunnel: w1958 -> [w2003 _]
                  tunnel: w1954 -> [w2002 _]
                  frame False {
                    # "系统日志"
                    n913 = call "规范时间戳.vi"("字符串"=w2003) -> ("result string"=w2005:string)  [unwired: 10 in]
                    n914 = Format Into String(format string="DataTime=%s;PolId=w00000,i21001-Info=//%s//;" ("格式字符串"), w2005, w2002) -> (resulting string=w2006:string)  [unwired: 2 in, 1 out]
                  }
                  frame True {
                  }
                }
                n915 = Empty String/Path?(string/path=w1957) -> (empty?=w1956:bool)
                n916 = case shown="假" w1956 {
                  tunnel: [w2010 ""] -> w1981
                  tunnel: w1963 -> [w2009 _]
                  tunnel: w1957 -> [w2008 _]
                  frame False {
                    # "高锰酸钾盐"
                    n917 = call "规范时间戳.vi"("字符串"=w2009) -> ("result string"=w2011:string)  [unwired: 10 in]
                    n918 = Format Into String(format string="DataTime=%s;PolId=w01019,i11001-Info=//%s//;" ("格式字符串"), w2011, w2008) -> (resulting string=w2010:string)  [unwired: 2 in, 1 out]
                  }
                  frame True {
                  }
                }
                n919 = Concatenate Strings(w1981, w1980, w1979, w1976, w1975) -> (w1973:string)
              }
              frame "返回执行结果" {
                w2014 = 0 ("包数")
                n920 = property on="包数" class="DigNum (严格)"("Value"=w2014) -> ()  [unwired: 2 in, 2 out]
                n921 = property on="总包数" class="DigNum (严格)"("Value"=w2014) -> ()  [unwired: 2 in, 2 out]
              }
            }
            n922 = global read "全局 数据数组大小.vi" "数据数组大小"() -> (w1923:i32)
            n923 = global read "全局1.vi" "枚举"() -> (w1916:enum16{"返回请求应答", "上传数据", "返回执行结果"})
            n924 = global read "全局1.vi" "枚举"() -> (w1920:enum16{"返回请求应答", "上传数据", "返回执行结果"})
            n925 = Increment(x=w1914) -> (x+1=w1922:i32)
            n926 = Equal?(x=w1916, y=enum16{"返回请求应答", "上传数据", "返回执行结果"}."返回执行结果") -> (x = y?=w1915:bool)
            n927 = Equal?(x=w1920, y=enum16{"返回请求应答", "上传数据", "返回执行结果"}."返回请求应答") -> (x = y?=w1918:bool)
            n928 = Greater Or Equal?(x=w1922, y=w1923) -> (x >= y?=w1921:bool)
            n929 = Compound Arithmetic op=OR ("复合运算")(w1915, w1918, w1921) -> (w1893:bool)
            n930 = call <vilib>:"Boolean Crossing PtByPt.vi"("direction"=enum16{"either", "false-true", "true-false"}."false-true", "input"=w1893) -> ("crossing"=w1894:bool)  [unwired: 1 in]
            n931 = case shown="真" w1894 {
              frame False {
              }
              frame True {
                n932 = property on="包数" class="DigNum (严格)"() -> ("Value"=w1943:i32)  [unwired: 2 in, 2 out]
                n933 = Increment(x=w1943) -> (x+1=w1942:i32)
                n934 = property on="总包数" class="DigNum (严格)"("Value"=w1942) -> ()  [unwired: 2 in, 2 out]
              }
            }
            n935 = Concatenate Strings(w1890, w1888) -> (w1892:string)
            n936 = String Length(string=w1892) -> (length=w1897:i32)
            n937 = Greater Or Equal?(x=w1897, y=890) -> (x >= y?=w1891:bool)
            n938 = case shown="真" w1891 {
              tunnel: w1892 -> [w1927 w1931]
              tunnel: [w1927 w1930] -> w1889
              tunnel: w1888 -> [_ w1932]
              frame False {
                n939 = global read "全局 小时数据发送次数.vi" "小时数据发送次数"() -> (w1924:i32)
                n940 = global read "全局 数据数组大小.vi" "数据数组大小"() -> (w1925:i32)
                n941 = Equal?(x=w1924, y=w1925) -> (x = y?=w1926:bool)
                n942 = case shown="假" w1926 {
                  frame False {
                  }
                  frame True {
                    n943 = property on="包数" class="DigNum (严格)"() -> ("Value"=w1929:i32)  [unwired: 2 in, 2 out]
                    n944 = Increment(x=w1929) -> (x+1=w1928:i32)
                    n945 = property on="包数" class="DigNum (严格)"("Value"=w1928) -> ()  [unwired: 2 in, 2 out]
                  }
                }
              }
              frame True {
                n946 = global read "全局 小时数据发送次数.vi" "小时数据发送次数"() -> (w1934:i32)
                n947 = global read "全局 数据数组大小.vi" "数据数组大小"() -> (w1933:i32)
                n948 = property on="小时数据发送次数" class="DigNum (严格)"() -> ("Value"=w1938:i32)  [unwired: 2 in, 2 out]
                n949 = Increment(x=w1938) -> (x+1=w1937:i32)
                n950 = Equal?(x=w1934, y=w1933) -> (x = y?=w1935:bool)
                n951 = case shown="假" w1935 {
                  tunnel: w1932 -> [w1940 _]
                  tunnel: [w1940 w1941] -> w1930
                  tunnel: w1931 -> [_ w1941]
                  frame False {
                  }
                  frame True {
                  }
                }
                n952 = property on="小时数据发送次数" class="DigNum (严格)"("Value"=w1937) -> ()  [unwired: 2 in, 2 out]
                n953 = property on="包数" class="DigNum (严格)"() -> ("Value"=w1939:i32)  [unwired: 2 in, 2 out]
                n954 = Increment(x=w1939) -> (x+1=w1936:i32)
                n955 = property on="包数" class="DigNum (严格)"("Value"=w1936) -> ()  [unwired: 2 in, 2 out]
              }
            }
          }
        }
      }
      n956 = while {
        shift-right: [w2040] -> _
        shift-left: "" -> [w2044]
        tunnel: [w2040] -> w1880
        tunnel: w1878 -> [w2033]
        tunnel: w1879 -> [w2029]
        tunnel: w1876 -> [w2025]
        tunnel: w1875 -> [w2024]
        tunnel: w1877 -> [w2020]
        i -> [w2043]
        stop <- w2045 stop-if-true
        n957 = global read "全局 小时数据发送次数.vi" "小时数据发送次数"() -> (w2030:i32)
        n958 = global read "全局 小时数据发送次数.vi" "小时数据发送次数"() -> (w2032:i32)
        n959 = global read "全局 小时数据发送次数.vi" "小时数据发送次数"() -> (w2027:i32)
        n960 = global read "全局 小时数据发送次数.vi" "小时数据发送次数"() -> (w2026:i32)
        n961 = global read "全局 小时数据发送次数.vi" "小时数据发送次数"() -> (w2021:i32)
        n962 = Index Array(array=w2029, index (row)=w2030) -> (element=w2028:string[])  [unwired: 1 in]
        n963 = Index Array(array=w2033, index (row)=w2032) -> (element=w2031:string[])  [unwired: 1 in]
        n964 = Index Array(array=w2025, index (row)=w2027) -> (element=w2023:string[])  [unwired: 1 in]
        n965 = Index Array(array=w2024, index (row)=w2026) -> (element=w2022:string[])  [unwired: 1 in]
        n966 = global read "全局1.vi" "枚举"() -> (w2056:enum16{"返回请求应答", "上传数据", "返回执行结果"})
        n967 = Index Array(array=w2020, index (row)=w2021) -> (element=w2019:string[])  [unwired: 1 in]
        n968 = case shown="\"上传数据\"" w2056 {
          tunnel: ["QnRtn=1" w2112 "ExeRtn=1"] -> w2042
          tunnel: w2031 -> [_ w2103 _]
          tunnel: w2028 -> [_ w2101 _]
          tunnel: w2023 -> [_ w2099 _]
          tunnel: w2022 -> [_ w2098 _]
          tunnel: w2019 -> [_ w2096 _]
          frame "返回请求应答", Default {
            n969 = global read "全局 数据数组大小.vi" "数据数组大小"() -> (w2082:i32)
            n970 = global write "全局1.vi" "枚举"(enum16{"返回请求应答", "上传数据", "返回执行结果"}."上传数据" ("枚举")) -> ()
            n971 = Equal To 0?(x=w2082) -> (x = 0?=w2081:bool)
            n972 = case shown="真" w2081 {
              frame False {
              }
              frame True {
                n973 = global read "全局 小时数据发送次数.vi" "小时数据发送次数"() -> (w2084:i32)
                n974 = Increment(x=w2084) -> (x+1=w2083:i32)
                n975 = global write "全局 小时数据发送次数.vi" "小时数据发送次数"(w2083) -> ()
              }
            }
            n976 = property on="当前包数" class="DigNum (严格)"("Value"=0 ("当前包数")) -> ()  [unwired: 2 in, 2 out]
          }
          frame "上传数据" {
            n977 = global read "全局 小时数据发送次数.vi" "小时数据发送次数"() -> (w2111:i32)
            n978 = Increment(x=w2111) -> (x+1=w2110:i32)
            n979 = global write "全局 小时数据发送次数.vi" "小时数据发送次数"(w2110) -> ()
            n980 = Index Array(array=w2098, index #1=0 ("索引"), index #2=2 ("索引")) -> (element #1=w2097:string, element #2=w2087:string)
            n981 = Index Array(array=w2103, index #1=0 ("索引"), index #2=2 ("索引")) -> (element #1=w2102:string, element #2=w2089:string)
            n982 = Index Array(array=w2096, index #1=0 ("索引"), index #2=2 ("索引")) -> (element #1=w2095:string, element #2=w2091:string)
            n983 = Index Array(array=w2099, index #1=0 ("索引"), index #2=2 ("索引")) -> (element #1=w2104:string, element #2=w2085:string)
            n984 = Index Array(array=w2101, index #1=0 ("索引"), index #2=2 ("索引")) -> (element #1=w2100:string, element #2=w2094:string)
            n985 = Empty String/Path?(string/path=w2087) -> (empty?=w2088:bool)
            n986 = Empty String/Path?(string/path=w2089) -> (empty?=w2090:bool)
            n987 = Empty String/Path?(string/path=w2085) -> (empty?=w2086:bool)
            n988 = case shown="假" w2090 {
              tunnel: [w2137 ""] -> w2119
              tunnel: w2089 -> [w2136 _]
              tunnel: w2102 -> [w2135 _]
              frame False {
                # "氨氮"
                n989 = call "规范时间戳.vi"("字符串"=w2135) -> ("result string"=w2138:string)  [unwired: 10 in]
                n990 = Format Into String(format string="DataTime=%s;PolId=w21003,i11001-Info=//%s//;" ("格式字符串"), w2138, w2136) -> (resulting string=w2137:string)  [unwired: 2 in, 1 out]
              }
              frame True {
              }
            }
            n991 = case shown="假" w2088 {
              tunnel: [w2129 ""] -> w2114
              tunnel: w2097 -> [w2131 _]
              tunnel: w2087 -> [w2130 _]
              frame False {
                # "总氮"
                n992 = call "规范时间戳.vi"("字符串"=w2131) -> ("result string"=w2133:string)  [unwired: 10 in]
                n993 = Format Into String(format string="DataTime=%s;PolId=w21001,i11001-Info=//%s//;" ("格式字符串"), w2133, w2130) -> (resulting string=w2129:string)  [unwired: 2 in, 1 out]
              }
              frame True {
              }
            }
            n994 = Empty String/Path?(string/path=w2091) -> (empty?=w2092:bool)
            n995 = case shown="假" w2086 {
              tunnel: [w2126 ""] -> w2115
              tunnel: w2104 -> [w2124 _]
              tunnel: w2085 -> [w2123 _]
              frame False {
                # "总磷"
                n996 = call "规范时间戳.vi"("字符串"=w2124) -> ("result string"=w2127:string)  [unwired: 10 in]
                n997 = Format Into String(format string="DataTime=%s;PolId=w21011,i11001-Info=//%s//;" ("格式字符串"), w2127, w2123) -> (resulting string=w2126:string)  [unwired: 2 in, 1 out]
              }
              frame True {
              }
            }
            n998 = case shown="假" w2092 {
              tunnel: [w2145 ""] -> w2118
              tunnel: w2095 -> [w2142 _]
              tunnel: w2091 -> [w2141 _]
              frame False {
                # "系统日志"
                n999 = call "规范时间戳.vi"("字符串"=w2142) -> ("result string"=w2144:string)  [unwired: 10 in]
                n1000 = Format Into String(format string="DataTime=%s;PolId=w00000,i21001-Info=//%s//;" ("格式字符串"), w2144, w2141) -> (resulting string=w2145:string)  [unwired: 2 in, 1 out]
              }
              frame True {
              }
            }
            n1001 = Empty String/Path?(string/path=w2094) -> (empty?=w2093:bool)
            n1002 = case shown="假" w2093 {
              tunnel: [w2149 ""] -> w2120
              tunnel: w2100 -> [w2148 _]
              tunnel: w2094 -> [w2147 _]
              frame False {
                # "高锰酸钾盐"
                n1003 = call "规范时间戳.vi"("字符串"=w2148) -> ("result string"=w2150:string)  [unwired: 10 in]
                n1004 = Format Into String(format string="DataTime=%s;PolId=w01019,i11001-Info=//%s//;" ("格式字符串"), w2150, w2147) -> (resulting string=w2149:string)  [unwired: 2 in, 1 out]
              }
              frame True {
              }
            }
            n1005 = Concatenate Strings(w2120, w2119, w2118, w2115, w2114) -> (w2112:string)
          }
          frame "返回执行结果" {
            n1006 = global write "全局1.vi" "枚举"(enum16{"返回请求应答", "上传数据", "返回执行结果"}."返回请求应答" ("枚举")) -> ()
            n1007 = property on="当前包数" class="DigNum (严格)"("Value"=0 ("当前包数")) -> ()  [unwired: 2 in, 2 out]
          }
        }
        n1008 = global read "全局 小时数据发送次数.vi" "小时数据发送次数"() -> (w2050:i32)
        n1009 = global read "全局 数据数组大小.vi" "数据数组大小"() -> (w2051:i32)
        n1010 = Greater Or Equal?(x=w2050, y=w2051) -> (x >= y?=w2049:bool)
        n1011 = Concatenate Strings(w2044, w2042) -> (w2041:string)
        n1012 = String Length(string=w2041) -> (length=w2052:i32)
        n1013 = Greater Or Equal?(x=w2052, y=890) -> (x >= y?=w2055:bool)
        n1014 = case shown="真" w2055 {
          tunnel: [w2057 TRUE ("值")] -> w2054
          tunnel: [w2058 w2070] -> w2040
          tunnel: w2044 -> [_ w2071]
          tunnel: w2041 -> [w2058 w2069]
          frame False {
            n1015 = global read "全局 小时数据发送次数.vi" "小时数据发送次数"() -> (w2059:i32)
            n1016 = global read "全局 数据数组大小.vi" "数据数组大小"() -> (w2060:i32)
            n1017 = Equal?(x=w2059, y=w2060) -> (x = y?=w2061:bool)
            n1018 = case shown="假" w2061 {
              tunnel: [_ TRUE ("值")] -> w2057
              frame False {
              }
              frame True {
                n1019 = property on="当前包数" class="DigNum (严格)"() -> ("Value"=w2063:i32)  [unwired: 2 in, 2 out]
                n1020 = Increment(x=w2063) -> (x+1=w2062:i32)
                n1021 = property on="当前包数" class="DigNum (严格)"("Value"=w2062) -> ()  [unwired: 2 in, 2 out]
              }
            }
          }
          frame True {
            n1022 = property on="当前包数" class="DigNum (严格)"() -> ("Value"=w2066:i32)  [unwired: 2 in, 2 out]
            n1023 = global read "全局 小时数据发送次数.vi" "小时数据发送次数"() -> (w2073:i32)
            n1024 = global read "全局 小时数据发送次数.vi" "小时数据发送次数"() -> (w2068:i32)
            n1025 = global read "全局 数据数组大小.vi" "数据数组大小"() -> (w2074:i32)
            n1026 = Increment(x=w2066) -> (x+1=w2065:i32)
            n1027 = property on="当前包数" class="DigNum (严格)"("Value"=w2065) -> ()  [unwired: 2 in, 2 out]
            n1028 = Equal?(x=w2073, y=w2074) -> (x = y?=w2072:bool)
            n1029 = Decrement(x=w2068) -> (x-1=w2067:i32)
            n1030 = case shown="假" w2072 {
              tunnel: w2071 -> [w2076 _]
              tunnel: [w2076 w2077] -> w2070
              tunnel: w2069 -> [_ w2077]
              frame False {
              }
              frame True {
              }
            }
            n1031 = global write "全局 小时数据发送次数.vi" "小时数据发送次数"(w2067) -> ()
          }
        }
        n1032 = global read "全局 数据数组大小.vi" "数据数组大小"() -> (w2046:i32)
        n1033 = global read "全局1.vi" "枚举"() -> (w2039:enum16{"返回请求应答", "上传数据", "返回执行结果"})
        n1034 = global read "全局1.vi" "枚举"() -> (w2035:enum16{"返回请求应答", "上传数据", "返回执行结果"})
        n1035 = Increment(x=w2043) -> (x+1=w2047:i32)
        n1036 = Equal?(x=w2039, y=enum16{"返回请求应答", "上传数据", "返回执行结果"}."返回请求应答") -> (x = y?=w2037:bool)
        n1037 = Greater Or Equal?(x=w2047, y=w2046) -> (x >= y?=w2048:bool)
        n1038 = Equal?(x=w2035, y=enum16{"返回请求应答", "上传数据", "返回执行结果"}."返回执行结果") -> (x = y?=w2034:bool)
        n1039 = Compound Arithmetic op=OR ("复合运算")(w2049, w2054, w2037, w2048, w2034) -> (w2045:bool)
      }
      n1040 = global read "全局1.vi" "枚举"() -> (w1874:enum16{"返回请求应答", "上传数据", "返回执行结果"})
      n1041 = Equal?(x=w1874, y=enum16{"返回请求应答", "上传数据", "返回执行结果"}."上传数据") -> (x = y?=w1872:bool)
      n1042 = case shown="真" w1872 {
        tunnel: ["" w2017] -> w1871
        frame False {
        }
        frame True {
          n1043 = property on="总包数" class="DigNum (严格)"() -> ("Value"=w2018:i32)  [unwired: 2 in, 2 out]
          n1044 = Number To Decimal String(number=w2018) -> (decimal integer string=w2017:string)  [unwired: 1 in]
        }
      }
    }
    frame "报警信息" {
      n1045 = while {
        shift-right: [w2320] -> _
        shift-left: "" -> [w2324]
        tunnel: [w2320] -> w2166
        tunnel: w2164 -> [w2313]
        tunnel: w2165 -> [w2309]
        tunnel: w2162 -> [w2305]
        tunnel: w2161 -> [w2304]
        tunnel: w2163 -> [w2300]
        i -> [w2323]
        stop <- w2325 stop-if-true
        n1046 = global read "全局 小时数据发送次数.vi" "小时数据发送次数"() -> (w2310:i32)
        n1047 = global read "全局 小时数据发送次数.vi" "小时数据发送次数"() -> (w2312:i32)
        n1048 = global read "全局 小时数据发送次数.vi" "小时数据发送次数"() -> (w2307:i32)
        n1049 = global read "全局 小时数据发送次数.vi" "小时数据发送次数"() -> (w2306:i32)
        n1050 = global read "全局 小时数据发送次数.vi" "小时数据发送次数"() -> (w2301:i32)
        n1051 = Index Array(array=w2309, index (row)=w2310) -> (element=w2308:string[])  [unwired: 1 in]
        n1052 = Index Array(array=w2313, index (row)=w2312) -> (element=w2311:string[])  [unwired: 1 in]
        n1053 = Index Array(array=w2305, index (row)=w2307) -> (element=w2303:string[])  [unwired: 1 in]
        n1054 = Index Array(array=w2304, index (row)=w2306) -> (element=w2302:string[])  [unwired: 1 in]
        n1055 = global read "全局1.vi" "枚举"() -> (w2336:enum16{"返回请求应答", "上传数据", "返回执行结果"})
        n1056 = Index Array(array=w2300, index (row)=w2301) -> (element=w2299:string[])  [unwired: 1 in]
        n1057 = case shown="\"上传数据\"" w2336 {
          tunnel: ["QnRtn=1" w2392 "ExeRtn=1"] -> w2322
          tunnel: w2311 -> [_ w2383 _]
          tunnel: w2308 -> [_ w2381 _]
          tunnel: w2303 -> [_ w2379 _]
          tunnel: w2302 -> [_ w2378 _]
          tunnel: w2299 -> [_ w2376 _]
          frame "返回请求应答", Default {
            w2358 = 0 ("当前包数")
            n1058 = global read "全局 数据数组大小.vi" "数据数组大小"() -> (w2362:i32)
            n1059 = global write "全局1.vi" "枚举"(enum16{"返回请求应答", "上传数据", "返回执行结果"}."上传数据" ("枚举")) -> ()
            n1060 = Equal To 0?(x=w2362) -> (x = 0?=w2361:bool)
            n1061 = case shown="真" w2361 {
              frame False {
              }
              frame True {
                n1062 = global read "全局 小时数据发送次数.vi" "小时数据发送次数"() -> (w2364:i32)
                n1063 = Increment(x=w2364) -> (x+1=w2363:i32)
                n1064 = global write "全局 小时数据发送次数.vi" "小时数据发送次数"(w2363) -> ()
              }
            }
            n1065 = property on="总包数" class="DigNum (严格)"("Value"=w2358) -> ()  [unwired: 2 in, 2 out]
            n1066 = property on="当前包数" class="DigNum (严格)"("Value"=w2358) -> ()  [unwired: 2 in, 2 out]
          }
          frame "上传数据" {
            n1067 = global read "全局 小时数据发送次数.vi" "小时数据发送次数"() -> (w2391:i32)
            n1068 = Increment(x=w2391) -> (x+1=w2390:i32)
            n1069 = global write "全局 小时数据发送次数.vi" "小时数据发送次数"(w2390) -> ()
            n1070 = Index Array(array=w2378, index #1=0 ("索引"), index #2=2 ("索引")) -> (element #1=w2377:string, element #2=w2367:string)
            n1071 = Index Array(array=w2383, index #1=0 ("索引"), index #2=2 ("索引")) -> (element #1=w2382:string, element #2=w2369:string)
            n1072 = Empty String/Path?(string/path=w2369) -> (empty?=w2370:bool)
            n1073 = Index Array(array=w2376, index #1=0 ("索引"), index #2=2 ("索引")) -> (element #1=w2375:string, element #2=w2371:string)
            n1074 = Index Array(array=w2379, index #1=0 ("索引"), index #2=2 ("索引")) -> (element #1=w2384:string, element #2=w2365:string)
            n1075 = Index Array(array=w2381, index #1=0 ("索引"), index #2=2 ("索引")) -> (element #1=w2380:string, element #2=w2374:string)
            n1076 = Empty String/Path?(string/path=w2367) -> (empty?=w2368:bool)
            n1077 = case shown="假" w2370 {
              tunnel: [w2417 ""] -> w2399
              tunnel: w2369 -> [_ _]
              tunnel: w2382 -> [w2416 _]
              frame False {
                w2415 = "0" ("输入 2")
                # "氨氮"
                n1078 = call "规范时间戳.vi"("字符串"=w2416) -> ("result string"=w2418:string)  [unwired: 10 in]
                n1079 = Format Into String(format string="DataTime=%s;PolId=w21003,i12001-Info=%s,i12031-Info=%s;" ("格式字符串"), w2418, w2415, w2415) -> (resulting string=w2417:string)  [unwired: 2 in, 1 out]
              }
              frame True {
              }
            }
            n1080 = Empty String/Path?(string/path=w2371) -> (empty?=w2372:bool)
            n1081 = Empty String/Path?(string/path=w2374) -> (empty?=w2373:bool)
            n1082 = Empty String/Path?(string/path=w2365) -> (empty?=w2366:bool)
            n1083 = case shown="假" w2372 {
              tunnel: [w2425 ""] -> w2398
              tunnel: w2375 -> [w2422 _]
              tunnel: w2371 -> [_ _]
              frame False {
                w2421 = "0" ("输入 2")
                # "系统日志"
                n1084 = call "规范时间戳.vi"("字符串"=w2422) -> ("result string"=w2424:string)  [unwired: 10 in]
                n1085 = Format Into String(format string="DataTime=%s;PolId=w00000,i22001-Info=%s,i22003-Info=%s;" ("格式字符串"), w2424, w2421, w2421) -> (resulting string=w2425:string)  [unwired: 2 in, 1 out]
              }
              frame True {
              }
            }
            n1086 = case shown="假" w2368 {
              tunnel: [w2410 ""] -> w2394
              tunnel: w2377 -> [w2411 _]
              tunnel: w2367 -> [_ _]
              frame False {
                w2409 = "0" ("输入 2")
                # "总氮"
                n1087 = call "规范时间戳.vi"("字符串"=w2411) -> ("result string"=w2413:string)  [unwired: 10 in]
                n1088 = Format Into String(format string="DataTime=%s;PolId=w21001,i12001-Info=%s,i12031-Info=%s;" ("格式字符串"), w2413, w2409, w2409) -> (resulting string=w2410:string)  [unwired: 2 in, 1 out]
              }
              frame True {
              }
            }
            n1089 = case shown="假" w2366 {
              tunnel: [w2407 ""] -> w2395
              tunnel: w2384 -> [w2405 _]
              tunnel: w2365 -> [_ _]
              frame False {
                w2403 = "0" ("输入 2")
                # "总磷"
                n1090 = call "规范时间戳.vi"("字符串"=w2405) -> ("result string"=w2404:string)  [unwired: 10 in]
                n1091 = Format Into String(format string="DataTime=%s;PolId=w21011,i12001-Info=%s,i12031-Info=%s;" ("格式字符串"), w2404, w2403, w2403) -> (resulting string=w2407:string)  [unwired: 2 in, 1 out]
              }
              frame True {
              }
            }
            n1092 = case shown="假" w2373 {
              tunnel: [w2430 ""] -> w2400
              tunnel: w2380 -> [w2429 _]
              tunnel: w2374 -> [_ _]
              frame False {
                # "高锰酸钾盐"
                n1093 = call "规范时间戳.vi"("字符串"=w2429) -> ("result string"=w2431:string)  [unwired: 10 in]
                n1094 = Format Into String(format string="DataTime=%s;PolId=w01019,i12001-Info=%s,i12031-Info=%s;" ("格式字符串"), w2431, "0" ("输入 2"), "0" ("输入 3")) -> (resulting string=w2430:string)  [unwired: 2 in, 1 out]
              }
              frame True {
              }
            }
            n1095 = Concatenate Strings(w2400, w2399, w2398, w2395, w2394) -> (w2392:string)
          }
          frame "返回执行结果" {
            w2434 = 0 ("当前包数")
            n1096 = global write "全局1.vi" "枚举"(enum16{"返回请求应答", "上传数据", "返回执行结果"}."返回请求应答" ("枚举")) -> ()
            n1097 = property on="当前包数" class="DigNum (严格)"("Value"=w2434) -> ()  [unwired: 2 in, 2 out]
            n1098 = property on="总包数" class="DigNum (严格)"("Value"=w2434) -> ()  [unwired: 2 in, 2 out]
          }
        }
        n1099 = global read "全局 小时数据发送次数.vi" "小时数据发送次数"() -> (w2330:i32)
        n1100 = global read "全局 数据数组大小.vi" "数据数组大小"() -> (w2331:i32)
        n1101 = Greater Or Equal?(x=w2330, y=w2331) -> (x >= y?=w2329:bool)
        n1102 = Concatenate Strings(w2324, w2322) -> (w2321:string)
        n1103 = String Length(string=w2321) -> (length=w2332:i32)
        n1104 = Greater Or Equal?(x=w2332, y=890) -> (x >= y?=w2335:bool)
        n1105 = case shown="假" w2335 {
          tunnel: [w2337 TRUE ("值")] -> w2334
          tunnel: [w2338 w2350] -> w2320
          tunnel: w2324 -> [_ w2351]
          tunnel: w2321 -> [w2338 w2349]
          frame False {
            n1106 = global read "全局 小时数据发送次数.vi" "小时数据发送次数"() -> (w2339:i32)
            n1107 = global read "全局 数据数组大小.vi" "数据数组大小"() -> (w2340:i32)
            n1108 = Equal?(x=w2339, y=w2340) -> (x = y?=w2341:bool)
            n1109 = case shown="真" w2341 {
              tunnel: [_ TRUE ("值")] -> w2337
              frame False {
              }
              frame True {
                n1110 = property on="当前包数" class="DigNum (严格)"() -> ("Value"=w2343:i32)  [unwired: 2 in, 2 out]
                n1111 = Increment(x=w2343) -> (x+1=w2342:i32)
                n1112 = property on="当前包数" class="DigNum (严格)"("Value"=w2342) -> ()  [unwired: 2 in, 2 out]
              }
            }
          }
          frame True {
            n1113 = property on="当前包数" class="DigNum (严格)"() -> ("Value"=w2346:i32)  [unwired: 2 in, 2 out]
            n1114 = Increment(x=w2346) -> (x+1=w2345:i32)
            n1115 = property on="当前包数" class="DigNum (严格)"("Value"=w2345) -> ()  [unwired: 2 in, 2 out]
            n1116 = global read "全局 小时数据发送次数.vi" "小时数据发送次数"() -> (w2348:i32)
            n1117 = global read "全局 小时数据发送次数.vi" "小时数据发送次数"() -> (w2353:i32)
            n1118 = global read "全局 数据数组大小.vi" "数据数组大小"() -> (w2354:i32)
            n1119 = Equal?(x=w2353, y=w2354) -> (x = y?=w2352:bool)
            n1120 = Decrement(x=w2348) -> (x-1=w2347:i32)
            n1121 = case shown="假" w2352 {
              tunnel: w2351 -> [w2356 _]
              tunnel: [w2356 w2357] -> w2350
              tunnel: w2349 -> [_ w2357]
              frame False {
              }
              frame True {
              }
            }
            n1122 = global write "全局 小时数据发送次数.vi" "小时数据发送次数"(w2347) -> ()
          }
        }
        n1123 = global read "全局 数据数组大小.vi" "数据数组大小"() -> (w2326:i32)
        n1124 = global read "全局1.vi" "枚举"() -> (w2319:enum16{"返回请求应答", "上传数据", "返回执行结果"})
        n1125 = global read "全局1.vi" "枚举"() -> (w2315:enum16{"返回请求应答", "上传数据", "返回执行结果"})
        n1126 = Increment(x=w2323) -> (x+1=w2327:i32)
        n1127 = Equal?(x=w2319, y=enum16{"返回请求应答", "上传数据", "返回执行结果"}."返回请求应答") -> (x = y?=w2317:bool)
        n1128 = Greater Or Equal?(x=w2327, y=w2326) -> (x >= y?=w2328:bool)
        n1129 = Equal?(x=w2315, y=enum16{"返回请求应答", "上传数据", "返回执行结果"}."返回执行结果") -> (x = y?=w2314:bool)
        n1130 = Compound Arithmetic op=OR ("复合运算")(w2329, w2334, w2317, w2328, w2314) -> (w2325:bool)
      }
      n1131 = while {
        tunnel: w2165 -> [w2190]
        tunnel: w2164 -> [w2189]
        tunnel: w2163 -> [w2188]
        tunnel: w2162 -> [w2187]
        tunnel: w2161 -> [w2186]
        shift-right: [w2173] -> _
        shift-left: "" -> [w2172]
        i -> [w2197]
        stop <- w2174 stop-if-true
        n1132 = property on="小时数据发送次数" class="DigNum (严格)"() -> ("Value"=w2183:i32)  [unwired: 2 in, 2 out]
        n1133 = property on="小时数据发送次数" class="DigNum (严格)"() -> ("Value"=w2182:i32)  [unwired: 2 in, 2 out]
        n1134 = property on="小时数据发送次数" class="DigNum (严格)"() -> ("Value"=w2185:i32)  [unwired: 2 in, 2 out]
        n1135 = property on="小时数据发送次数" class="DigNum (严格)"() -> ("Value"=w2181:i32)  [unwired: 2 in, 2 out]
        n1136 = property on="小时数据发送次数" class="DigNum (严格)"() -> ("Value"=w2184:i32)  [unwired: 2 in, 2 out]
        n1137 = Index Array(array=w2190, index (row)=w2181) -> (element=w2193:string[])  [unwired: 1 in]
        n1138 = Index Array(array=w2189, index (row)=w2182) -> (element=w2192:string[])  [unwired: 1 in]
        n1139 = Index Array(array=w2187, index (row)=w2184) -> (element=w2194:string[])  [unwired: 1 in]
        n1140 = Index Array(array=w2186, index (row)=w2185) -> (element=w2195:string[])  [unwired: 1 in]
        n1141 = global read "全局1.vi" "枚举"() -> (w2191:enum16{"返回请求应答", "上传数据", "返回执行结果"})
        n1142 = Index Array(array=w2188, index (row)=w2183) -> (element=w2196:string[])  [unwired: 1 in]
        n1143 = case shown="\"返回请求应答\", 默认" w2191 {
          tunnel: ["QnRtn=1" w2256 "ExeRtn=1"] -> w2171
          tunnel: w2192 -> [_ w2249 _]
          tunnel: w2193 -> [_ w2247 _]
          tunnel: w2194 -> [_ w2245 _]
          tunnel: w2195 -> [_ w2244 _]
          tunnel: w2196 -> [_ w2242 _]
          frame "返回请求应答", Default {
            w2227 = 0 ("包数")
            n1144 = property on="包数" class="DigNum (严格)"("Value"=w2227) -> ()  [unwired: 2 in, 2 out]
            n1145 = property on="总包数" class="DigNum (严格)"("Value"=w2227) -> ()  [unwired: 2 in, 2 out]
          }
          frame "上传数据" {
            n1146 = property on="小时数据发送次数" class="DigNum (严格)"() -> ("Value"=w2230:i32)  [unwired: 2 in, 2 out]
            n1147 = Increment(x=w2230) -> (x+1=w2229:i32)
            n1148 = property on="小时数据发送次数" class="DigNum (严格)"("Value"=w2229) -> ()  [unwired: 2 in, 2 out]
            n1149 = Index Array(array=w2244, index #1=0 ("索引"), index #2=2 ("索引")) -> (element #1=w2243:string, element #2=w2233:string)
            n1150 = Index Array(array=w2249, index #1=0 ("索引"), index #2=2 ("索引")) -> (element #1=w2248:string, element #2=w2235:string)
            n1151 = Index Array(array=w2242, index #1=0 ("索引"), index #2=2 ("索引")) -> (element #1=w2241:string, element #2=w2237:string)
            n1152 = Index Array(array=w2245, index #1=0 ("索引"), index #2=2 ("索引")) -> (element #1=w2250:string, element #2=w2231:string)
            n1153 = Index Array(array=w2247, index #1=0 ("索引"), index #2=2 ("索引")) -> (element #1=w2246:string, element #2=w2240:string)
            n1154 = Empty String/Path?(string/path=w2233) -> (empty?=w2234:bool)
            n1155 = Empty String/Path?(string/path=w2235) -> (empty?=w2236:bool)
            n1156 = Empty String/Path?(string/path=w2231) -> (empty?=w2232:bool)
            n1157 = case shown="假" w2236 {
              tunnel: [w2281 ""] -> w2263
              tunnel: w2235 -> [_ _]
              tunnel: w2248 -> [w2280 _]
              frame False {
                w2279 = "0" ("输入 2")
                # "氨氮"
                n1158 = call "规范时间戳.vi"("字符串"=w2280) -> ("result string"=w2282:string)  [unwired: 10 in]
                n1159 = Format Into String(format string="DataTime=%s;PolId=w21003,i12001-Info=%s,i12031-Info=%s;" ("格式字符串"), w2282, w2279, w2279) -> (resulting string=w2281:string)  [unwired: 2 in, 1 out]
              }
              frame True {
              }
            }
            n1160 = case shown="假" w2232 {
              tunnel: [w2270 ""] -> w2259
              tunnel: w2250 -> [w2268 _]
              tunnel: w2231 -> [_ _]
              frame False {
                w2267 = "0" ("输入 2")
                # "总磷"
                n1161 = call "规范时间戳.vi"("字符串"=w2268) -> ("result string"=w2271:string)  [unwired: 10 in]
                n1162 = Format Into String(format string="DataTime=%s;PolId=w21011,i12001-Info=%s,i12031-Info=%s;" ("格式字符串"), w2271, w2267, w2267) -> (resulting string=w2270:string)  [unwired: 2 in, 1 out]
              }
              frame True {
              }
            }
            n1163 = case shown="假" w2234 {
              tunnel: [w2274 ""] -> w2258
              tunnel: w2243 -> [w2275 _]
              tunnel: w2233 -> [_ _]
              frame False {
                w2273 = "0" ("输入 2")
                # "总氮"
                n1164 = call "规范时间戳.vi"("字符串"=w2275) -> ("result string"=w2277:string)  [unwired: 10 in]
                n1165 = Format Into String(format string="DataTime=%s;PolId=w21001,i12001-Info=%s,i12031-Info=%s;" ("格式字符串"), w2277, w2273, w2273) -> (resulting string=w2274:string)  [unwired: 2 in, 1 out]
              }
              frame True {
              }
            }
            n1166 = Empty String/Path?(string/path=w2237) -> (empty?=w2238:bool)
            n1167 = case shown="假" w2238 {
              tunnel: [w2289 ""] -> w2262
              tunnel: w2241 -> [w2286 _]
              tunnel: w2237 -> [_ _]
              frame False {
                w2285 = "0" ("输入 2")
                # "系统日志"
                n1168 = call "规范时间戳.vi"("字符串"=w2286) -> ("result string"=w2288:string)  [unwired: 10 in]
                n1169 = Format Into String(format string="DataTime=%s;PolId=w00000,i22001-Info=%s,i22003-Info=%s;" ("格式字符串"), w2288, w2285, w2285) -> (resulting string=w2289:string)  [unwired: 2 in, 1 out]
              }
              frame True {
              }
            }
            n1170 = Empty String/Path?(string/path=w2240) -> (empty?=w2239:bool)
            n1171 = case shown="假" w2239 {
              tunnel: [w2293 ""] -> w2264
              tunnel: w2246 -> [w2292 _]
              tunnel: w2240 -> [_ _]
              frame False {
                w2291 = "0" ("输入 2")
                # "高锰酸钾盐"
                n1172 = call "规范时间戳.vi"("字符串"=w2292) -> ("result string"=w2294:string)  [unwired: 10 in]
                n1173 = Format Into String(format string="DataTime=%s;PolId=w01019,i12001-Info=%s,i12031-Info=%s;" ("格式字符串"), w2294, w2291, w2291) -> (resulting string=w2293:string)  [unwired: 2 in, 1 out]
              }
              frame True {
              }
            }
            n1174 = Concatenate Strings(w2264, w2263, w2262, w2259, w2258) -> (w2256:string)
          }
          frame "返回执行结果" {
            w2297 = 0 ("包数")
            n1175 = property on="总包数" class="DigNum (严格)"("Value"=w2297) -> ()  [unwired: 2 in, 2 out]
            n1176 = property on="包数" class="DigNum (严格)"("Value"=w2297) -> ()  [unwired: 2 in, 2 out]
          }
        }
        n1177 = global read "全局 数据数组大小.vi" "数据数组大小"() -> (w2206:i32)
        n1178 = global read "全局1.vi" "枚举"() -> (w2199:enum16{"返回请求应答", "上传数据", "返回执行结果"})
        n1179 = global read "全局1.vi" "枚举"() -> (w2203:enum16{"返回请求应答", "上传数据", "返回执行结果"})
        n1180 = Increment(x=w2197) -> (x+1=w2205:i32)
        n1181 = Equal?(x=w2199, y=enum16{"返回请求应答", "上传数据", "返回执行结果"}."返回执行结果") -> (x = y?=w2198:bool)
        n1182 = Equal?(x=w2203, y=enum16{"返回请求应答", "上传数据", "返回执行结果"}."返回请求应答") -> (x = y?=w2201:bool)
        n1183 = Greater Or Equal?(x=w2205, y=w2206) -> (x >= y?=w2204:bool)
        n1184 = Compound Arithmetic op=OR ("复合运算")(w2198, w2201, w2204) -> (w2174:bool)
        n1185 = call <vilib>:"Boolean Crossing PtByPt.vi"("direction"=enum16{"either", "false-true", "true-false"}."false-true", "input"=w2174) -> ("crossing"=w2175:bool)  [unwired: 1 in]
        n1186 = case shown="真" w2175 {
          frame False {
          }
          frame True {
            n1187 = property on="包数" class="DigNum (严格)"() -> ("Value"=w2226:i32)  [unwired: 2 in, 2 out]
            n1188 = Increment(x=w2226) -> (x+1=w2225:i32)
            n1189 = property on="总包数" class="DigNum (严格)"("Value"=w2225) -> ()  [unwired: 2 in, 2 out]
          }
        }
        n1190 = Concatenate Strings(w2172, w2171) -> (w2177:string)
        n1191 = String Length(string=w2177) -> (length=w2180:i32)
        n1192 = Greater Or Equal?(x=w2180, y=890) -> (x >= y?=w2178:bool)
        n1193 = case shown="真" w2178 {
          tunnel: w2177 -> [w2210 w2214]
          tunnel: [w2210 w2213] -> w2173
          tunnel: w2171 -> [_ w2215]
          frame False {
            n1194 = global read "全局 小时数据发送次数.vi" "小时数据发送次数"() -> (w2207:i32)
            n1195 = global read "全局 数据数组大小.vi" "数据数组大小"() -> (w2208:i32)
            n1196 = Equal?(x=w2207, y=w2208) -> (x = y?=w2209:bool)
            n1197 = case shown="真" w2209 {
              frame False {
              }
              frame True {
                n1198 = property on="包数" class="DigNum (严格)"() -> ("Value"=w2212:i32)  [unwired: 2 in, 2 out]
                n1199 = Increment(x=w2212) -> (x+1=w2211:i32)
                n1200 = property on="包数" class="DigNum (严格)"("Value"=w2211) -> ()  [unwired: 2 in, 2 out]
              }
            }
          }
          frame True {
            n1201 = global read "全局 小时数据发送次数.vi" "小时数据发送次数"() -> (w2217:i32)
            n1202 = global read "全局 数据数组大小.vi" "数据数组大小"() -> (w2216:i32)
            n1203 = property on="小时数据发送次数" class="DigNum (严格)"() -> ("Value"=w2221:i32)  [unwired: 2 in, 2 out]
            n1204 = Increment(x=w2221) -> (x+1=w2220:i32)
            n1205 = Equal?(x=w2217, y=w2216) -> (x = y?=w2218:bool)
            n1206 = case shown="假" w2218 {
              tunnel: w2215 -> [w2223 _]
              tunnel: [w2223 w2224] -> w2213
              tunnel: w2214 -> [_ w2224]
              frame False {
              }
              frame True {
              }
            }
            n1207 = property on="小时数据发送次数" class="DigNum (严格)"("Value"=w2220) -> ()  [unwired: 2 in, 2 out]
            n1208 = property on="包数" class="DigNum (严格)"() -> ("Value"=w2222:i32)  [unwired: 2 in, 2 out]
            n1209 = Increment(x=w2222) -> (x+1=w2219:i32)
            n1210 = property on="包数" class="DigNum (严格)"("Value"=w2219) -> ()  [unwired: 2 in, 2 out]
          }
        }
      }
      n1211 = global read "全局1.vi" "枚举"() -> (w2159:enum16{"返回请求应答", "上传数据", "返回执行结果"})
      n1212 = Equal?(x=w2159, y=enum16{"返回请求应答", "上传数据", "返回执行结果"}."上传数据") -> (x = y?=w2157:bool)
      n1213 = case shown="真" w2157 {
        tunnel: ["" w2169] -> w2156
        frame False {
        }
        frame True {
          n1214 = property on="总包数" class="DigNum (严格)"() -> ("Value"=w2170:i32)  [unwired: 2 in, 2 out]
          n1215 = Number To Decimal String(number=w2170) -> (decimal integer string=w2169:string)  [unwired: 1 in]
        }
      }
    }
    frame "系统状态" {
      n1216 = disable-structure shown="禁用" {
        disable-tunnel: [w2439 _] -> w2437
        frame Disabled {
          n1217 = Spreadsheet String To Array(delimiter (Tab)=" " ("分隔符(Tab)"), format string="" ("格式字符串"), array type (2D Dbl)=string[] []) -> (array=w2444:string[])  [unwired: 1 in]
          n1218 = Index Array(array=w2444, index #1=3 ("索引"), index #2=1 ("索引")) -> (element #1=w2442:string, element #2=w2440:string)
          n1219 = call "规范时间戳.vi"() -> ("result string"=w2438:string)  [unwired: 11 in]
          n1220 = Format Into String(format string="DataTime=%s;Volt=%s;Temp=%s;Hum=%s;Lng=%s;Lat=%s" ("格式字符串"), w2438, w2442, w2440) -> (resulting string=w2439:string)  [unwired: 5 in, 1 out]
        }
        frame Enabled {
        }
      }
    }
  }
  n1221 = case shown="假" w29 {
    tunnel: [w2450 w2454] -> w31
    frame False {
      n1222 = global read "全局1.vi" "枚举"() -> (w2449:enum16{"返回请求应答", "上传数据", "返回执行结果"})
      n1223 = case shown="\"上传数据\"" w2449 {
        tunnel: ["91" ("CN") "21" ("CN") "91" ("CN")] -> w2450
        frame "返回请求应答", Default {
        }
        frame "上传数据" {
        }
        frame "返回执行结果" {
        }
      }
    }
    frame True {
      n1224 = global read "全局 反控命令枚举.vi" "反控命令枚举"() -> (w2455:enum16{"返回请求应答", "返回执行结果"})
      n1225 = case shown="\"返回请求应答\", 默认" w2455 {
        tunnel: ["91" "91"] -> w2454
        frame "返回请求应答", Default {
        }
        frame "返回执行结果" {
        }
      }
    }
  }
  n1226 = Decimal String To Number(string=w14) -> (number=w23:i32)  [unwired: 2 in, 1 out]
  n1227 = Greater?(x=w23, y=1) -> (0:w2:bool)
  n1228 = case shown="\"报警信息\", \"操作日志\"" "table输入" {
    tunnel: ["9015" ("ST") w2468 w2476 w2484 w2495 w2509 w2518 w2539 w2550 w2560 w2570 "3020" ("ST")] -> w35
    tunnel: ["8" ("ST") "9" ("ST") "9" ("ST") "8" ("ST") "9" ("ST") w2512 w2523 w2537 w2549 w2559 "9" ("ST") "8" ("ST")] -> w34
    tunnel: w10 -> [_ w2466 w2474 w2485 w2496 w2511 w2522 w2541 w2552 w2563 w2572 w2578]
    tunnel: [_ w2466 w2474 w2485 w2496 w2511 w2522 w2541 w2552 w2563 w2572 w2578] -> w33
    tunnel: w2 -> [_ _ _ _ _ w2508 w2521 w2538 w2548 w2561 _ _]
    tunnel: [w2458 w2465 w2473 w2481 w2488 w2507 w2520 w2536 w2547 w2558 w2569 w2577] -> w1
    frame "心跳包", Default {
      # "心跳包"
      n1229 = Get Date/Time In Seconds() -> (seconds since 1Jan1904=w2461:timestamp)
      n1230 = Format Date/Time String(time format string (%c)="%Y%m%d%H%M%S%3u" ("时间格式字符串(%c)"), seconds (now)=w2461) -> (date/time string=w2460:string)  [unwired: 1 in]
      n1231 = Search and Replace String(input string=w2460, search string="." ("搜索字符串")) -> (result string=w2458:string)  [unwired: 6 in, 3 out]
    }
    frame "提取数采仪时间" {
      n1232 = global read "全局1.vi" "枚举"() -> (w2469:enum16{"返回请求应答", "上传数据", "返回执行结果"})
      n1233 = case shown="\"返回执行结果\"" w2469 {
        tunnel: ["9011" ("CN") "1014" ("CN") "9012" ("CN")] -> w2468
        frame "返回请求应答", Default {
        }
        frame "上传数据" {
        }
        frame "返回执行结果" {
        }
      }
      n1234 = local read "QN"() -> (w2465:string)
    }
    frame "提取实时数据间隔" {
      n1235 = global read "全局1.vi" "枚举"() -> (w2477:enum16{"返回请求应答", "上传数据", "返回执行结果"})
      n1236 = case shown="\"上传数据\"" w2477 {
        tunnel: ["9011" ("CN") "1061" ("CN") "9012" ("CN")] -> w2476
        frame "返回请求应答", Default {
        }
        frame "上传数据" {
        }
        frame "返回执行结果" {
        }
      }
      n1237 = local read "QN"() -> (w2473:string)
    }
    frame "反控命令" {
      n1238 = global read "全局 反控命令枚举.vi" "反控命令枚举"() -> (w2482:enum16{"返回请求应答", "返回执行结果"})
      n1239 = case shown="\"返回请求应答\", 默认" w2482 {
        tunnel: ["9011" ("CN") "9012" ("CN")] -> w2484
        frame "返回请求应答", Default {
        }
        frame "返回执行结果" {
        }
      }
      n1240 = local read "QN"() -> (w2481:string)
    }
    frame "实时数据" {
      n1241 = global read "全局1.vi" "枚举"() -> (w2494:enum16{"返回请求应答", "上传数据", "返回执行结果"})
      n1242 = case shown="\"上传数据\"" w2494 {
        tunnel: ["9011" ("CN") w2499 "9012" ("CN")] -> w2495
        frame "返回请求应答", Default {
        }
        frame "上传数据" {
          n1243 = global read "全局 实时数据参数.vi" "实时数据参数"() -> (w2498:string)
          n1244 = case shown="\"零点核查\"" w2498 {
            tunnel: ["2011" ("CN") "2064" ("CN") "2063" ("CN") "2065" ("CN") "2066" ("CN") "fff" ("CN")] -> w2499
            frame "水样测试", Default {
            }
            frame "平行样测试" {
            }
            frame "加标回收测试" {
            }
            frame "零点核查" {
            }
            frame "跨度核查" {
            }
            frame "" {
            }
          }
        }
        frame "返回执行结果" {
        }
      }
      n1245 = Get Date/Time In Seconds() -> (seconds since 1Jan1904=w2491:timestamp)
      n1246 = Format Date/Time String(time format string (%c)="%Y%m%d%H%M%S%3u" ("时间格式字符串(%c)"), seconds (now)=w2491) -> (date/time string=w2490:string)  [unwired: 1 in]
      n1247 = Search and Replace String(input string=w2490, search string="." ("搜索字符串")) -> (result string=w2488:string)  [unwired: 6 in, 3 out]
    }
    frame "小时数据" {
      # "监测小时数据"
      n1248 = global read "全局1.vi" "枚举"() -> (w2510:enum16{"返回请求应答", "上传数据", "返回执行结果"})
      n1249 = case shown="\"上传数据\"" w2510 {
        tunnel: ["9011" ("CN") "2061" ("CN") "9012" ("CN")] -> w2509
        frame "返回请求应答", Default {
        }
        frame "上传数据" {
        }
        frame "返回执行结果" {
        }
      }
      n1250 = case shown="假" w2508 {
        tunnel: ["9" ("ST") "11" ("ST")] -> w2512
        frame False {
        }
        frame True {
        }
      }
      n1251 = local read "QN"() -> (w2507:string)
    }
    frame "提取实时数据" {
      # "提取实时数据"
      n1252 = global read "全局1.vi" "枚举"() -> (w2519:enum16{"返回请求应答", "上传数据", "返回执行结果"})
      n1253 = case shown="\"上传数据\"" w2519 {
        tunnel: ["9011" ("CN") w2526 "9012" ("CN")] -> w2518
        frame "返回请求应答", Default {
        }
        frame "上传数据" {
          n1254 = global read "全局 实时数据参数.vi" "实时数据参数"() -> (w2525:string)
          n1255 = case shown="\"零点核查\"" w2525 {
            tunnel: ["2011" ("CN") "2064" ("CN") "2063" ("CN") "2065" ("CN") "2066" ("CN") "fff" ("CN")] -> w2526
            frame "水样测试", Default {
            }
            frame "平行样测试" {
            }
            frame "加标回收测试" {
            }
            frame "零点核查" {
            }
            frame "跨度核查" {
            }
            frame "" {
            }
          }
        }
        frame "返回执行结果" {
        }
      }
      n1256 = case shown="真" w2521 {
        tunnel: ["9" ("ST") "11" ("ST")] -> w2523
        frame False {
        }
        frame True {
        }
      }
      n1257 = local read "QN"() -> (w2520:string)
    }
    frame "跨度核查" {
      # "跨度核查"
      n1258 = global read "全局1.vi" "枚举"() -> (w2540:enum16{"返回请求应答", "上传数据", "返回执行结果"})
      n1259 = case shown="\"上传数据\"" w2540 {
        tunnel: ["9011" ("CN") "2066" ("ST") "9012" ("CN")] -> w2539
        frame "返回请求应答", Default {
        }
        frame "上传数据" {
        }
        frame "返回执行结果" {
        }
      }
      n1260 = case shown="假" w2538 {
        tunnel: ["9" ("ST") "11" ("ST")] -> w2537
        frame False {
        }
        frame True {
        }
      }
      n1261 = local read "QN"() -> (w2536:string)
    }
    frame "零点核查" {
      # "零点核查"
      n1262 = global read "全局1.vi" "枚举"() -> (w2551:enum16{"返回请求应答", "上传数据", "返回执行结果"})
      n1263 = case shown="\"上传数据\"" w2551 {
        tunnel: ["9011" ("CN") "2065" ("ST") "9012" ("CN")] -> w2550
        frame "返回请求应答", Default {
        }
        frame "上传数据" {
        }
        frame "返回执行结果" {
        }
      }
      n1264 = case shown="假" w2548 {
        tunnel: ["9" ("ST") "11" ("ST")] -> w2549
        frame False {
        }
        frame True {
        }
      }
      n1265 = local read "QN"() -> (w2547:string)
    }
    frame "核查数据" {
      # "核查数据"
      n1266 = global read "全局1.vi" "枚举"() -> (w2562:enum16{"返回请求应答", "上传数据", "返回执行结果"})
      n1267 = case shown="\"上传数据\"" w2562 {
        tunnel: ["9011" ("CN") "2066" ("ST") "9012" ("CN")] -> w2560
        frame "返回请求应答", Default {
        }
        frame "上传数据" {
        }
        frame "返回执行结果" {
        }
      }
      n1268 = case shown="假" w2561 {
        tunnel: ["9" ("ST") "11" ("ST")] -> w2559
        frame False {
        }
        frame True {
        }
      }
      n1269 = local read "QN"() -> (w2558:string)
    }
    frame "报警信息", "操作日志" {
      n1270 = global read "全局1.vi" "枚举"() -> (w2571:enum16{"返回请求应答", "上传数据", "返回执行结果"})
      n1271 = case shown="\"上传数据\"" w2571 {
        tunnel: ["9011" ("CN") "3020" ("CN") "9012" ("CN")] -> w2570
        frame "返回请求应答", Default {
        }
        frame "上传数据" {
        }
        frame "返回执行结果" {
        }
      }
      n1272 = local read "QN"() -> (w2569:string)
    }
    frame "系统状态" {
      n1273 = local read "QN"() -> (w2577:string)
    }
  }
  n1274 = case shown="真" w2 {
    tunnel: [w2581 w2583] -> w21
    tunnel: w14 -> [_ w2582]
    tunnel: [w2581 w2582] -> w13
    frame False {
      w2581 = ""
    }
    frame True {
      n1275 = property on="当前包数" class="DigNum (严格)"() -> ("Value"=w2584:i32)  [unwired: 2 in, 2 out]
      n1276 = Number To Decimal String(number=w2584) -> (decimal integer string=w2583:string)  [unwired: 1 in]
    }
  }
  n1277 = Bundle By Name(cluster="数据块", "ST"=w31, "CN"=w35, "FLAG"=w34, "CP"=w33, "QN"=w1, "MN"="MN", "PW"="PW", "PNUM"=w13, "PNO"=w21) -> (w32:T1)
  n1278 = call "HJ212-2017.vi"("数据段"=w32) -> ("通讯包字符串"=w39:string, "通讯包"=→"通讯包":T2)  [unwired: 8 in, 1 out]
  "通讯包字符串" <- w39
  n1279 = String Length(string=w39) -> (length=→"长度":i32)
  "错误常量" <- "错误常量 2"
  "小时数据发送次数" <- 0 ("小时数据发送次数")
  "核查数据发送次数" <- 0 ("核查数据发送次数")
